vi "Wavefront analysis Final.vi"() -> ()   [LabVIEW 2020]
uses:
  <vilib>/Utility/file.llb/Read Delimited Spreadsheet (DBL).vi
  <vilib>/Analysis/NI_AALPro.lvlib
  <vilib>/Analysis/2dsp.llb/2D Real FFT.vi
  <vilib>/Analysis/2dsp.llb/2D Inverse Real FFT.vi
panel:
  in  "Reference images":T1(tab)
  out "Idler ref":dbl[][](graph)=[[0.0, 0.0, 0.0, 0.0, 0.0, 0.0, 0.0, 0.0, 0.0, 0.0, 0.0, 0.0, 0.0, 0.0, 0.0, 0.0, 0.0, 0.0, 33.0, 33.0, 33.0, 38.0, 30.0, 41.0, 34.0, 38.0, 29.0, 26.0, 34.0, 37.0, 34.0, 39.0, 41.0, 39.0, 28.0, 51.0, 29.0, 46.0, 35.0, 0.0, 0.0, 0.0, 0.0, 0.0, 0.0, 0.0, 0.0, 0.0, 0.0, 0.0, 0.0, 0.0, 0.0, 0.0, 0.0, 0.0, 0.0, 0.0], [0.0, 0.0, 0.0, 0.0, 0.0, 0.0, 0.0, 0.0, 0.0, 0.0, 0.0, 0.0, 0.0, 0.0, 0.0, 29.0, 23.0, 38.0, 37.0, 31.0, 35.0, 38.0, 33.0, 31.0, 43.0, 36.0, 24.0, 41.0, 38.0, 33.0, 48.0, 34.0, 27.0, 37.0, 37.0, 47.0, 27.0, 30.0, 24.0, 36.0, 28.0, 40.0, 0.0, 0.0, 0.0, 0.0, 0.0, 0.0, 0.0, 0.0, 0.0, 0.0, 0.0, 0.0, 0.0, 0.0, 0.0, 0.0], [0.0, 0.0, 0.0, 0.0, 0.0, 0.0, 0.0, 0.0, 0.0, 0.0, 0.0, 0.0, 0.0, 0.0, 24.0, 28.0, 30.0, 32.0, 21.0, 38.0, 33.0, 37.0, 36.0, 39.0, 36.0, 20.0, 48.0, 45.0, 50.0, 36.0, 30.0, 33.0, 44.0, 34.0, 31.0, 41.0, 34.0, 34.0, 26.0, 38.0, 38.0, 33.0, 28.0, 0.0, 0.0, 0.0, 0.0, 0.0, 0.0, 0.0, 0.0, 0.0, 0.0, 0.0, 0.0, 0.0, 0.0, 0.0], [0.0, 0.0, 0.0, 0.0, 0.0, 0.0, 0.0, 0.0, 0.0, 0.0, 0.0, 0.0, 36.0, 33.0, 26.0, 25.0, 35.0, 38.0, 37.0, 24.0, 35.0, 37.0, 34.0, 35.0, 34.0, 35.0, 42.0, 33.0, 36.0, 33.0, 53.0, 50.0, 40.0, 36.0, 45.0, 27.0, 36.0, 44.0, 23.0, 29.0, 23.0, 31.0, 26.0, 22.0, 27.0, 0.0, 0.0, 0.0, 0.0, 0.0, 0.0, 0.0, 0.0, 0.0, 0.0, 0.0, 0.0, 0.0], [0.0, 0.0, 0.0, 0.0, 0.0, 0.0, 0.0, 0.0, 0.0, 0.0, 0.0, 27.0, 31.0, 42.0, 27.0, 39.0, 33.0, 23.0, 26.0, 41.0, 28.0, 46.0, 34.0, 36.0, 36.0, 37.0, 37.0, 51.0, 39.0, 51.0, 38.0, 40.0, 32.0, 43.0, 30.0, 48.0, 29.0, 27.0, 31.0, 50.0, 35.0, 31.0, 23.0, 18.0, 27.0, 26.0, 0.0, 0.0, 0.0, 0.0, 0.0, 0.0, 0.0, 0.0, 0.0, 0.0, 0.0, 0.0], [0.0, 0.0, 0.0, 0.0, 0.0, 0.0, 0.0, 0.0, 0.0, 26.0, 28.0, 24.0, 30.0, 32.0, 29.0, 36.0, 28.0, 42.0, 34.0, 34.0, 43.0, 42.0, 35.0, 40.0, 24.0, 47.0, 35.0, 40.0, 41.0, 44.0, 46.0, 46.0, 40.0, 33.0, 42.0, 38.0, 30.0, 35.0, 29.0, 30.0, 24.0, 42.0, 40.0, 27.0, 29.0, 36.0, 26.0, 60.0, 0.0, 0.0, 0.0, 0.0, 0.0, 0.0, 0.0, 0.0, 0.0, 0.0], [0.0, 0.0, 0.0, 0.0, 0.0, 0.0, 0.0, 0.0, 30.0, 36.0, 36.0, 25.0, 30.0, 38.0, 31.0, 37.0, 36.0, 30.0, 25.0, 34.0, 55.0, 21.0, 38.0, 55.0, 42.0, 46.0, 34.0, 53.0, 43.0, 36.0, 41.0, 44.0, 40.0, 35.0, 42.0, 42.0, 27.0, 38.0, 40.0, 40.0, 41.0, 35.0, 31.0, 37.0, 30.0, 36.0, 39.0, 38.0, 25.0, 0.0, 0.0, 0.0, 0.0, 0.0, 0.0, 0.0, 0.0, 0.0], [0.0, 0.0, 0.0, 0.0, 0.0, 0.0, 0.0, 32.0, 34.0, 29.0, 26.0, 28.0, 35.0, 32.0, 27.0, 32.0, 35.0, 40.0, 43.0, 41.0, 29.0, 52.0, 41.0, 55.0, 34.0, 45.0, 44.0, 53.0, 55.0, 45.0, 41.0, 50.0, 47.0, 49.0, 41.0, 53.0, 57.0, 39.0, 43.0, 51.0, 30.0, 45.0, 32.0, 32.0, 28.0, 39.0, 31.0, 39.0, 38.0, 29.0, 0.0, 0.0, 0.0, 0.0, 0.0, 0.0, 0.0, 0.0], [0.0, 0.0, 0.0, 0.0, 0.0, 0.0, 24.0, 28.0, 14.0, 26.0, 35.0, 26.0, 43.0, 27.0, 40.0, 51.0, 25.0, 39.0, 40.0, 35.0, 39.0, 43.0, 43.0, 63.0, 50.0, 55.0, 64.0, 56.0, 55.0, 58.0, 62.0, 49.0, 50.0, 53.0, 40.0, 53.0, 40.0, 32.0, 47.0, 48.0, 40.0, 31.0, 33.0, 41.0, 37.0, 41.0, 35.0, 38.0, 22.0, 43.0, 25.0, 0.0, 0.0, 0.0, 0.0, 0.0, 0.0, 0.0], [0.0, 0.0, 0.0, 0.0, 0.0, 30.0, 23.0, 38.0, 28.0, 28.0, 21.0, 17.0, 39.0, 32.0, 25.0, 30.0, 39.0, 43.0, 39.0, 40.0, 36.0, 49.0, 65.0, 63.0, 68.0, 68.0, 91.0, 134.0, 191.0, 218.0, 213.0, 162.0, 141.0, 99.0, 74.0, 61.0, 57.0, 50.0, 46.0, 43.0, 39.0, 44.0, 31.0, 41.0, 31.0, 31.0, 39.0, 39.0, 25.0, 47.0, 30.0, 39.0, 0.0, 0.0, 0.0, 0.0, 0.0, 0.0], [0.0, 0.0, 0.0, 0.0, 0.0, 25.0, 34.0, 32.0, 30.0, 30.0, 33.0, 38.0, 20.0, 38.0, 36.0, 38.0, 38.0, 37.0, 50.0, 56.0, 67.0, 82.0, 95.0, 151.0, 229.0, 345.0, 495.0, 498.0, 427.0, 526.0, 467.0, 540.0, 425.0, 358.0, 282.0, 162.0, 126.0, 88.0, 41.0, 56.0, 54.0, 29.0, 38.0, 24.0, 29.0, 41.0, 25.0, 34.0, 38.0, 37.0, 32.0, 28.0, 0.0, 0.0, 0.0, 0.0, 0.0, 0.0], [0.0, 0.0, 0.0, 0.0, 33.0, 23.0, 29.0, 28.0, 21.0, 34.0, 21.0, 31.0, 28.0, 32.0, 38.0, 48.0, 24.0, 44.0, 53.0, 80.0, 88.0, 241.0, 416.0, 503.0, 578.0, 542.0, 550.0, 501.0, 622.0, 490.0, 555.0, 528.0, 521.0, 522.0, 551.0, 513.0, 396.0, 306.0, 163.0, 65.0, 58.0, 47.0, 45.0, 36.0, 49.0, 37.0, 40.0, 21.0, 28.0, 43.0, 42.0, 29.0, 39.0, 0.0, 0.0, 0.0, 0.0, 0.0], [0.0, 0.0, 0.0, 26.0, 22.0, 31.0, 26.0, 26.0, 29.0, 21.0, 33.0, 39.0, 34.0, 32.0, 40.0, 54.0, 44.0, 50.0, 84.0, 130.0, 319.0, 562.0, 595.0, 590.0, 484.0, 448.0, 430.0, 508.0, 426.0, 495.0, 370.0, 486.0, 414.0, 422.0, 449.0, 546.0, 539.0, 454.0, 378.0, 228.0, 88.0, 48.0, 35.0, 46.0, 27.0, 38.0, 30.0, 45.0, 34.0, 31.0, 35.0, 26.0, 42.0, 27.0, 0.0, 0.0, 0.0, 0.0], [0.0, 0.0, 0.0, 28.0, 28.0, 24.0, 30.0, 21.0, 29.0, 30.0, 37.0, 28.0, 41.0, 47.0, 32.0, 40.0, 69.0, 72.0, 195.0, 471.0, 613.0, 548.0, 436.0, 452.0, 459.0, 526.0, 488.0, 652.0, 721.0, 779.0, 685.0, 563.0, 529.0, 568.0, 425.0, 399.0, 408.0, 519.0, 486.0, 494.0, 295.0, 138.0, 54.0, 59.0, 44.0, 40.0, 36.0, 35.0, 34.0, 36.0, 30.0, 26.0, 20.0, 37.0, 0.0, 0.0, 0.0, 0.0], [0.0, 0.0, 24.0, 26.0, 32.0, 27.0, 27.0, 34.0, 19.0, 40.0, 35.0, 33.0, 35.0, 33.0, 55.0, 71.0, 90.0, 231.0, 518.0, 543.0, 543.0, 410.0, 519.0, 562.0, 791.0, 1009.0, 1198.0, 1635.0, 1601.0, 1726.0, 1566.0, 1517.0, 1198.0, 1037.0, 729.0, 515.0, 464.0, 430.0, 429.0, 503.0, 406.0, 338.0, 122.0, 51.0, 36.0, 41.0, 39.0, 42.0, 44.0, 36.0, 26.0, 33.0, 21.0, 32.0, 35.0, 0.0, 0.0, 0.0], [0.0, 21.0, 22.0, 24.0, 27.0, 27.0, 27.0, 23.0, 26.0, 29.0, 17.0, 42.0, 42.0, 46.0, 52.0, 106.0, 346.0, 509.0, 575.0, 535.0, 497.0, 567.0, 866.0, 1318.0, 1774.0, 2119.0, 2964.0, 3113.0, 3455.0, 3111.0, 3488.0, 3069.0, 2628.0, 2285.0, 1622.0, 1099.0, 710.0, 556.0, 435.0, 484.0, 498.0, 519.0, 371.0, 150.0, 59.0, 55.0, 36.0, 36.0, 35.0, 31.0, 41.0, 39.0, 30.0, 30.0, 26.0, 33.0, 0.0, 0.0], [0.0, 32.0, 24.0, 27.0, 25.0, 21.0, 32.0, 31.0, 36.0, 25.0, 45.0, 44.0, 58.0, 64.0, 65.0, 377.0, 581.0, 632.0, 457.0, 563.0, 675.0, 1158.0, 1641.0, 2438.0, 3581.0, 4509.0, 4776.0, 5330.0, 5944.0, 6860.0, 6038.0, 5448.0, 4841.0, 3697.0, 3073.0, 2359.0, 1544.0, 971.0, 576.0, 432.0, 386.0, 564.0, 475.0, 342.0, 118.0, 59.0, 45.0, 35.0, 43.0, 44.0, 32.0, 37.0, 43.0, 36.0, 27.0, 26.0, 0.0, 0.0], [0.0, 23.0, 16.0, 31.0, 22.0, 30.0, 32.0, 31.0, 35.0, 38.0, 40.0, 41.0, 52.0, 74.0, 176.0, 530.0, 531.0, 542.0, 517.0, 741.0, 1312.0, 1994.0, 3477.0, 4643.0, 5314.0, 6802.0, 7334.0, 7358.0, 8098.0, 7575.0, 8057.0, 7131.0, 6266.0, 6447.0, 4971.0, 4459.0, 2925.0, 2009.0, 1242.0, 643.0, 485.0, 441.0, 476.0, 478.0, 230.0, 121.0, 43.0, 35.0, 47.0, 37.0, 34.0, 26.0, 30.0, 43.0, 35.0, 38.0, 0.0, 0.0], [22.0, 14.0, 27.0, 31.0, 29.0, 36.0, 22.0, 29.0, 30.0, 32.0, 33.0, 37.0, 56.0, 104.0, 425.0, 632.0, 524.0, 490.0, 697.0, 1430.0, 2375.0, 3795.0, 4959.0, 7130.0, 7177.0, 7810.0, 8567.0, 10207.0, 9049.0, 9189.0, 8739.0, 9440.0, 8494.0, 7912.0, 7186.0, 5411.0, 4928.0, 3224.0, 2005.0, 1126.0, 613.0, 437.0, 411.0, 580.0, 384.0, 187.0, 76.0, 46.0, 32.0, 35.0, 42.0, 36.0, 33.0, 29.0, 23.0, 30.0, 26.0, 0.0], [20.0, 24.0, 22.0, 19.0, 30.0, 24.0, 32.0, 40.0, 41.0, 42.0, 40.0, 52.0, 68.0, 232.0, 602.0, 525.0, 564.0, 695.0, 1240.0, 2185.0, 3656.0, 5311.0, 4998.0, 9311.0, 9246.0, 11117.0, 9926.0, 10643.0, 9993.0, 10412.0, 10979.0, 10696.0, 10376.0, 9054.0, 8507.0, 7575.0, 5940.0, 4773.0, 3361.0, 1780.0, 1166.0, 531.0, 411.0, 468.0, 491.0, 311.0, 113.0, 56.0, 40.0, 39.0, 26.0, 35.0, 31.0, 34.0, 29.0, 26.0, 33.0, 0.0], [24.0, 23.0, 25.0, 31.0, 36.0, 20.0, 41.0, 28.0, 47.0, 25.0, 38.0, 71.0, 119.0, 408.0, 589.0, 505.0, 529.0, 1018.0, 2193.0, 3424.0, 5249.0, 6870.0, 12486.0, 7988.0, 10335.0, 10971.0, 11179.0, 10325.0, 11253.0, 11504.0, 10668.0, 9355.0, 12095.0, 9948.0, 10038.0, 9773.0, 8219.0, 6509.0, 4643.0, 3116.0, 1708.0, 893.0, 415.0, 381.0, 491.0, 398.0, 157.0, 68.0, 43.0, 43.0, 34.0, 34.0, 27.0, 24.0, 26.0, 40.0, 29.0, 0.0], [25.0, 31.0, 29.0, 24.0, 25.0, 21.0, 29.0, 30.0, 36.0, 32.0, 57.0, 71.0, 172.0, 601.0, 502.0, 557.0, 739.0, 1605.0, 2981.0, 4696.0, 6564.0, 7940.0, 9108.0, 9805.0, 12772.0, 10382.0, 10614.0, 11851.0, 11619.0, 9702.0, 11860.0, 11185.0, 12321.0, 10842.0, 11020.0, 9818.0, 8451.0, 8122.0, 5936.0, 4325.0, 2629.0, 1259.0, 627.0, 413.0, 407.0, 538.0, 227.0, 107.0, 49.0, 33.0, 39.0, 35.0, 26.0, 33.0, 31.0, 43.0, 21.0, 32.0], [28.0, 27.0, 31.0, 31.0, 21.0, 35.0, 25.0, 32.0, 21.0, 42.0, 61.0, 95.0, 378.0, 589.0, 538.0, 547.0, 975.0, 2235.0, 3482.0, 6571.0, 8268.0, 9056.0, 11003.0, 11631.0, 10641.0, 11928.0, 10949.0, 10324.0, 10096.0, 11159.0, 10977.0, 10308.0, 10593.0, 10623.0, 10514.0, 11646.0, 9405.0, 9366.0, 7021.0, 5020.0, 3319.0, 1720.0, 806.0, 455.0, 421.0, 467.0, 345.0, 132.0, 54.0, 34.0, 37.0, 37.0, 34.0, 27.0, 33.0, 20.0, 37.0, 34.0], [19.0, 18.0, 18.0, 23.0, 27.0, 34.0, 28.0, 31.0, 50.0, 42.0, 65.0, 182.0, 477.0, 528.0, 524.0, 691.0, 1719.0, 2864.0, 5291.0, 6825.0, 8333.0, 11756.0, 10344.0, 10804.0, 11046.0, 11765.0, 10495.0, 9731.0, 10459.0, 9842.0, 9930.0, 11113.0, 10964.0, 10430.0, 11969.0, 10333.0, 10266.0, 9385.0, 8245.0, 6496.0, 4192.0, 2630.0, 1143.0, 511.0, 400.0, 488.0, 448.0, 150.0, 70.0, 64.0, 42.0, 47.0, 34.0, 28.0, 33.0, 40.0, 13.0, 29.0], [21.0, 21.0, 24.0, 24.0, 27.0, 29.0, 24.0, 29.0, 46.0, 60.0, 76.0, 211.0, 501.0, 550.0, 555.0, 854.0, 1737.0, 3504.0, 6034.0, 8184.0, 8996.0, 11258.0, 10863.0, 12142.0, 11259.0, 10331.0, 10193.0, 9997.0, 10594.0, 8854.0, 10112.0, 9586.0, 10297.0, 11180.0, 10510.0, 10948.0, 10675.0, 10412.0, 8729.0, 6607.0, 5134.0, 3360.0, 1427.0, 586.0, 372.0, 479.0, 399.0, 286.0, 89.0, 51.0, 29.0, 30.0, 37.0, 32.0, 22.0, 31.0, 26.0, 37.0], [25.0, 27.0, 34.0, 27.0, 24.0, 28.0, 24.0, 36.0, 30.0, 53.0, 85.0, 319.0, 584.0, 600.0, 481.0, 1091.0, 2479.0, 4389.0, 6310.0, 9581.0, 9832.0, 10928.0, 11595.0, 11202.0, 11015.0, 10084.0, 9684.0, 9403.0, 7350.0, 9729.0, 8597.0, 10018.0, 9495.0, 10362.0, 10919.0, 10975.0, 10297.0, 10217.0, 9438.0, 7555.0, 5604.0, 3235.0, 1775.0, 800.0, 424.0, 481.0, 434.0, 294.0, 121.0, 48.0, 34.0, 37.0, 26.0, 35.0, 36.0, 25.0, 36.0, 33.0], [29.0, 21.0, 18.0, 24.0, 35.0, 21.0, 25.0, 37.0, 45.0, 52.0, 87.0, 334.0, 584.0, 473.0, 565.0, 1252.0, 2463.0, 4773.0, 6636.0, 8697.0, 11429.0, 10731.0, 10391.0, 11230.0, 10171.0, 9829.0, 9358.0, 9183.0, 9445.0, 8181.0, 9165.0, 8709.0, 8839.0, 10359.0, 10801.0, 9836.0, 10995.0, 10816.0, 10069.0, 7534.0, 5988.0, 3951.0, 1933.0, 952.0, 401.0, 448.0, 450.0, 343.0, 99.0, 57.0, 42.0, 36.0, 36.0, 38.0, 38.0, 37.0, 22.0, 40.0], [33.0, 35.0, 24.0, 27.0, 24.0, 26.0, 32.0, 30.0, 42.0, 65.0, 71.0, 328.0, 607.0, 516.0, 605.0, 1220.0, 2764.0, 5060.0, 7173.0, 9574.0, 9796.0, 11663.0, 10720.0, 12846.0, 9527.0, 10609.0, 8504.0, 9578.0, 8651.0, 8801.0, 7431.0, 8853.0, 9445.0, 9729.0, 10227.0, 11834.0, 10672.0, 10151.0, 9726.0, 8997.0, 6241.0, 4204.0, 2261.0, 870.0, 495.0, 443.0, 510.0, 339.0, 103.0, 64.0, 34.0, 33.0, 25.0, 41.0, 21.0, 21.0, 22.0, 31.0], [18.0, 23.0, 26.0, 26.0, 26.0, 42.0, 29.0, 42.0, 40.0, 57.0, 79.0, 370.0, 532.0, 574.0, 568.0, 1438.0, 2860.0, 5302.0, 7498.0, 9651.0, 9680.0, 11035.0, 11621.0, 10274.0, 9812.0, 10930.0, 8870.0, 9508.0, 7597.0, 8953.0, 8701.0, 9464.0, 8784.0, 10769.0, 9489.0, 11215.0, 10422.0, 10977.0, 8756.0, 8755.0, 5647.0, 4844.0, 2058.0, 1048.0, 428.0, 413.0, 465.0, 364.0, 127.0, 56.0, 38.0, 32.0, 32.0, 26.0, 26.0, 28.0, 26.0, 33.0], [22.0, 17.0, 26.0, 31.0, 26.0, 25.0, 23.0, 24.0, 35.0, 58.0, 99.0, 316.0, 630.0, 597.0, 550.0, 1361.0, 2643.0, 4687.0, 6930.0, 8844.0, 9908.0, 11137.0, 10461.0, 12016.0, 11124.0, 8758.0, 9497.0, 8959.0, 8403.0, 8907.0, 7968.0, 9479.0, 7817.0, 11878.0, 10209.0, 11642.0, 10825.0, 10586.0, 9688.0, 8819.0, 6405.0, 4123.0, 2208.0, 951.0, 432.0, 510.0, 416.0, 317.0, 98.0, 47.0, 30.0, 36.0, 34.0, 27.0, 30.0, 27.0, 28.0, 34.0], [20.0, 20.0, 31.0, 13.0, 23.0, 26.0, 38.0, 41.0, 43.0, 51.0, 59.0, 372.0, 566.0, 550.0, 547.0, 1163.0, 2273.0, 4811.0, 6481.0, 9604.0, 10290.0, 11230.0, 10872.0, 10070.0, 10565.0, 10873.0, 9490.0, 9608.0, 8858.0, 8698.0, 9740.0, 9255.0, 9585.0, 10318.0, 10549.0, 10201.0, 10721.0, 11495.0, 8466.0, 8079.0, 5681.0, 4016.0, 2129.0, 962.0, 427.0, 445.0, 393.0, 332.0, 116.0, 55.0, 32.0, 41.0, 30.0, 34.0, 34.0, 33.0, 27.0, 27.0], [16.0, 38.0, 26.0, 34.0, 22.0, 38.0, 27.0, 27.0, 44.0, 59.0, 66.0, 324.0, 585.0, 605.0, 505.0, 1057.0, 2197.0, 4221.0, 5855.0, 8610.0, 9564.0, 11505.0, 9789.0, 12674.0, 9997.0, 11264.0, 9528.0, 10363.0, 9151.0, 9507.0, 8605.0, 10215.0, 10311.0, 10253.0, 10901.0, 12845.0, 10351.0, 10239.0, 9807.0, 7870.0, 5582.0, 3329.0, 1717.0, 853.0, 371.0, 460.0, 440.0, 288.0, 102.0, 43.0, 34.0, 30.0, 41.0, 33.0, 19.0, 23.0, 27.0, 30.0], [16.0, 15.0, 12.0, 18.0, 32.0, 30.0, 18.0, 29.0, 48.0, 50.0, 68.0, 235.0, 544.0, 581.0, 577.0, 892.0, 1622.0, 3969.0, 6014.0, 7901.0, 9519.0, 11253.0, 10036.0, 12070.0, 10805.0, 10642.0, 10593.0, 10784.0, 9506.0, 11212.0, 9785.0, 11127.0, 10100.0, 12230.0, 10694.0, 10737.0, 12054.0, 11072.0, 8620.0, 7469.0, 4757.0, 3066.0, 1367.0, 495.0, 428.0, 498.0, 377.0, 256.0, 76.0, 53.0, 35.0, 30.0, 33.0, 37.0, 23.0, 44.0, 27.0, 31.0], [24.0, 31.0, 27.0, 15.0, 21.0, 30.0, 30.0, 36.0, 31.0, 49.0, 55.0, 145.0, 504.0, 573.0, 495.0, 620.0, 1607.0, 2733.0, 4655.0, 7794.0, 7507.0, 10585.0, 11470.0, 10295.0, 11512.0, 11444.0, 11207.0, 10982.0, 10269.0, 11393.0, 9225.0, 11186.0, 10890.0, 10763.0, 11164.0, 11732.0, 10195.0, 9714.0, 7731.0, 6073.0, 3965.0, 2203.0, 963.0, 560.0, 388.0, 443.0, 362.0, 245.0, 78.0, 54.0, 41.0, 25.0, 27.0, 36.0, 27.0, 22.0, 19.0, 24.0], [17.0, 23.0, 22.0, 27.0, 23.0, 25.0, 28.0, 27.0, 37.0, 59.0, 52.0, 86.0, 369.0, 616.0, 524.0, 613.0, 922.0, 2172.0, 3677.0, 5932.0, 8236.0, 9587.0, 10519.0, 11994.0, 11385.0, 12455.0, 11490.0, 11569.0, 9786.0, 12618.0, 10807.0, 11378.0, 10102.0, 11687.0, 11262.0, 11813.0, 9709.0, 9646.0, 6898.0, 5553.0, 3092.0, 1903.0, 712.0, 463.0, 401.0, 514.0, 366.0, 107.0, 61.0, 45.0, 31.0, 25.0, 19.0, 23.0, 24.0, 30.0, 32.0, 31.0], [35.0, 20.0, 25.0, 23.0, 25.0, 24.0, 28.0, 25.0, 38.0, 50.0, 59.0, 73.0, 172.0, 520.0, 567.0, 524.0, 809.0, 1769.0, 2680.0, 4518.0, 6192.0, 8250.0, 9723.0, 10511.0, 9553.0, 10974.0, 11124.0, 11651.0, 11831.0, 10824.0, 10850.0, 10868.0, 10452.0, 12044.0, 10795.0, 9860.0, 8964.0, 7809.0, 5547.0, 4172.0, 2266.0, 1037.0, 501.0, 427.0, 452.0, 473.0, 207.0, 97.0, 38.0, 35.0, 40.0, 41.0, 26.0, 38.0, 32.0, 23.0, 20.0, 29.0], [24.0, 25.0, 20.0, 28.0, 26.0, 23.0, 37.0, 36.0, 37.0, 39.0, 64.0, 63.0, 104.0, 418.0, 611.0, 593.0, 561.0, 1071.0, 1871.0, 4080.0, 4588.0, 7458.0, 7802.0, 9977.0, 10579.0, 10430.0, 10760.0, 11288.0, 10234.0, 12567.0, 10198.0, 11758.0, 10670.0, 11137.0, 9421.0, 9271.0, 7021.0, 6943.0, 3874.0, 2970.0, 1411.0, 812.0, 352.0, 444.0, 456.0, 394.0, 165.0, 59.0, 37.0, 30.0, 22.0, 31.0, 28.0, 27.0, 29.0, 28.0, 26.0, 0.0], [21.0, 24.0, 24.0, 25.0, 28.0, 29.0, 25.0, 44.0, 52.0, 45.0, 64.0, 76.0, 99.0, 215.0, 567.0, 577.0, 493.0, 697.0, 1111.0, 2039.0, 3142.0, 5007.0, 5918.0, 8639.0, 7955.0, 10544.0, 9986.0, 10767.0, 10437.0, 10532.0, 9905.0, 10126.0, 9204.0, 9729.0, 8888.0, 7806.0, 5715.0, 5184.0, 3167.0, 1756.0, 788.0, 560.0, 399.0, 480.0, 498.0, 250.0, 83.0, 56.0, 26.0, 34.0, 23.0, 29.0, 18.0, 27.0, 24.0, 27.0, 30.0, 0.0], [26.0, 22.0, 23.0, 23.0, 29.0, 34.0, 34.0, 46.0, 37.0, 48.0, 46.0, 74.0, 72.0, 128.0, 392.0, 639.0, 595.0, 512.0, 661.0, 1409.0, 2136.0, 3870.0, 4979.0, 5905.0, 6955.0, 8199.0, 8335.0, 8836.0, 8999.0, 9055.0, 8382.0, 9320.0, 8041.0, 8419.0, 6068.0, 5857.0, 4121.0, 2936.0, 1819.0, 994.0, 519.0, 404.0, 419.0, 507.0, 343.0, 164.0, 51.0, 55.0, 37.0, 29.0, 27.0, 20.0, 27.0, 22.0, 19.0, 24.0, 23.0, 0.0], [0.0, 22.0, 32.0, 27.0, 29.0, 33.0, 51.0, 25.0, 56.0, 48.0, 50.0, 63.0, 66.0, 102.0, 178.0, 575.0, 615.0, 596.0, 546.0, 708.0, 1087.0, 1959.0, 2831.0, 4292.0, 4826.0, 5620.0, 6566.0, 7177.0, 7116.0, 7486.0, 7108.0, 6801.0, 6665.0, 5350.0, 4676.0, 4161.0, 2937.0, 1656.0, 958.0, 611.0, 447.0, 466.0, 490.0, 468.0, 210.0, 88.0, 41.0, 49.0, 33.0, 43.0, 25.0, 35.0, 36.0, 26.0, 18.0, 21.0, 0.0, 0.0], [0.0, 20.0, 31.0, 31.0, 27.0, 34.0, 39.0, 57.0, 67.0, 56.0, 56.0, 60.0, 43.0, 73.0, 100.0, 256.0, 550.0, 593.0, 507.0, 507.0, 711.0, 1045.0, 1493.0, 2398.0, 2932.0, 4019.0, 4055.0, 5382.0, 4901.0, 5001.0, 5674.0, 5081.0, 3871.0, 4132.0, 2946.0, 1977.0, 1153.0, 918.0, 458.0, 391.0, 442.0, 540.0, 456.0, 291.0, 145.0, 59.0, 32.0, 35.0, 36.0, 35.0, 26.0, 22.0, 29.0, 19.0, 28.0, 28.0, 0.0, 0.0], [0.0, 28.0, 27.0, 32.0, 36.0, 34.0, 44.0, 41.0, 48.0, 58.0, 66.0, 55.0, 55.0, 54.0, 91.0, 102.0, 250.0, 571.0, 552.0, 494.0, 500.0, 556.0, 685.0, 1115.0, 1507.0, 2296.0, 2160.0, 3075.0, 2945.0, 3083.0, 2646.0, 2552.0, 2134.0, 2121.0, 1312.0, 1011.0, 629.0, 500.0, 395.0, 525.0, 514.0, 517.0, 306.0, 128.0, 63.0, 48.0, 28.0, 29.0, 22.0, 31.0, 25.0, 25.0, 19.0, 35.0, 23.0, 28.0, 0.0, 0.0], [0.0, 0.0, 38.0, 29.0, 31.0, 41.0, 43.0, 47.0, 41.0, 55.0, 64.0, 52.0, 66.0, 61.0, 70.0, 82.0, 146.0, 261.0, 506.0, 681.0, 570.0, 516.0, 465.0, 629.0, 707.0, 810.0, 1030.0, 1195.0, 1313.0, 1485.0, 1376.0, 1280.0, 1040.0, 835.0, 578.0, 487.0, 389.0, 416.0, 520.0, 504.0, 444.0, 273.0, 105.0, 82.0, 33.0, 36.0, 37.0, 36.0, 32.0, 20.0, 26.0, 36.0, 17.0, 26.0, 19.0, 0.0, 0.0, 0.0], [0.0, 0.0, 0.0, 40.0, 42.0, 35.0, 46.0, 41.0, 36.0, 56.0, 54.0, 63.0, 61.0, 50.0, 74.0, 75.0, 82.0, 107.0, 207.0, 465.0, 561.0, 647.0, 475.0, 444.0, 436.0, 517.0, 535.0, 560.0, 613.0, 674.0, 563.0, 591.0, 485.0, 467.0, 419.0, 442.0, 487.0, 576.0, 489.0, 438.0, 259.0, 127.0, 48.0, 38.0, 33.0, 31.0, 35.0, 31.0, 29.0, 29.0, 18.0, 36.0, 20.0, 22.0, 0.0, 0.0, 0.0, 0.0], [0.0, 0.0, 0.0, 31.0, 26.0, 40.0, 45.0, 40.0, 42.0, 56.0, 47.0, 43.0, 44.0, 70.0, 60.0, 66.0, 75.0, 71.0, 108.0, 130.0, 342.0, 563.0, 585.0, 561.0, 538.0, 523.0, 460.0, 479.0, 441.0, 384.0, 463.0, 437.0, 411.0, 476.0, 465.0, 609.0, 551.0, 529.0, 356.0, 192.0, 69.0, 45.0, 35.0, 48.0, 24.0, 24.0, 38.0, 27.0, 23.0, 25.0, 26.0, 23.0, 26.0, 23.0, 0.0, 0.0, 0.0, 0.0], [0.0, 0.0, 0.0, 0.0, 42.0, 55.0, 45.0, 47.0, 52.0, 38.0, 44.0, 52.0, 39.0, 59.0, 62.0, 61.0, 63.0, 63.0, 88.0, 97.0, 93.0, 223.0, 410.0, 517.0, 556.0, 602.0, 567.0, 594.0, 533.0, 602.0, 514.0, 624.0, 619.0, 596.0, 465.0, 473.0, 389.0, 230.0, 108.0, 68.0, 47.0, 38.0, 40.0, 40.0, 29.0, 28.0, 32.0, 23.0, 23.0, 32.0, 30.0, 19.0, 29.0, 0.0, 0.0, 0.0, 0.0, 0.0], [0.0, 0.0, 0.0, 0.0, 0.0, 40.0, 52.0, 44.0, 53.0, 40.0, 55.0, 52.0, 45.0, 55.0, 49.0, 58.0, 69.0, 55.0, 77.0, 59.0, 83.0, 109.0, 111.0, 139.0, 205.0, 362.0, 381.0, 536.0, 455.0, 495.0, 450.0, 439.0, 447.0, 353.0, 263.0, 134.0, 75.0, 77.0, 65.0, 60.0, 37.0, 35.0, 25.0, 22.0, 29.0, 35.0, 25.0, 24.0, 22.0, 27.0, 22.0, 36.0, 0.0, 0.0, 0.0, 0.0, 0.0, 0.0], [0.0, 0.0, 0.0, 0.0, 0.0, 44.0, 47.0, 55.0, 62.0, 51.0, 30.0, 40.0, 55.0, 52.0, 43.0, 56.0, 42.0, 64.0, 53.0, 69.0, 67.0, 66.0, 88.0, 86.0, 90.0, 90.0, 102.0, 127.0, 152.0, 236.0, 192.0, 140.0, 85.0, 79.0, 54.0, 53.0, 46.0, 51.0, 43.0, 32.0, 32.0, 26.0, 27.0, 15.0, 21.0, 30.0, 38.0, 22.0, 29.0, 19.0, 26.0, 15.0, 0.0, 0.0, 0.0, 0.0, 0.0, 0.0], [0.0, 0.0, 0.0, 0.0, 0.0, 0.0, 36.0, 33.0, 44.0, 49.0, 39.0, 45.0, 52.0, 48.0, 51.0, 50.0, 53.0, 51.0, 61.0, 75.0, 53.0, 76.0, 55.0, 55.0, 47.0, 77.0, 83.0, 73.0, 62.0, 58.0, 66.0, 51.0, 42.0, 48.0, 65.0, 34.0, 30.0, 49.0, 28.0, 37.0, 24.0, 35.0, 21.0, 20.0, 25.0, 30.0, 14.0, 33.0, 27.0, 20.0, 18.0, 0.0, 0.0, 0.0, 0.0, 0.0, 0.0, 0.0], [0.0, 0.0, 0.0, 0.0, 0.0, 0.0, 0.0, 45.0, 42.0, 58.0, 55.0, 66.0, 47.0, 42.0, 45.0, 37.0, 40.0, 64.0, 48.0, 48.0, 52.0, 47.0, 62.0, 50.0, 72.0, 32.0, 69.0, 48.0, 49.0, 40.0, 52.0, 51.0, 36.0, 42.0, 43.0, 29.0, 40.0, 35.0, 34.0, 35.0, 25.0, 18.0, 20.0, 24.0, 22.0, 19.0, 21.0, 20.0, 18.0, 23.0, 0.0, 0.0, 0.0, 0.0, 0.0, 0.0, 0.0, 0.0], [0.0, 0.0, 0.0, 0.0, 0.0, 0.0, 0.0, 0.0, 42.0, 43.0, 42.0, 36.0, 46.0, 42.0, 32.0, 56.0, 45.0, 54.0, 51.0, 43.0, 70.0, 56.0, 59.0, 50.0, 50.0, 54.0, 38.0, 32.0, 41.0, 45.0, 40.0, 36.0, 38.0, 48.0, 30.0, 30.0, 33.0, 35.0, 27.0, 31.0, 24.0, 26.0, 26.0, 29.0, 14.0, 24.0, 21.0, 23.0, 15.0, 0.0, 0.0, 0.0, 0.0, 0.0, 0.0, 0.0, 0.0, 0.0], [0.0, 0.0, 0.0, 0.0, 0.0, 0.0, 0.0, 0.0, 0.0, 42.0, 35.0, 52.0, 46.0, 49.0, 76.0, 38.0, 51.0, 42.0, 47.0, 51.0, 47.0, 52.0, 43.0, 61.0, 51.0, 48.0, 40.0, 38.0, 35.0, 40.0, 33.0, 36.0, 33.0, 31.0, 23.0, 24.0, 25.0, 34.0, 25.0, 20.0, 32.0, 25.0, 23.0, 23.0, 15.0, 34.0, 22.0, 27.0, 0.0, 0.0, 0.0, 0.0, 0.0, 0.0, 0.0, 0.0, 0.0, 0.0], [0.0, 0.0, 0.0, 0.0, 0.0, 0.0, 0.0, 0.0, 0.0, 0.0, 0.0, 39.0, 58.0, 43.0, 36.0, 51.0, 42.0, 53.0, 48.0, 42.0, 56.0, 35.0, 41.0, 43.0, 33.0, 42.0, 31.0, 32.0, 34.0, 36.0, 31.0, 27.0, 35.0, 31.0, 25.0, 37.0, 27.0, 26.0, 24.0, 30.0, 22.0, 32.0, 22.0, 19.0, 20.0, 17.0, 0.0, 0.0, 0.0, 0.0, 0.0, 0.0, 0.0, 0.0, 0.0, 0.0, 0.0, 0.0], [0.0, 0.0, 0.0, 0.0, 0.0, 0.0, 0.0, 0.0, 0.0, 0.0, 0.0, 0.0, 49.0, 36.0, 49.0, 46.0, 38.0, 45.0, 43.0, 45.0, 55.0, 53.0, 47.0, 46.0, 37.0, 41.0, 36.0, 45.0, 33.0, 35.0, 29.0, 34.0, 27.0, 33.0, 27.0, 27.0, 24.0, 34.0, 13.0, 27.0, 22.0, 30.0, 27.0, 16.0, 23.0, 0.0, 0.0, 0.0, 0.0, 0.0, 0.0, 0.0, 0.0, 0.0, 0.0, 0.0, 0.0, 0.0], [0.0, 0.0, 0.0, 0.0, 0.0, 0.0, 0.0, 0.0, 0.0, 0.0, 0.0, 0.0, 0.0, 0.0, 51.0, 53.0, 53.0, 47.0, 44.0, 48.0, 30.0, 39.0, 31.0, 49.0, 34.0, 28.0, 45.0, 22.0, 38.0, 30.0, 30.0, 30.0, 30.0, 16.0, 33.0, 22.0, 30.0, 28.0, 26.0, 25.0, 15.0, 32.0, 28.0, 0.0, 0.0, 0.0, 0.0, 0.0, 0.0, 0.0, 0.0, 0.0, 0.0, 0.0, 0.0, 0.0, 0.0, 0.0], [0.0, 0.0, 0.0, 0.0, 0.0, 0.0, 0.0, 0.0, 0.0, 0.0, 0.0, 0.0, 0.0, 0.0, 0.0, 42.0, 52.0, 47.0, 41.0, 40.0, 49.0, 44.0, 44.0, 25.0, 39.0, 43.0, 30.0, 32.0, 37.0, 31.0, 29.0, 35.0, 28.0, 38.0, 16.0, 28.0, 32.0, 22.0, 35.0, 18.0, 24.0, 26.0, 0.0, 0.0, 0.0, 0.0, 0.0, 0.0, 0.0, 0.0, 0.0, 0.0, 0.0, 0.0, 0.0, 0.0, 0.0, 0.0], [0.0, 0.0, 0.0, 0.0, 0.0, 0.0, 0.0, 0.0, 0.0, 0.0, 0.0, 0.0, 0.0, 0.0, 0.0, 0.0, 0.0, 0.0, 49.0, 46.0, 40.0, 32.0, 28.0, 38.0, 34.0, 29.0, 31.0, 23.0, 34.0, 30.0, 25.0, 32.0, 28.0, 28.0, 25.0, 23.0, 27.0, 29.0, 23.0, 0.0, 0.0, 0.0, 0.0, 0.0, 0.0, 0.0, 0.0, 0.0, 0.0, 0.0, 0.0, 0.0, 0.0, 0.0, 0.0, 0.0, 0.0, 0.0], [0.0, 0.0, 0.0, 0.0, 0.0, 0.0, 0.0, 0.0, 0.0, 0.0, 0.0, 0.0, 0.0, 0.0, 0.0, 0.0, 0.0, 0.0, 0.0, 0.0, 0.0, 43.0, 35.0, 33.0, 34.0, 26.0, 29.0, 22.0, 28.0, 30.0, 29.0, 34.0, 27.0, 38.0, 20.0, 22.0, 0.0, 0.0, 0.0, 0.0, 0.0, 0.0, 0.0, 0.0, 0.0, 0.0, 0.0, 0.0, 0.0, 0.0, 0.0, 0.0, 0.0, 0.0, 0.0, 0.0, 0.0, 0.0]]
  out "Signal ref":dbl[][](graph)
  out "Idler Bck fer":dbl[][](graph)=[[0.0, 0.0, 0.0, 0.0, 0.0, 0.0, 0.0, 0.0, 0.0, 0.0, 0.0, 0.0, 0.0, 0.0, 0.0, 0.0, 0.0, 0.0, 30.0, 43.0, 31.0, 27.0, 24.0, 24.0, 33.0, 34.0, 40.0, 44.0, 26.0, 28.0, 24.0, 30.0, 32.0, 44.0, 24.0, 27.0, 32.0, 32.0, 28.0, 0.0, 0.0, 0.0, 0.0, 0.0, 0.0, 0.0, 0.0, 0.0, 0.0, 0.0, 0.0, 0.0, 0.0, 0.0, 0.0, 0.0, 0.0, 0.0], [0.0, 0.0, 0.0, 0.0, 0.0, 0.0, 0.0, 0.0, 0.0, 0.0, 0.0, 0.0, 0.0, 0.0, 0.0, 33.0, 24.0, 25.0, 29.0, 16.0, 31.0, 32.0, 24.0, 33.0, 37.0, 32.0, 18.0, 33.0, 18.0, 34.0, 27.0, 25.0, 28.0, 42.0, 23.0, 22.0, 23.0, 25.0, 32.0, 30.0, 18.0, 25.0, 0.0, 0.0, 0.0, 0.0, 0.0, 0.0, 0.0, 0.0, 0.0, 0.0, 0.0, 0.0, 0.0, 0.0, 0.0, 0.0], [0.0, 0.0, 0.0, 0.0, 0.0, 0.0, 0.0, 0.0, 0.0, 0.0, 0.0, 0.0, 0.0, 0.0, 29.0, 30.0, 25.0, 32.0, 20.0, 38.0, 31.0, 35.0, 24.0, 38.0, 27.0, 25.0, 36.0, 26.0, 45.0, 37.0, 40.0, 27.0, 45.0, 21.0, 36.0, 37.0, 28.0, 22.0, 38.0, 28.0, 31.0, 35.0, 32.0, 0.0, 0.0, 0.0, 0.0, 0.0, 0.0, 0.0, 0.0, 0.0, 0.0, 0.0, 0.0, 0.0, 0.0, 0.0], [0.0, 0.0, 0.0, 0.0, 0.0, 0.0, 0.0, 0.0, 0.0, 0.0, 0.0, 0.0, 24.0, 33.0, 37.0, 20.0, 30.0, 33.0, 24.0, 16.0, 24.0, 31.0, 29.0, 23.0, 28.0, 28.0, 22.0, 20.0, 28.0, 36.0, 24.0, 42.0, 24.0, 27.0, 32.0, 28.0, 31.0, 42.0, 23.0, 42.0, 29.0, 38.0, 29.0, 38.0, 23.0, 0.0, 0.0, 0.0, 0.0, 0.0, 0.0, 0.0, 0.0, 0.0, 0.0, 0.0, 0.0, 0.0], [0.0, 0.0, 0.0, 0.0, 0.0, 0.0, 0.0, 0.0, 0.0, 0.0, 0.0, 36.0, 22.0, 33.0, 32.0, 22.0, 23.0, 27.0, 29.0, 26.0, 39.0, 27.0, 24.0, 27.0, 29.0, 37.0, 32.0, 38.0, 19.0, 37.0, 33.0, 25.0, 36.0, 30.0, 29.0, 31.0, 34.0, 37.0, 31.0, 28.0, 26.0, 38.0, 40.0, 33.0, 33.0, 17.0, 0.0, 0.0, 0.0, 0.0, 0.0, 0.0, 0.0, 0.0, 0.0, 0.0, 0.0, 0.0], [0.0, 0.0, 0.0, 0.0, 0.0, 0.0, 0.0, 0.0, 0.0, 22.0, 30.0, 19.0, 26.0, 29.0, 23.0, 23.0, 36.0, 23.0, 25.0, 22.0, 32.0, 34.0, 28.0, 33.0, 17.0, 28.0, 29.0, 40.0, 30.0, 37.0, 32.0, 27.0, 34.0, 31.0, 29.0, 24.0, 25.0, 13.0, 38.0, 34.0, 31.0, 24.0, 35.0, 36.0, 30.0, 39.0, 23.0, 35.0, 0.0, 0.0, 0.0, 0.0, 0.0, 0.0, 0.0, 0.0, 0.0, 0.0], [0.0, 0.0, 0.0, 0.0, 0.0, 0.0, 0.0, 0.0, 21.0, 39.0, 38.0, 30.0, 21.0, 24.0, 29.0, 29.0, 29.0, 29.0, 23.0, 47.0, 34.0, 21.0, 31.0, 32.0, 33.0, 33.0, 32.0, 30.0, 35.0, 39.0, 28.0, 38.0, 38.0, 37.0, 31.0, 30.0, 35.0, 37.0, 25.0, 28.0, 41.0, 27.0, 25.0, 29.0, 28.0, 35.0, 24.0, 22.0, 20.0, 0.0, 0.0, 0.0, 0.0, 0.0, 0.0, 0.0, 0.0, 0.0], [0.0, 0.0, 0.0, 0.0, 0.0, 0.0, 0.0, 25.0, 21.0, 34.0, 25.0, 24.0, 30.0, 32.0, 17.0, 32.0, 22.0, 40.0, 28.0, 22.0, 16.0, 34.0, 30.0, 33.0, 25.0, 42.0, 36.0, 35.0, 41.0, 44.0, 32.0, 37.0, 27.0, 41.0, 37.0, 41.0, 38.0, 30.0, 27.0, 38.0, 31.0, 24.0, 37.0, 36.0, 28.0, 41.0, 30.0, 38.0, 31.0, 26.0, 0.0, 0.0, 0.0, 0.0, 0.0, 0.0, 0.0, 0.0], [0.0, 0.0, 0.0, 0.0, 0.0, 0.0, 25.0, 25.0, 21.0, 32.0, 18.0, 23.0, 23.0, 30.0, 27.0, 35.0, 22.0, 24.0, 25.0, 42.0, 42.0, 33.0, 17.0, 30.0, 45.0, 36.0, 48.0, 37.0, 37.0, 45.0, 39.0, 31.0, 35.0, 33.0, 40.0, 36.0, 33.0, 31.0, 25.0, 19.0, 32.0, 26.0, 35.0, 37.0, 40.0, 34.0, 30.0, 35.0, 26.0, 31.0, 30.0, 0.0, 0.0, 0.0, 0.0, 0.0, 0.0, 0.0], [0.0, 0.0, 0.0, 0.0, 0.0, 22.0, 25.0, 26.0, 23.0, 33.0, 24.0, 27.0, 18.0, 29.0, 19.0, 28.0, 40.0, 39.0, 26.0, 31.0, 24.0, 38.0, 52.0, 40.0, 38.0, 36.0, 41.0, 71.0, 63.0, 90.0, 79.0, 78.0, 68.0, 61.0, 38.0, 37.0, 30.0, 54.0, 27.0, 29.0, 33.0, 36.0, 26.0, 40.0, 22.0, 40.0, 39.0, 33.0, 29.0, 37.0, 30.0, 22.0, 0.0, 0.0, 0.0, 0.0, 0.0, 0.0], [0.0, 0.0, 0.0, 0.0, 0.0, 25.0, 27.0, 25.0, 26.0, 21.0, 23.0, 23.0, 24.0, 36.0, 31.0, 33.0, 28.0, 21.0, 26.0, 32.0, 39.0, 45.0, 35.0, 62.0, 80.0, 130.0, 141.0, 164.0, 125.0, 156.0, 139.0, 148.0, 121.0, 121.0, 137.0, 93.0, 80.0, 72.0, 34.0, 42.0, 29.0, 31.0, 23.0, 23.0, 30.0, 46.0, 28.0, 38.0, 29.0, 30.0, 21.0, 31.0, 0.0, 0.0, 0.0, 0.0, 0.0, 0.0], [0.0, 0.0, 0.0, 0.0, 25.0, 25.0, 15.0, 28.0, 26.0, 26.0, 26.0, 31.0, 29.0, 36.0, 19.0, 38.0, 27.0, 28.0, 24.0, 40.0, 47.0, 70.0, 140.0, 143.0, 155.0, 162.0, 159.0, 163.0, 188.0, 160.0, 181.0, 165.0, 171.0, 150.0, 146.0, 131.0, 94.0, 139.0, 79.0, 51.0, 29.0, 32.0, 36.0, 27.0, 32.0, 29.0, 34.0, 28.0, 24.0, 31.0, 24.0, 31.0, 20.0, 0.0, 0.0, 0.0, 0.0, 0.0], [0.0, 0.0, 0.0, 28.0, 19.0, 35.0, 24.0, 22.0, 26.0, 18.0, 26.0, 31.0, 21.0, 27.0, 33.0, 25.0, 39.0, 29.0, 47.0, 39.0, 100.0, 146.0, 162.0, 161.0, 140.0, 148.0, 155.0, 193.0, 152.0, 201.0, 139.0, 170.0, 163.0, 124.0, 147.0, 151.0, 157.0, 137.0, 152.0, 123.0, 58.0, 36.0, 42.0, 35.0, 29.0, 33.0, 16.0, 43.0, 29.0, 33.0, 23.0, 27.0, 30.0, 20.0, 0.0, 0.0, 0.0, 0.0], [0.0, 0.0, 0.0, 26.0, 25.0, 31.0, 28.0, 27.0, 30.0, 25.0, 28.0, 22.0, 25.0, 41.0, 25.0, 34.0, 34.0, 46.0, 81.0, 135.0, 163.0, 170.0, 136.0, 166.0, 169.0, 192.0, 215.0, 238.0, 221.0, 225.0, 244.0, 226.0, 191.0, 182.0, 156.0, 145.0, 126.0, 165.0, 148.0, 147.0, 117.0, 81.0, 27.0, 32.0, 31.0, 34.0, 55.0, 27.0, 29.0, 29.0, 21.0, 26.0, 17.0, 29.0, 0.0, 0.0, 0.0, 0.0], [0.0, 0.0, 18.0, 21.0, 21.0, 25.0, 17.0, 32.0, 22.0, 34.0, 33.0, 35.0, 21.0, 25.0, 36.0, 38.0, 42.0, 79.0, 136.0, 154.0, 168.0, 153.0, 204.0, 197.0, 235.0, 291.0, 354.0, 419.0, 444.0, 404.0, 389.0, 445.0, 309.0, 314.0, 222.0, 166.0, 161.0, 162.0, 131.0, 143.0, 133.0, 117.0, 71.0, 47.0, 38.0, 26.0, 20.0, 32.0, 35.0, 33.0, 32.0, 27.0, 31.0, 21.0, 15.0, 0.0, 0.0, 0.0], [0.0, 25.0, 19.0, 33.0, 19.0, 24.0, 21.0, 31.0, 29.0, 30.0, 31.0, 25.0, 35.0, 20.0, 34.0, 59.0, 116.0, 151.0, 157.0, 168.0, 168.0, 203.0, 290.0, 397.0, 463.0, 516.0, 704.0, 737.0, 791.0, 747.0, 960.0, 748.0, 645.0, 521.0, 454.0, 312.0, 204.0, 195.0, 135.0, 157.0, 141.0, 120.0, 137.0, 84.0, 45.0, 32.0, 25.0, 28.0, 34.0, 32.0, 26.0, 29.0, 25.0, 26.0, 22.0, 31.0, 0.0, 0.0], [0.0, 17.0, 21.0, 31.0, 16.0, 21.0, 23.0, 24.0, 28.0, 19.0, 21.0, 27.0, 21.0, 34.0, 32.0, 118.0, 168.0, 185.0, 154.0, 177.0, 222.0, 332.0, 402.0, 631.0, 830.0, 981.0, 1023.0, 1143.0, 1299.0, 1566.0, 1389.0, 1193.0, 1034.0, 777.0, 648.0, 602.0, 409.0, 253.0, 172.0, 147.0, 109.0, 152.0, 125.0, 138.0, 85.0, 42.0, 39.0, 28.0, 33.0, 28.0, 41.0, 20.0, 24.0, 24.0, 20.0, 17.0, 0.0, 0.0], [0.0, 23.0, 16.0, 23.0, 23.0, 29.0, 25.0, 27.0, 24.0, 38.0, 30.0, 28.0, 19.0, 50.0, 74.0, 136.0, 153.0, 184.0, 186.0, 254.0, 353.0, 461.0, 807.0, 1037.0, 1180.0, 1334.0, 1540.0, 1519.0, 1716.0, 1599.0, 1774.0, 1516.0, 1329.0, 1492.0, 1073.0, 922.0, 677.0, 466.0, 339.0, 202.0, 151.0, 113.0, 121.0, 126.0, 94.0, 82.0, 37.0, 34.0, 32.0, 25.0, 26.0, 26.0, 20.0, 20.0, 21.0, 23.0, 0.0, 0.0], [25.0, 25.0, 24.0, 24.0, 22.0, 20.0, 23.0, 24.0, 21.0, 22.0, 25.0, 16.0, 30.0, 51.0, 112.0, 185.0, 149.0, 168.0, 231.0, 430.0, 588.0, 842.0, 1077.0, 1539.0, 1511.0, 1590.0, 1685.0, 2150.0, 1827.0, 1926.0, 1771.0, 1953.0, 1756.0, 1691.0, 1540.0, 1159.0, 1059.0, 701.0, 432.0, 267.0, 162.0, 135.0, 130.0, 148.0, 109.0, 88.0, 53.0, 41.0, 36.0, 19.0, 32.0, 35.0, 31.0, 23.0, 27.0, 27.0, 27.0, 0.0], [31.0, 28.0, 27.0, 21.0, 17.0, 21.0, 22.0, 28.0, 31.0, 30.0, 26.0, 31.0, 51.0, 85.0, 179.0, 162.0, 200.0, 238.0, 373.0, 566.0, 838.0, 1076.0, 965.0, 2073.0, 1860.0, 2338.0, 2087.0, 2183.0, 2159.0, 2026.0, 2259.0, 2148.0, 2208.0, 1766.0, 1719.0, 1376.0, 1184.0, 1006.0, 789.0, 365.0, 314.0, 155.0, 170.0, 148.0, 149.0, 103.0, 79.0, 32.0, 37.0, 36.0, 32.0, 41.0, 29.0, 27.0, 24.0, 29.0, 33.0, 0.0], [19.0, 22.0, 18.0, 24.0, 25.0, 29.0, 27.0, 24.0, 34.0, 22.0, 26.0, 43.0, 52.0, 125.0, 186.0, 155.0, 189.0, 314.0, 603.0, 802.0, 1200.0, 1529.0, 2843.0, 1582.0, 2150.0, 2271.0, 2342.0, 2106.0, 2259.0, 2414.0, 2188.0, 1850.0, 2598.0, 2074.0, 2007.0, 2071.0, 1589.0, 1388.0, 899.0, 684.0, 390.0, 226.0, 133.0, 126.0, 117.0, 125.0, 92.0, 51.0, 28.0, 34.0, 23.0, 21.0, 20.0, 29.0, 33.0, 24.0, 32.0, 0.0], [21.0, 27.0, 19.0, 21.0, 18.0, 12.0, 23.0, 31.0, 31.0, 25.0, 38.0, 37.0, 64.0, 165.0, 142.0, 188.0, 206.0, 421.0, 745.0, 1023.0, 1384.0, 1644.0, 1935.0, 1915.0, 2646.0, 2078.0, 2196.0, 2583.0, 2491.0, 2193.0, 2551.0, 2302.0, 2611.0, 2072.0, 2342.0, 2054.0, 1592.0, 1561.0, 1119.0, 846.0, 544.0, 304.0, 180.0, 143.0, 101.0, 173.0, 91.0, 63.0, 24.0, 34.0, 23.0, 27.0, 19.0, 23.0, 28.0, 25.0, 27.0, 16.0], [17.0, 19.0, 17.0, 20.0, 24.0, 22.0, 18.0, 30.0, 23.0, 30.0, 27.0, 47.0, 111.0, 135.0, 209.0, 197.0, 319.0, 550.0, 775.0, 1537.0, 1821.0, 1836.0, 2224.0, 2316.0, 2119.0, 2514.0, 2374.0, 2223.0, 2299.0, 2416.0, 2366.0, 2019.0, 2264.0, 2043.0, 2182.0, 2402.0, 1928.0, 1883.0, 1427.0, 1018.0, 703.0, 372.0, 209.0, 167.0, 125.0, 144.0, 126.0, 77.0, 51.0, 33.0, 31.0, 27.0, 27.0, 28.0, 21.0, 21.0, 26.0, 24.0], [25.0, 20.0, 25.0, 17.0, 20.0, 18.0, 18.0, 20.0, 23.0, 33.0, 27.0, 74.0, 170.0, 173.0, 179.0, 241.0, 471.0, 664.0, 1168.0, 1387.0, 1731.0, 2460.0, 2053.0, 2222.0, 2244.0, 2561.0, 2311.0, 2064.0, 2189.0, 2104.0, 2074.0, 2317.0, 2355.0, 2225.0, 2459.0, 2049.0, 2098.0, 1911.0, 1605.0, 1244.0, 880.0, 661.0, 283.0, 172.0, 143.0, 136.0, 125.0, 91.0, 44.0, 41.0, 19.0, 30.0, 20.0, 27.0, 23.0, 28.0, 28.0, 25.0], [19.0, 24.0, 29.0, 28.0, 33.0, 12.0, 20.0, 26.0, 27.0, 32.0, 46.0, 92.0, 160.0, 145.0, 183.0, 266.0, 426.0, 795.0, 1285.0, 1650.0, 1815.0, 2313.0, 2278.0, 2602.0, 2408.0, 2217.0, 2150.0, 2290.0, 2394.0, 1884.0, 2209.0, 1984.0, 2232.0, 2318.0, 2103.0, 2197.0, 2072.0, 2113.0, 1657.0, 1296.0, 1090.0, 688.0, 332.0, 180.0, 132.0, 137.0, 131.0, 106.0, 77.0, 35.0, 38.0, 16.0, 27.0, 36.0, 21.0, 26.0, 24.0, 26.0], [12.0, 23.0, 18.0, 11.0, 19.0, 21.0, 21.0, 17.0, 17.0, 45.0, 20.0, 115.0, 161.0, 180.0, 189.0, 341.0, 645.0, 1029.0, 1270.0, 1935.0, 2093.0, 2130.0, 2357.0, 2242.0, 2237.0, 2072.0, 2119.0, 1984.0, 1444.0, 2123.0, 1772.0, 2115.0, 2031.0, 2285.0, 2251.0, 2218.0, 2074.0, 1996.0, 1823.0, 1503.0, 1175.0, 626.0, 389.0, 219.0, 131.0, 132.0, 96.0, 98.0, 79.0, 38.0, 24.0, 35.0, 28.0, 29.0, 29.0, 29.0, 16.0, 26.0], [24.0, 24.0, 21.0, 24.0, 25.0, 25.0, 15.0, 20.0, 23.0, 33.0, 41.0, 119.0, 164.0, 169.0, 202.0, 370.0, 553.0, 1056.0, 1402.0, 1818.0, 2437.0, 2142.0, 2116.0, 2300.0, 2118.0, 2071.0, 1921.0, 1902.0, 2073.0, 1720.0, 1998.0, 1897.0, 1756.0, 2183.0, 2312.0, 2061.0, 2258.0, 2236.0, 1943.0, 1534.0, 1181.0, 799.0, 477.0, 264.0, 111.0, 127.0, 121.0, 111.0, 62.0, 40.0, 26.0, 29.0, 14.0, 28.0, 20.0, 26.0, 22.0, 27.0], [22.0, 21.0, 19.0, 21.0, 17.0, 20.0, 22.0, 17.0, 26.0, 24.0, 40.0, 110.0, 180.0, 169.0, 199.0, 365.0, 704.0, 1157.0, 1489.0, 1980.0, 2025.0, 2522.0, 2258.0, 2725.0, 1889.0, 2363.0, 1820.0, 1997.0, 1803.0, 1904.0, 1493.0, 1979.0, 2097.0, 2100.0, 2121.0, 2432.0, 2073.0, 2149.0, 1847.0, 1849.0, 1218.0, 934.0, 492.0, 198.0, 150.0, 119.0, 120.0, 96.0, 76.0, 56.0, 29.0, 19.0, 31.0, 29.0, 33.0, 35.0, 22.0, 20.0], [12.0, 19.0, 25.0, 19.0, 16.0, 18.0, 21.0, 20.0, 30.0, 30.0, 39.0, 121.0, 134.0, 178.0, 183.0, 423.0, 728.0, 1221.0, 1592.0, 2105.0, 2006.0, 2279.0, 2332.0, 2143.0, 1975.0, 2373.0, 1821.0, 2110.0, 1513.0, 1933.0, 1913.0, 2086.0, 1811.0, 2283.0, 2029.0, 2454.0, 2116.0, 2168.0, 1722.0, 1699.0, 1014.0, 973.0, 444.0, 254.0, 137.0, 115.0, 112.0, 70.0, 58.0, 30.0, 32.0, 28.0, 24.0, 19.0, 21.0, 23.0, 25.0, 24.0], [17.0, 27.0, 29.0, 22.0, 15.0, 16.0, 22.0, 27.0, 21.0, 31.0, 39.0, 112.0, 168.0, 191.0, 162.0, 418.0, 658.0, 1060.0, 1441.0, 1874.0, 2043.0, 2415.0, 2243.0, 2614.0, 2348.0, 1751.0, 1972.0, 1890.0, 1827.0, 1903.0, 1693.0, 2071.0, 1591.0, 2461.0, 2016.0, 2422.0, 2248.0, 2158.0, 1951.0, 1805.0, 1299.0, 897.0, 489.0, 261.0, 110.0, 152.0, 103.0, 144.0, 69.0, 42.0, 14.0, 15.0, 24.0, 25.0, 21.0, 16.0, 18.0, 19.0], [21.0, 21.0, 21.0, 26.0, 18.0, 28.0, 23.0, 23.0, 23.0, 27.0, 32.0, 149.0, 146.0, 161.0, 212.0, 386.0, 535.0, 1151.0, 1444.0, 2096.0, 2122.0, 2464.0, 2196.0, 2141.0, 2202.0, 2312.0, 2074.0, 1990.0, 1860.0, 1929.0, 2124.0, 2035.0, 2019.0, 2231.0, 2187.0, 2119.0, 2172.0, 2328.0, 1659.0, 1615.0, 1035.0, 830.0, 489.0, 251.0, 162.0, 144.0, 108.0, 104.0, 83.0, 29.0, 19.0, 35.0, 20.0, 14.0, 21.0, 19.0, 29.0, 20.0], [23.0, 33.0, 20.0, 32.0, 22.0, 24.0, 30.0, 19.0, 26.0, 34.0, 36.0, 92.0, 144.0, 198.0, 162.0, 344.0, 527.0, 954.0, 1233.0, 1884.0, 2108.0, 2409.0, 1970.0, 2857.0, 2011.0, 2459.0, 1965.0, 2281.0, 1928.0, 2001.0, 1672.0, 2054.0, 2091.0, 2136.0, 2189.0, 2677.0, 2079.0, 1956.0, 2040.0, 1535.0, 1125.0, 687.0, 411.0, 227.0, 117.0, 124.0, 100.0, 113.0, 74.0, 33.0, 24.0, 30.0, 25.0, 20.0, 24.0, 17.0, 17.0, 27.0], [17.0, 19.0, 15.0, 28.0, 15.0, 16.0, 16.0, 28.0, 24.0, 20.0, 39.0, 78.0, 158.0, 192.0, 177.0, 286.0, 441.0, 972.0, 1336.0, 1683.0, 1949.0, 2382.0, 2023.0, 2618.0, 2109.0, 2169.0, 2284.0, 2251.0, 1928.0, 2304.0, 1971.0, 2274.0, 1992.0, 2592.0, 2260.0, 2130.0, 2562.0, 2282.0, 1666.0, 1478.0, 1017.0, 669.0, 338.0, 170.0, 121.0, 131.0, 107.0, 82.0, 40.0, 38.0, 18.0, 29.0, 26.0, 24.0, 22.0, 18.0, 21.0, 22.0], [21.0, 22.0, 23.0, 21.0, 19.0, 19.0, 16.0, 18.0, 30.0, 27.0, 37.0, 66.0, 141.0, 177.0, 182.0, 197.0, 417.0, 634.0, 995.0, 1684.0, 1601.0, 2254.0, 2375.0, 2106.0, 2392.0, 2256.0, 2295.0, 2178.0, 2005.0, 2474.0, 1768.0, 2250.0, 2153.0, 2115.0, 2274.0, 2399.0, 2032.0, 1839.0, 1452.0, 1338.0, 816.0, 486.0, 238.0, 215.0, 86.0, 125.0, 102.0, 95.0, 48.0, 20.0, 25.0, 20.0, 23.0, 22.0, 29.0, 19.0, 21.0, 27.0], [27.0, 24.0, 14.0, 15.0, 13.0, 27.0, 19.0, 28.0, 26.0, 29.0, 20.0, 47.0, 109.0, 199.0, 147.0, 201.0, 261.0, 556.0, 855.0, 1386.0, 1789.0, 2046.0, 2139.0, 2352.0, 2374.0, 2424.0, 2299.0, 2334.0, 1939.0, 2701.0, 2280.0, 2239.0, 2025.0, 2334.0, 2230.0, 2470.0, 1918.0, 1963.0, 1408.0, 1183.0, 670.0, 460.0, 222.0, 148.0, 107.0, 160.0, 105.0, 61.0, 32.0, 40.0, 26.0, 17.0, 26.0, 22.0, 31.0, 23.0, 26.0, 35.0], [12.0, 17.0, 27.0, 19.0, 22.0, 22.0, 22.0, 25.0, 32.0, 18.0, 30.0, 30.0, 67.0, 152.0, 142.0, 214.0, 253.0, 525.0, 656.0, 1020.0, 1372.0, 1773.0, 2131.0, 2287.0, 1886.0, 2263.0, 2258.0, 2415.0, 2344.0, 2200.0, 2188.0, 2300.0, 2128.0, 2548.0, 2214.0, 1938.0, 1749.0, 1611.0, 1101.0, 842.0, 512.0, 265.0, 146.0, 140.0, 118.0, 129.0, 102.0, 75.0, 29.0, 28.0, 19.0, 25.0, 17.0, 29.0, 26.0, 20.0, 25.0, 26.0], [19.0, 25.0, 20.0, 16.0, 16.0, 25.0, 27.0, 32.0, 23.0, 31.0, 38.0, 35.0, 39.0, 136.0, 184.0, 201.0, 179.0, 292.0, 482.0, 1016.0, 1014.0, 1561.0, 1664.0, 2135.0, 2110.0, 2169.0, 2083.0, 2320.0, 1992.0, 2526.0, 2043.0, 2504.0, 2168.0, 2210.0, 1892.0, 1910.0, 1415.0, 1535.0, 764.0, 674.0, 370.0, 225.0, 128.0, 129.0, 135.0, 125.0, 82.0, 45.0, 18.0, 25.0, 24.0, 33.0, 29.0, 19.0, 15.0, 28.0, 26.0, 0.0], [12.0, 21.0, 14.0, 21.0, 21.0, 19.0, 15.0, 28.0, 26.0, 23.0, 29.0, 34.0, 29.0, 80.0, 174.0, 164.0, 146.0, 265.0, 323.0, 566.0, 779.0, 1068.0, 1215.0, 1906.0, 1633.0, 2358.0, 2058.0, 2229.0, 2192.0, 2205.0, 2129.0, 2249.0, 1828.0, 1993.0, 1755.0, 1643.0, 1132.0, 1172.0, 753.0, 433.0, 196.0, 145.0, 133.0, 126.0, 124.0, 94.0, 57.0, 45.0, 29.0, 28.0, 24.0, 32.0, 21.0, 20.0, 22.0, 31.0, 23.0, 0.0], [11.0, 19.0, 23.0, 19.0, 29.0, 14.0, 25.0, 27.0, 27.0, 31.0, 25.0, 29.0, 34.0, 47.0, 107.0, 197.0, 175.0, 178.0, 213.0, 437.0, 525.0, 891.0, 1146.0, 1298.0, 1495.0, 1777.0, 1703.0, 1754.0, 1790.0, 1936.0, 1799.0, 1980.0, 1573.0, 1781.0, 1189.0, 1283.0, 845.0, 697.0, 458.0, 302.0, 180.0, 140.0, 112.0, 143.0, 124.0, 100.0, 45.0, 25.0, 18.0, 20.0, 18.0, 21.0, 25.0, 18.0, 13.0, 27.0, 25.0, 0.0], [0.0, 15.0, 25.0, 19.0, 21.0, 25.0, 28.0, 19.0, 19.0, 32.0, 29.0, 31.0, 21.0, 51.0, 72.0, 172.0, 153.0, 179.0, 186.0, 220.0, 321.0, 504.0, 658.0, 1030.0, 1028.0, 1267.0, 1404.0, 1449.0, 1519.0, 1608.0, 1531.0, 1442.0, 1292.0, 1146.0, 995.0, 983.0, 719.0, 407.0, 300.0, 196.0, 123.0, 135.0, 137.0, 112.0, 70.0, 59.0, 20.0, 27.0, 25.0, 35.0, 11.0, 21.0, 21.0, 17.0, 21.0, 29.0, 0.0, 0.0], [0.0, 22.0, 17.0, 28.0, 16.0, 22.0, 25.0, 29.0, 18.0, 35.0, 30.0, 32.0, 28.0, 33.0, 41.0, 71.0, 186.0, 164.0, 155.0, 148.0, 235.0, 333.0, 431.0, 632.0, 658.0, 937.0, 932.0, 1294.0, 1034.0, 1135.0, 1256.0, 1084.0, 837.0, 961.0, 655.0, 455.0, 296.0, 244.0, 193.0, 147.0, 125.0, 168.0, 142.0, 101.0, 82.0, 45.0, 32.0, 29.0, 15.0, 24.0, 19.0, 21.0, 13.0, 24.0, 28.0, 14.0, 0.0, 0.0], [0.0, 19.0, 12.0, 20.0, 20.0, 12.0, 18.0, 18.0, 25.0, 24.0, 24.0, 32.0, 30.0, 27.0, 43.0, 45.0, 81.0, 141.0, 148.0, 137.0, 172.0, 204.0, 195.0, 328.0, 431.0, 612.0, 557.0, 807.0, 682.0, 789.0, 659.0, 621.0, 519.0, 537.0, 340.0, 325.0, 198.0, 171.0, 123.0, 142.0, 135.0, 128.0, 95.0, 89.0, 33.0, 28.0, 21.0, 18.0, 18.0, 16.0, 19.0, 21.0, 20.0, 18.0, 16.0, 22.0, 0.0, 0.0], [0.0, 0.0, 26.0, 24.0, 21.0, 21.0, 35.0, 28.0, 32.0, 21.0, 30.0, 31.0, 38.0, 23.0, 32.0, 54.0, 63.0, 91.0, 134.0, 190.0, 158.0, 156.0, 144.0, 233.0, 242.0, 255.0, 300.0, 356.0, 387.0, 422.0, 422.0, 380.0, 304.0, 293.0, 194.0, 148.0, 123.0, 125.0, 163.0, 156.0, 119.0, 106.0, 65.0, 45.0, 27.0, 33.0, 13.0, 24.0, 18.0, 13.0, 23.0, 21.0, 20.0, 22.0, 19.0, 0.0, 0.0, 0.0], [0.0, 0.0, 0.0, 22.0, 22.0, 21.0, 19.0, 20.0, 27.0, 21.0, 24.0, 32.0, 29.0, 27.0, 24.0, 33.0, 40.0, 36.0, 63.0, 155.0, 167.0, 192.0, 137.0, 120.0, 162.0, 174.0, 176.0, 205.0, 191.0, 249.0, 218.0, 225.0, 158.0, 155.0, 119.0, 152.0, 149.0, 141.0, 143.0, 152.0, 94.0, 75.0, 36.0, 21.0, 22.0, 25.0, 27.0, 32.0, 21.0, 30.0, 16.0, 32.0, 13.0, 35.0, 0.0, 0.0, 0.0, 0.0], [0.0, 0.0, 0.0, 16.0, 26.0, 20.0, 22.0, 24.0, 33.0, 45.0, 27.0, 24.0, 14.0, 35.0, 22.0, 22.0, 36.0, 36.0, 38.0, 58.0, 107.0, 166.0, 155.0, 148.0, 180.0, 141.0, 136.0, 191.0, 138.0, 162.0, 139.0, 146.0, 117.0, 142.0, 159.0, 170.0, 146.0, 134.0, 109.0, 89.0, 33.0, 29.0, 25.0, 23.0, 29.0, 18.0, 21.0, 21.0, 12.0, 15.0, 21.0, 11.0, 34.0, 15.0, 0.0, 0.0, 0.0, 0.0], [0.0, 0.0, 0.0, 0.0, 12.0, 27.0, 26.0, 24.0, 30.0, 24.0, 25.0, 21.0, 27.0, 26.0, 31.0, 37.0, 37.0, 35.0, 36.0, 40.0, 42.0, 84.0, 115.0, 137.0, 167.0, 157.0, 153.0, 174.0, 118.0, 208.0, 161.0, 167.0, 186.0, 178.0, 142.0, 141.0, 108.0, 102.0, 67.0, 29.0, 28.0, 18.0, 30.0, 24.0, 20.0, 23.0, 20.0, 19.0, 16.0, 25.0, 19.0, 11.0, 19.0, 0.0, 0.0, 0.0, 0.0, 0.0], [0.0, 0.0, 0.0, 0.0, 0.0, 31.0, 22.0, 24.0, 17.0, 17.0, 25.0, 27.0, 24.0, 26.0, 29.0, 33.0, 34.0, 30.0, 20.0, 26.0, 30.0, 40.0, 42.0, 50.0, 68.0, 108.0, 117.0, 149.0, 158.0, 158.0, 129.0, 136.0, 125.0, 138.0, 102.0, 78.0, 54.0, 39.0, 42.0, 52.0, 23.0, 17.0, 22.0, 25.0, 27.0, 24.0, 18.0, 19.0, 17.0, 16.0, 20.0, 17.0, 0.0, 0.0, 0.0, 0.0, 0.0, 0.0], [0.0, 0.0, 0.0, 0.0, 0.0, 23.0, 30.0, 26.0, 18.0, 17.0, 32.0, 27.0, 28.0, 21.0, 14.0, 26.0, 19.0, 32.0, 30.0, 37.0, 26.0, 35.0, 28.0, 42.0, 40.0, 35.0, 51.0, 48.0, 53.0, 88.0, 92.0, 86.0, 59.0, 51.0, 26.0, 31.0, 27.0, 35.0, 21.0, 23.0, 25.0, 26.0, 21.0, 29.0, 14.0, 15.0, 20.0, 31.0, 24.0, 23.0, 22.0, 15.0, 0.0, 0.0, 0.0, 0.0, 0.0, 0.0], [0.0, 0.0, 0.0, 0.0, 0.0, 0.0, 21.0, 20.0, 30.0, 25.0, 22.0, 20.0, 21.0, 25.0, 27.0, 26.0, 22.0, 31.0, 16.0, 31.0, 24.0, 30.0, 28.0, 41.0, 33.0, 43.0, 43.0, 26.0, 27.0, 41.0, 33.0, 31.0, 18.0, 29.0, 29.0, 20.0, 19.0, 33.0, 20.0, 22.0, 19.0, 27.0, 22.0, 22.0, 24.0, 20.0, 14.0, 24.0, 18.0, 23.0, 14.0, 0.0, 0.0, 0.0, 0.0, 0.0, 0.0, 0.0], [0.0, 0.0, 0.0, 0.0, 0.0, 0.0, 0.0, 22.0, 19.0, 29.0, 22.0, 29.0, 24.0, 35.0, 18.0, 20.0, 32.0, 37.0, 27.0, 29.0, 30.0, 25.0, 36.0, 26.0, 35.0, 33.0, 28.0, 19.0, 34.0, 25.0, 23.0, 32.0, 33.0, 30.0, 24.0, 16.0, 18.0, 35.0, 18.0, 25.0, 20.0, 17.0, 23.0, 23.0, 19.0, 20.0, 22.0, 24.0, 15.0, 24.0, 0.0, 0.0, 0.0, 0.0, 0.0, 0.0, 0.0, 0.0], [0.0, 0.0, 0.0, 0.0, 0.0, 0.0, 0.0, 0.0, 26.0, 24.0, 29.0, 29.0, 14.0, 20.0, 20.0, 29.0, 19.0, 27.0, 21.0, 27.0, 24.0, 29.0, 30.0, 31.0, 22.0, 28.0, 23.0, 24.0, 25.0, 17.0, 29.0, 13.0, 28.0, 42.0, 23.0, 23.0, 24.0, 22.0, 17.0, 18.0, 11.0, 20.0, 20.0, 22.0, 29.0, 12.0, 12.0, 25.0, 20.0, 0.0, 0.0, 0.0, 0.0, 0.0, 0.0, 0.0, 0.0, 0.0], [0.0, 0.0, 0.0, 0.0, 0.0, 0.0, 0.0, 0.0, 0.0, 19.0, 28.0, 26.0, 20.0, 21.0, 14.0, 25.0, 28.0, 29.0, 26.0, 28.0, 27.0, 30.0, 31.0, 26.0, 33.0, 33.0, 22.0, 21.0, 19.0, 22.0, 31.0, 25.0, 32.0, 25.0, 16.0, 32.0, 29.0, 27.0, 19.0, 20.0, 30.0, 21.0, 15.0, 19.0, 18.0, 17.0, 14.0, 18.0, 0.0, 0.0, 0.0, 0.0, 0.0, 0.0, 0.0, 0.0, 0.0, 0.0], [0.0, 0.0, 0.0, 0.0, 0.0, 0.0, 0.0, 0.0, 0.0, 0.0, 0.0, 28.0, 19.0, 29.0, 21.0, 16.0, 33.0, 26.0, 22.0, 33.0, 21.0, 20.0, 30.0, 31.0, 26.0, 35.0, 16.0, 22.0, 16.0, 16.0, 28.0, 13.0, 20.0, 13.0, 22.0, 18.0, 13.0, 22.0, 23.0, 27.0, 18.0, 13.0, 17.0, 15.0, 15.0, 21.0, 0.0, 0.0, 0.0, 0.0, 0.0, 0.0, 0.0, 0.0, 0.0, 0.0, 0.0, 0.0], [0.0, 0.0, 0.0, 0.0, 0.0, 0.0, 0.0, 0.0, 0.0, 0.0, 0.0, 0.0, 20.0, 18.0, 18.0, 33.0, 22.0, 27.0, 32.0, 17.0, 23.0, 27.0, 31.0, 21.0, 16.0, 21.0, 25.0, 18.0, 26.0, 22.0, 17.0, 24.0, 16.0, 22.0, 28.0, 20.0, 19.0, 23.0, 21.0, 30.0, 16.0, 19.0, 18.0, 19.0, 15.0, 0.0, 0.0, 0.0, 0.0, 0.0, 0.0, 0.0, 0.0, 0.0, 0.0, 0.0, 0.0, 0.0], [0.0, 0.0, 0.0, 0.0, 0.0, 0.0, 0.0, 0.0, 0.0, 0.0, 0.0, 0.0, 0.0, 0.0, 21.0, 20.0, 16.0, 23.0, 18.0, 22.0, 17.0, 12.0, 27.0, 29.0, 27.0, 23.0, 26.0, 25.0, 24.0, 18.0, 16.0, 19.0, 16.0, 19.0, 20.0, 19.0, 22.0, 20.0, 20.0, 14.0, 12.0, 17.0, 17.0, 0.0, 0.0, 0.0, 0.0, 0.0, 0.0, 0.0, 0.0, 0.0, 0.0, 0.0, 0.0, 0.0, 0.0, 0.0], [0.0, 0.0, 0.0, 0.0, 0.0, 0.0, 0.0, 0.0, 0.0, 0.0, 0.0, 0.0, 0.0, 0.0, 0.0, 21.0, 19.0, 33.0, 24.0, 34.0, 29.0, 34.0, 34.0, 15.0, 23.0, 20.0, 30.0, 14.0, 21.0, 21.0, 24.0, 15.0, 27.0, 25.0, 29.0, 22.0, 11.0, 27.0, 20.0, 24.0, 18.0, 18.0, 0.0, 0.0, 0.0, 0.0, 0.0, 0.0, 0.0, 0.0, 0.0, 0.0, 0.0, 0.0, 0.0, 0.0, 0.0, 0.0], [0.0, 0.0, 0.0, 0.0, 0.0, 0.0, 0.0, 0.0, 0.0, 0.0, 0.0, 0.0, 0.0, 0.0, 0.0, 0.0, 0.0, 0.0, 23.0, 24.0, 25.0, 15.0, 21.0, 22.0, 25.0, 24.0, 22.0, 20.0, 16.0, 21.0, 19.0, 28.0, 15.0, 20.0, 24.0, 15.0, 27.0, 24.0, 20.0, 0.0, 0.0, 0.0, 0.0, 0.0, 0.0, 0.0, 0.0, 0.0, 0.0, 0.0, 0.0, 0.0, 0.0, 0.0, 0.0, 0.0, 0.0, 0.0], [0.0, 0.0, 0.0, 0.0, 0.0, 0.0, 0.0, 0.0, 0.0, 0.0, 0.0, 0.0, 0.0, 0.0, 0.0, 0.0, 0.0, 0.0, 0.0, 0.0, 0.0, 29.0, 17.0, 22.0, 18.0, 25.0, 12.0, 18.0, 21.0, 27.0, 13.0, 21.0, 20.0, 18.0, 23.0, 14.0, 0.0, 0.0, 0.0, 0.0, 0.0, 0.0, 0.0, 0.0, 0.0, 0.0, 0.0, 0.0, 0.0, 0.0, 0.0, 0.0, 0.0, 0.0, 0.0, 0.0, 0.0, 0.0]]
  out "Signal Bck ref":dbl[][](graph)
  out "Coincidence image ref":dbl[][](graph)
  out "Coincidence image ref bck":dbl[][](graph)
  out "Signal Idler pix crop":T2
  out "Background pix crop":T2
  in  "Signal (Near Field) ROI":T3={"Near Field  Row"=130, "Near Field Col"=125, "Near Field outer radius"=75, "Near Field inner radius"=0}
  in  "Magnification":dbl=37.5 format="%#_13g"
  in  "Reference Background files":path caption="start path"
  in  "Reference Coincidence files":path caption="start path"
  in  "Subtract Background?":bool=TRUE
  in  "Phase":enum32{"Phase", "Phase gradient"}(tab)
  out "Phase":dbl[][](graph)
  out "Poisson":dbl[][](graph)
  out "Shift kx":dbl[][](graph)
  out "Shift ky":dbl[][](graph)
  in  "Data images":T4(tab)
  out "Signal":dbl[][](graph)
  out "Idler":dbl[][](graph)=[[0.0, 0.0, 0.0, 0.0, 0.0, 0.0, 0.0, 0.0, 0.0, 0.0, 0.0, 0.0, 0.0, 0.0, 0.0, 0.0, 0.0, 0.0, 57.0, 49.0, 43.0, 67.0, 62.0, 70.0, 65.0, 67.0, 76.0, 67.0, 75.0, 52.0, 68.0, 77.0, 70.0, 76.0, 64.0, 81.0, 59.0, 75.0, 40.0, 0.0, 0.0, 0.0, 0.0, 0.0, 0.0, 0.0, 0.0, 0.0, 0.0, 0.0, 0.0, 0.0, 0.0, 0.0, 0.0, 0.0, 0.0, 0.0], [0.0, 0.0, 0.0, 0.0, 0.0, 0.0, 0.0, 0.0, 0.0, 0.0, 0.0, 0.0, 0.0, 0.0, 0.0, 38.0, 33.0, 47.0, 45.0, 54.0, 63.0, 59.0, 67.0, 54.0, 60.0, 112.0, 60.0, 70.0, 73.0, 83.0, 79.0, 78.0, 49.0, 66.0, 69.0, 58.0, 57.0, 63.0, 59.0, 47.0, 35.0, 37.0, 0.0, 0.0, 0.0, 0.0, 0.0, 0.0, 0.0, 0.0, 0.0, 0.0, 0.0, 0.0, 0.0, 0.0, 0.0, 0.0], [0.0, 0.0, 0.0, 0.0, 0.0, 0.0, 0.0, 0.0, 0.0, 0.0, 0.0, 0.0, 0.0, 0.0, 40.0, 50.0, 51.0, 48.0, 35.0, 56.0, 66.0, 56.0, 74.0, 83.0, 56.0, 69.0, 80.0, 91.0, 87.0, 70.0, 90.0, 71.0, 88.0, 79.0, 66.0, 76.0, 85.0, 48.0, 60.0, 75.0, 38.0, 37.0, 48.0, 0.0, 0.0, 0.0, 0.0, 0.0, 0.0, 0.0, 0.0, 0.0, 0.0, 0.0, 0.0, 0.0, 0.0, 0.0], [0.0, 0.0, 0.0, 0.0, 0.0, 0.0, 0.0, 0.0, 0.0, 0.0, 0.0, 0.0, 33.0, 30.0, 28.0, 55.0, 43.0, 46.0, 52.0, 35.0, 62.0, 66.0, 69.0, 76.0, 80.0, 80.0, 110.0, 86.0, 87.0, 81.0, 68.0, 103.0, 70.0, 70.0, 79.0, 68.0, 70.0, 63.0, 45.0, 62.0, 42.0, 44.0, 30.0, 53.0, 41.0, 0.0, 0.0, 0.0, 0.0, 0.0, 0.0, 0.0, 0.0, 0.0, 0.0, 0.0, 0.0, 0.0], [0.0, 0.0, 0.0, 0.0, 0.0, 0.0, 0.0, 0.0, 0.0, 0.0, 0.0, 33.0, 29.0, 48.0, 41.0, 39.0, 45.0, 41.0, 58.0, 73.0, 66.0, 89.0, 89.0, 101.0, 55.0, 86.0, 83.0, 96.0, 85.0, 133.0, 86.0, 101.0, 92.0, 79.0, 73.0, 69.0, 91.0, 75.0, 50.0, 70.0, 52.0, 40.0, 41.0, 32.0, 37.0, 43.0, 0.0, 0.0, 0.0, 0.0, 0.0, 0.0, 0.0, 0.0, 0.0, 0.0, 0.0, 0.0], [0.0, 0.0, 0.0, 0.0, 0.0, 0.0, 0.0, 0.0, 0.0, 24.0, 31.0, 35.0, 31.0, 38.0, 31.0, 34.0, 41.0, 53.0, 59.0, 53.0, 53.0, 74.0, 96.0, 98.0, 71.0, 108.0, 93.0, 95.0, 103.0, 97.0, 95.0, 92.0, 100.0, 90.0, 95.0, 81.0, 74.0, 61.0, 71.0, 60.0, 47.0, 58.0, 49.0, 39.0, 52.0, 35.0, 31.0, 44.0, 0.0, 0.0, 0.0, 0.0, 0.0, 0.0, 0.0, 0.0, 0.0, 0.0], [0.0, 0.0, 0.0, 0.0, 0.0, 0.0, 0.0, 0.0, 19.0, 39.0, 27.0, 32.0, 36.0, 41.0, 38.0, 40.0, 39.0, 52.0, 53.0, 59.0, 86.0, 70.0, 56.0, 95.0, 110.0, 117.0, 113.0, 106.0, 105.0, 130.0, 111.0, 85.0, 84.0, 114.0, 94.0, 102.0, 72.0, 78.0, 78.0, 64.0, 70.0, 48.0, 56.0, 55.0, 40.0, 42.0, 37.0, 31.0, 42.0, 0.0, 0.0, 0.0, 0.0, 0.0, 0.0, 0.0, 0.0, 0.0], [0.0, 0.0, 0.0, 0.0, 0.0, 0.0, 0.0, 30.0, 24.0, 43.0, 35.0, 34.0, 25.0, 49.0, 30.0, 37.0, 43.0, 66.0, 69.0, 72.0, 94.0, 95.0, 112.0, 98.0, 101.0, 128.0, 113.0, 138.0, 127.0, 116.0, 105.0, 134.0, 129.0, 113.0, 112.0, 108.0, 81.0, 94.0, 65.0, 70.0, 71.0, 64.0, 58.0, 39.0, 41.0, 45.0, 40.0, 47.0, 35.0, 51.0, 0.0, 0.0, 0.0, 0.0, 0.0, 0.0, 0.0, 0.0], [0.0, 0.0, 0.0, 0.0, 0.0, 0.0, 19.0, 30.0, 27.0, 38.0, 29.0, 18.0, 44.0, 39.0, 41.0, 59.0, 52.0, 65.0, 57.0, 89.0, 96.0, 99.0, 94.0, 129.0, 118.0, 158.0, 153.0, 147.0, 140.0, 181.0, 202.0, 135.0, 139.0, 136.0, 136.0, 128.0, 101.0, 93.0, 85.0, 78.0, 67.0, 54.0, 50.0, 50.0, 45.0, 38.0, 29.0, 30.0, 38.0, 38.0, 37.0, 0.0, 0.0, 0.0, 0.0, 0.0, 0.0, 0.0], [0.0, 0.0, 0.0, 0.0, 0.0, 41.0, 24.0, 39.0, 27.0, 29.0, 36.0, 40.0, 28.0, 44.0, 39.0, 51.0, 56.0, 77.0, 73.0, 98.0, 76.0, 121.0, 156.0, 131.0, 154.0, 172.0, 169.0, 209.0, 326.0, 281.0, 239.0, 275.0, 221.0, 178.0, 171.0, 138.0, 123.0, 129.0, 80.0, 84.0, 73.0, 58.0, 57.0, 49.0, 48.0, 35.0, 59.0, 54.0, 32.0, 42.0, 36.0, 25.0, 0.0, 0.0, 0.0, 0.0, 0.0, 0.0], [0.0, 0.0, 0.0, 0.0, 0.0, 27.0, 29.0, 24.0, 31.0, 34.0, 34.0, 53.0, 36.0, 26.0, 46.0, 50.0, 48.0, 77.0, 96.0, 102.0, 128.0, 140.0, 161.0, 290.0, 376.0, 446.0, 629.0, 601.0, 527.0, 615.0, 586.0, 581.0, 515.0, 416.0, 332.0, 261.0, 214.0, 163.0, 108.0, 102.0, 91.0, 57.0, 63.0, 65.0, 53.0, 35.0, 36.0, 55.0, 46.0, 39.0, 34.0, 34.0, 0.0, 0.0, 0.0, 0.0, 0.0, 0.0], [0.0, 0.0, 0.0, 0.0, 25.0, 34.0, 37.0, 39.0, 34.0, 27.0, 49.0, 28.0, 40.0, 61.0, 45.0, 61.0, 67.0, 107.0, 99.0, 124.0, 181.0, 340.0, 522.0, 584.0, 687.0, 606.0, 721.0, 572.0, 675.0, 586.0, 709.0, 638.0, 627.0, 580.0, 627.0, 622.0, 413.0, 370.0, 208.0, 136.0, 77.0, 94.0, 71.0, 60.0, 49.0, 50.0, 56.0, 38.0, 41.0, 33.0, 37.0, 32.0, 35.0, 0.0, 0.0, 0.0, 0.0, 0.0], [0.0, 0.0, 0.0, 22.0, 32.0, 32.0, 27.0, 47.0, 32.0, 35.0, 32.0, 53.0, 42.0, 58.0, 56.0, 78.0, 87.0, 92.0, 158.0, 180.0, 395.0, 606.0, 646.0, 707.0, 565.0, 597.0, 552.0, 608.0, 520.0, 582.0, 467.0, 544.0, 565.0, 518.0, 575.0, 602.0, 645.0, 521.0, 462.0, 266.0, 139.0, 96.0, 80.0, 73.0, 44.0, 65.0, 54.0, 55.0, 36.0, 44.0, 53.0, 34.0, 36.0, 43.0, 0.0, 0.0, 0.0, 0.0], [0.0, 0.0, 0.0, 33.0, 33.0, 36.0, 45.0, 27.0, 36.0, 31.0, 35.0, 38.0, 58.0, 48.0, 60.0, 78.0, 101.0, 153.0, 251.0, 534.0, 689.0, 698.0, 572.0, 517.0, 656.0, 660.0, 626.0, 840.0, 756.0, 866.0, 847.0, 750.0, 587.0, 667.0, 550.0, 530.0, 497.0, 582.0, 535.0, 553.0, 354.0, 164.0, 92.0, 78.0, 70.0, 48.0, 46.0, 36.0, 49.0, 46.0, 35.0, 40.0, 32.0, 28.0, 0.0, 0.0, 0.0, 0.0], [0.0, 0.0, 31.0, 33.0, 23.0, 36.0, 46.0, 40.0, 46.0, 45.0, 42.0, 44.0, 64.0, 47.0, 72.0, 88.0, 133.0, 299.0, 583.0, 633.0, 624.0, 532.0, 691.0, 669.0, 962.0, 1084.0, 1421.0, 1630.0, 1697.0, 1690.0, 1602.0, 1653.0, 1257.0, 1144.0, 873.0, 658.0, 611.0, 555.0, 512.0, 638.0, 453.0, 350.0, 128.0, 81.0, 87.0, 68.0, 51.0, 49.0, 46.0, 52.0, 41.0, 36.0, 50.0, 43.0, 35.0, 0.0, 0.0, 0.0], [0.0, 38.0, 24.0, 37.0, 32.0, 47.0, 40.0, 46.0, 35.0, 37.0, 59.0, 62.0, 59.0, 100.0, 111.0, 137.0, 356.0, 533.0, 600.0, 626.0, 585.0, 719.0, 958.0, 1463.0, 1952.0, 2127.0, 2963.0, 3024.0, 3327.0, 3119.0, 3526.0, 2988.0, 2554.0, 2256.0, 1766.0, 1251.0, 840.0, 627.0, 534.0, 509.0, 543.0, 554.0, 392.0, 156.0, 94.0, 66.0, 61.0, 68.0, 59.0, 47.0, 47.0, 35.0, 34.0, 35.0, 42.0, 43.0, 0.0, 0.0], [0.0, 36.0, 33.0, 36.0, 33.0, 37.0, 28.0, 56.0, 50.0, 56.0, 64.0, 52.0, 66.0, 90.0, 109.0, 333.0, 589.0, 676.0, 496.0, 641.0, 741.0, 1345.0, 1694.0, 2501.0, 3724.0, 4510.0, 4732.0, 5317.0, 5818.0, 6458.0, 5675.0, 5108.0, 4736.0, 3743.0, 3034.0, 2392.0, 1589.0, 1031.0, 683.0, 562.0, 443.0, 624.0, 459.0, 408.0, 130.0, 72.0, 86.0, 59.0, 56.0, 55.0, 45.0, 57.0, 43.0, 40.0, 36.0, 27.0, 0.0, 0.0], [0.0, 46.0, 40.0, 36.0, 25.0, 42.0, 58.0, 56.0, 43.0, 66.0, 64.0, 98.0, 84.0, 123.0, 270.0, 538.0, 581.0, 606.0, 588.0, 896.0, 1534.0, 2062.0, 3488.0, 4691.0, 5408.0, 6555.0, 7335.0, 7320.0, 7879.0, 7159.0, 7726.0, 6795.0, 6310.0, 6313.0, 4906.0, 4428.0, 2898.0, 2222.0, 1366.0, 749.0, 549.0, 490.0, 521.0, 548.0, 272.0, 167.0, 69.0, 72.0, 69.0, 56.0, 54.0, 48.0, 51.0, 46.0, 31.0, 32.0, 0.0, 0.0], [27.0, 37.0, 48.0, 47.0, 48.0, 41.0, 48.0, 60.0, 60.0, 57.0, 77.0, 79.0, 95.0, 145.0, 436.0, 661.0, 589.0, 559.0, 811.0, 1590.0, 2458.0, 3724.0, 4945.0, 6945.0, 7160.0, 7757.0, 8324.0, 10140.0, 8604.0, 8924.0, 8604.0, 9083.0, 8133.0, 7799.0, 6908.0, 5354.0, 4906.0, 3223.0, 1994.0, 1350.0, 659.0, 531.0, 540.0, 542.0, 407.0, 211.0, 118.0, 85.0, 58.0, 73.0, 39.0, 56.0, 57.0, 45.0, 27.0, 41.0, 37.0, 0.0], [32.0, 40.0, 50.0, 40.0, 36.0, 48.0, 62.0, 54.0, 62.0, 79.0, 87.0, 98.0, 154.0, 331.0, 659.0, 598.0, 651.0, 796.0, 1387.0, 2361.0, 3664.0, 5192.0, 4864.0, 9306.0, 8938.0, 10876.0, 9949.0, 10370.0, 9847.0, 10227.0, 10675.0, 10232.0, 10211.0, 8839.0, 8224.0, 7219.0, 5758.0, 4832.0, 3313.0, 1812.0, 1313.0, 611.0, 465.0, 563.0, 565.0, 331.0, 149.0, 90.0, 71.0, 54.0, 63.0, 61.0, 54.0, 57.0, 60.0, 57.0, 47.0, 0.0], [40.0, 59.0, 50.0, 52.0, 55.0, 43.0, 56.0, 47.0, 64.0, 68.0, 75.0, 114.0, 194.0, 456.0, 618.0, 569.0, 643.0, 1147.0, 2287.0, 3571.0, 5079.0, 6673.0, 12486.0, 7493.0, 9908.0, 10522.0, 10704.0, 10145.0, 10812.0, 11419.0, 10336.0, 9040.0, 11533.0, 9856.0, 9764.0, 9337.0, 7767.0, 6618.0, 4530.0, 3186.0, 1771.0, 934.0, 534.0, 458.0, 548.0, 443.0, 200.0, 121.0, 64.0, 90.0, 61.0, 64.0, 45.0, 47.0, 46.0, 59.0, 39.0, 0.0], [46.0, 32.0, 47.0, 54.0, 47.0, 55.0, 52.0, 79.0, 78.0, 89.0, 106.0, 133.0, 265.0, 666.0, 582.0, 702.0, 851.0, 1735.0, 3143.0, 4726.0, 6507.0, 7531.0, 9052.0, 9347.0, 12466.0, 9822.0, 10218.0, 12049.0, 11257.0, 9801.0, 11456.0, 10796.0, 12064.0, 10495.0, 10702.0, 9605.0, 8219.0, 7753.0, 5663.0, 4095.0, 2619.0, 1402.0, 651.0, 523.0, 412.0, 631.0, 274.0, 166.0, 80.0, 103.0, 87.0, 73.0, 64.0, 61.0, 49.0, 54.0, 47.0, 48.0], [37.0, 49.0, 41.0, 30.0, 44.0, 60.0, 78.0, 72.0, 68.0, 114.0, 82.0, 150.0, 460.0, 613.0, 630.0, 627.0, 1137.0, 2284.0, 3508.0, 6622.0, 8473.0, 8988.0, 10690.0, 11364.0, 10376.0, 11713.0, 10750.0, 10237.0, 9938.0, 11003.0, 10682.0, 10028.0, 10471.0, 10250.0, 10392.0, 11222.0, 9150.0, 8980.0, 6815.0, 5055.0, 3209.0, 1736.0, 864.0, 548.0, 501.0, 575.0, 397.0, 178.0, 112.0, 80.0, 54.0, 64.0, 54.0, 59.0, 58.0, 53.0, 60.0, 49.0], [46.0, 40.0, 50.0, 54.0, 59.0, 69.0, 65.0, 69.0, 78.0, 109.0, 109.0, 250.0, 579.0, 646.0, 649.0, 793.0, 1855.0, 2935.0, 5274.0, 6655.0, 8251.0, 11346.0, 10149.0, 10538.0, 10783.0, 11527.0, 10424.0, 9668.0, 10153.0, 9793.0, 9814.0, 11040.0, 10799.0, 10106.0, 11585.0, 10130.0, 9947.0, 9193.0, 7772.0, 6337.0, 4136.0, 2647.0, 1075.0, 573.0, 517.0, 510.0, 493.0, 244.0, 112.0, 100.0, 60.0, 76.0, 69.0, 56.0, 44.0, 50.0, 43.0, 55.0], [47.0, 52.0, 46.0, 58.0, 56.0, 43.0, 61.0, 88.0, 86.0, 110.0, 151.0, 324.0, 624.0, 607.0, 666.0, 996.0, 1803.0, 3459.0, 5992.0, 7900.0, 8791.0, 11010.0, 10693.0, 11917.0, 11061.0, 10210.0, 9944.0, 9815.0, 10487.0, 8548.0, 9932.0, 9328.0, 10074.0, 10831.0, 10266.0, 10565.0, 10268.0, 10072.0, 8317.0, 6264.0, 4935.0, 3297.0, 1424.0, 645.0, 488.0, 528.0, 534.0, 339.0, 155.0, 96.0, 85.0, 65.0, 88.0, 54.0, 57.0, 57.0, 52.0, 54.0], [39.0, 45.0, 49.0, 52.0, 44.0, 60.0, 76.0, 80.0, 84.0, 144.0, 148.0, 448.0, 586.0, 681.0, 664.0, 1327.0, 2578.0, 4390.0, 6111.0, 9415.0, 9706.0, 10440.0, 11165.0, 10977.0, 10739.0, 9905.0, 9485.0, 9109.0, 7133.0, 9596.0, 8479.0, 9967.0, 9383.0, 10386.0, 10613.0, 10688.0, 9774.0, 10024.0, 8751.0, 7262.0, 5437.0, 3107.0, 1829.0, 921.0, 451.0, 538.0, 440.0, 372.0, 174.0, 123.0, 75.0, 70.0, 53.0, 66.0, 58.0, 68.0, 47.0, 51.0], [48.0, 50.0, 49.0, 62.0, 59.0, 50.0, 58.0, 112.0, 101.0, 106.0, 172.0, 435.0, 681.0, 545.0, 627.0, 1368.0, 2448.0, 4700.0, 6446.0, 8584.0, 11226.0, 10382.0, 10245.0, 10964.0, 10026.0, 9736.0, 9134.0, 8793.0, 9394.0, 8242.0, 9250.0, 8700.0, 8829.0, 10074.0, 10511.0, 9798.0, 10767.0, 10687.0, 9496.0, 7284.0, 5690.0, 3830.0, 1931.0, 1017.0, 492.0, 591.0, 507.0, 395.0, 165.0, 120.0, 91.0, 77.0, 66.0, 53.0, 79.0, 59.0, 57.0, 60.0], [41.0, 52.0, 56.0, 41.0, 56.0, 54.0, 82.0, 96.0, 98.0, 112.0, 167.0, 417.0, 712.0, 611.0, 763.0, 1389.0, 2858.0, 4995.0, 7046.0, 9295.0, 9673.0, 11261.0, 10484.0, 12601.0, 9209.0, 10775.0, 8458.0, 9636.0, 8578.0, 8664.0, 7312.0, 8866.0, 9439.0, 9688.0, 9647.0, 11576.0, 10342.0, 9848.0, 9477.0, 8509.0, 5996.0, 4200.0, 2226.0, 953.0, 568.0, 508.0, 564.0, 418.0, 182.0, 131.0, 75.0, 73.0, 58.0, 68.0, 60.0, 71.0, 47.0, 48.0], [42.0, 47.0, 51.0, 67.0, 56.0, 68.0, 77.0, 84.0, 98.0, 115.0, 161.0, 435.0, 556.0, 692.0, 651.0, 1576.0, 2829.0, 5330.0, 7306.0, 9302.0, 9449.0, 11048.0, 11300.0, 10199.0, 9591.0, 10788.0, 8537.0, 9401.0, 7582.0, 9159.0, 8741.0, 9162.0, 8699.0, 10636.0, 9557.0, 11188.0, 10228.0, 10533.0, 8555.0, 8375.0, 5317.0, 4788.0, 2010.0, 1135.0, 537.0, 533.0, 514.0, 429.0, 201.0, 97.0, 87.0, 82.0, 62.0, 59.0, 64.0, 53.0, 37.0, 50.0], [56.0, 49.0, 51.0, 54.0, 46.0, 66.0, 84.0, 72.0, 107.0, 109.0, 170.0, 388.0, 666.0, 689.0, 640.0, 1497.0, 2682.0, 4445.0, 6921.0, 8754.0, 9673.0, 10935.0, 10284.0, 12081.0, 10816.0, 8302.0, 9237.0, 8724.0, 8346.0, 8661.0, 8143.0, 9239.0, 7785.0, 11724.0, 10079.0, 11161.0, 10442.0, 10239.0, 9468.0, 8466.0, 6283.0, 3993.0, 2110.0, 1047.0, 489.0, 552.0, 444.0, 403.0, 165.0, 112.0, 66.0, 95.0, 82.0, 74.0, 57.0, 48.0, 58.0, 50.0], [38.0, 50.0, 56.0, 48.0, 51.0, 83.0, 74.0, 71.0, 100.0, 106.0, 131.0, 487.0, 624.0, 578.0, 632.0, 1331.0, 2348.0, 5123.0, 6363.0, 9618.0, 10251.0, 11205.0, 10673.0, 9881.0, 10275.0, 10829.0, 9525.0, 9291.0, 8776.0, 8677.0, 9635.0, 8839.0, 9459.0, 10159.0, 10375.0, 10090.0, 10258.0, 11294.0, 7956.0, 7766.0, 5540.0, 3937.0, 2146.0, 979.0, 541.0, 564.0, 467.0, 397.0, 163.0, 98.0, 95.0, 73.0, 59.0, 56.0, 49.0, 56.0, 56.0, 52.0], [53.0, 48.0, 50.0, 58.0, 49.0, 72.0, 82.0, 79.0, 96.0, 126.0, 148.0, 441.0, 641.0, 727.0, 631.0, 1199.0, 2285.0, 4363.0, 5668.0, 8397.0, 9341.0, 11147.0, 9546.0, 12554.0, 9382.0, 11001.0, 9028.0, 10103.0, 9116.0, 9364.0, 8492.0, 10029.0, 10127.0, 10158.0, 10380.0, 12645.0, 10069.0, 9863.0, 9348.0, 7347.0, 5340.0, 3245.0, 1729.0, 911.0, 462.0, 536.0, 464.0, 363.0, 179.0, 121.0, 86.0, 96.0, 69.0, 52.0, 57.0, 57.0, 69.0, 63.0], [34.0, 40.0, 39.0, 60.0, 47.0, 50.0, 57.0, 77.0, 92.0, 105.0, 169.0, 287.0, 574.0, 652.0, 690.0, 914.0, 1669.0, 4028.0, 5906.0, 7922.0, 9101.0, 10821.0, 10025.0, 11720.0, 10376.0, 10554.0, 10586.0, 10705.0, 9206.0, 11048.0, 9519.0, 10771.0, 9911.0, 12018.0, 10443.0, 10433.0, 11653.0, 10868.0, 8273.0, 7042.0, 4676.0, 2944.0, 1433.0, 593.0, 514.0, 541.0, 468.0, 282.0, 135.0, 125.0, 66.0, 85.0, 59.0, 66.0, 60.0, 58.0, 47.0, 54.0], [51.0, 52.0, 57.0, 56.0, 58.0, 73.0, 79.0, 83.0, 97.0, 136.0, 132.0, 237.0, 519.0, 733.0, 601.0, 845.0, 1840.0, 2764.0, 4580.0, 7601.0, 7562.0, 10524.0, 11102.0, 10016.0, 11428.0, 11043.0, 10909.0, 10769.0, 10238.0, 11295.0, 9110.0, 10794.0, 10497.0, 10654.0, 11055.0, 11282.0, 9897.0, 9114.0, 7534.0, 5939.0, 3893.0, 2242.0, 992.0, 649.0, 490.0, 528.0, 496.0, 308.0, 126.0, 104.0, 72.0, 76.0, 60.0, 60.0, 53.0, 56.0, 47.0, 54.0], [43.0, 35.0, 48.0, 63.0, 40.0, 77.0, 54.0, 78.0, 90.0, 100.0, 117.0, 161.0, 410.0, 707.0, 630.0, 739.0, 1027.0, 2298.0, 3802.0, 5938.0, 7937.0, 9245.0, 10375.0, 11695.0, 11033.0, 12197.0, 10987.0, 11483.0, 9671.0, 12701.0, 10444.0, 10946.0, 10194.0, 11417.0, 10817.0, 11476.0, 9498.0, 9417.0, 6847.0, 5308.0, 3092.0, 2008.0, 804.0, 572.0, 471.0, 563.0, 379.0, 185.0, 109.0, 110.0, 82.0, 74.0, 54.0, 74.0, 64.0, 43.0, 48.0, 47.0], [35.0, 55.0, 61.0, 54.0, 40.0, 69.0, 60.0, 88.0, 77.0, 91.0, 124.0, 140.0, 270.0, 572.0, 608.0, 650.0, 923.0, 1902.0, 3019.0, 4467.0, 6238.0, 8118.0, 9530.0, 10343.0, 9223.0, 10723.0, 10817.0, 11322.0, 11405.0, 10575.0, 10430.0, 10470.0, 9932.0, 11697.0, 10439.0, 9469.0, 8598.0, 7635.0, 5353.0, 4215.0, 2470.0, 1065.0, 573.0, 568.0, 486.0, 537.0, 290.0, 162.0, 91.0, 77.0, 55.0, 70.0, 60.0, 52.0, 53.0, 48.0, 40.0, 59.0], [41.0, 44.0, 41.0, 53.0, 56.0, 56.0, 59.0, 80.0, 61.0, 79.0, 134.0, 110.0, 181.0, 494.0, 613.0, 742.0, 678.0, 1135.0, 2028.0, 4297.0, 4499.0, 7335.0, 7649.0, 9582.0, 10180.0, 10280.0, 10322.0, 11392.0, 9819.0, 12281.0, 9843.0, 11415.0, 10346.0, 10653.0, 9376.0, 9128.0, 6831.0, 6725.0, 3861.0, 2944.0, 1609.0, 906.0, 477.0, 543.0, 513.0, 464.0, 179.0, 120.0, 79.0, 75.0, 45.0, 69.0, 49.0, 65.0, 42.0, 61.0, 37.0, 0.0], [35.0, 45.0, 42.0, 43.0, 44.0, 70.0, 53.0, 77.0, 82.0, 92.0, 98.0, 152.0, 129.0, 305.0, 625.0, 605.0, 565.0, 840.0, 1300.0, 2254.0, 3353.0, 5065.0, 5744.0, 8587.0, 7931.0, 10381.0, 9591.0, 10643.0, 10156.0, 10030.0, 9592.0, 9943.0, 9054.0, 9449.0, 8537.0, 7544.0, 5516.0, 5096.0, 3177.0, 1886.0, 923.0, 666.0, 478.0, 520.0, 511.0, 320.0, 111.0, 101.0, 75.0, 52.0, 49.0, 53.0, 36.0, 51.0, 52.0, 47.0, 33.0, 0.0], [33.0, 33.0, 52.0, 41.0, 61.0, 54.0, 70.0, 69.0, 65.0, 85.0, 79.0, 122.0, 128.0, 219.0, 396.0, 677.0, 674.0, 667.0, 707.0, 1548.0, 2286.0, 3904.0, 4771.0, 5936.0, 6956.0, 8090.0, 8053.0, 8551.0, 8651.0, 8738.0, 8203.0, 9152.0, 7729.0, 8324.0, 5988.0, 5881.0, 4193.0, 2926.0, 1852.0, 1151.0, 644.0, 545.0, 495.0, 539.0, 397.0, 211.0, 102.0, 90.0, 55.0, 54.0, 45.0, 53.0, 48.0, 47.0, 32.0, 38.0, 38.0, 0.0], [0.0, 35.0, 45.0, 56.0, 44.0, 57.0, 57.0, 72.0, 47.0, 81.0, 72.0, 106.0, 127.0, 172.0, 254.0, 616.0, 598.0, 644.0, 714.0, 803.0, 1287.0, 2146.0, 2959.0, 4334.0, 4545.0, 5643.0, 6271.0, 6953.0, 6924.0, 7309.0, 7110.0, 6573.0, 6314.0, 5274.0, 4505.0, 4247.0, 2943.0, 1888.0, 1122.0, 712.0, 510.0, 571.0, 577.0, 520.0, 197.0, 128.0, 82.0, 91.0, 60.0, 48.0, 31.0, 39.0, 36.0, 34.0, 37.0, 43.0, 0.0, 0.0], [0.0, 36.0, 32.0, 40.0, 39.0, 46.0, 50.0, 79.0, 72.0, 64.0, 93.0, 78.0, 95.0, 122.0, 156.0, 307.0, 650.0, 651.0, 578.0, 665.0, 855.0, 1191.0, 1694.0, 2565.0, 2926.0, 4053.0, 4058.0, 5371.0, 5037.0, 5109.0, 5581.0, 5156.0, 3810.0, 4174.0, 2897.0, 2132.0, 1192.0, 1035.0, 592.0, 492.0, 514.0, 591.0, 500.0, 359.0, 164.0, 98.0, 48.0, 58.0, 38.0, 35.0, 59.0, 45.0, 31.0, 42.0, 37.0, 35.0, 0.0, 0.0], [0.0, 36.0, 39.0, 47.0, 50.0, 57.0, 63.0, 45.0, 67.0, 60.0, 91.0, 81.0, 90.0, 131.0, 118.0, 140.0, 322.0, 567.0, 628.0, 612.0, 629.0, 783.0, 803.0, 1296.0, 1638.0, 2460.0, 2366.0, 3165.0, 3047.0, 3183.0, 2693.0, 2719.0, 2300.0, 2181.0, 1444.0, 1227.0, 807.0, 669.0, 508.0, 621.0, 516.0, 524.0, 320.0, 171.0, 82.0, 85.0, 48.0, 51.0, 40.0, 48.0, 37.0, 45.0, 31.0, 41.0, 36.0, 23.0, 0.0, 0.0], [0.0, 0.0, 36.0, 29.0, 50.0, 50.0, 43.0, 56.0, 53.0, 60.0, 56.0, 53.0, 76.0, 82.0, 97.0, 138.0, 157.0, 323.0, 556.0, 684.0, 618.0, 611.0, 638.0, 759.0, 865.0, 913.0, 1174.0, 1369.0, 1400.0, 1638.0, 1478.0, 1471.0, 1090.0, 989.0, 750.0, 610.0, 522.0, 547.0, 634.0, 596.0, 453.0, 332.0, 129.0, 83.0, 44.0, 56.0, 37.0, 51.0, 30.0, 43.0, 31.0, 35.0, 36.0, 38.0, 13.0, 0.0, 0.0, 0.0], [0.0, 0.0, 0.0, 42.0, 41.0, 41.0, 47.0, 59.0, 59.0, 59.0, 53.0, 71.0, 73.0, 72.0, 90.0, 94.0, 126.0, 155.0, 250.0, 543.0, 638.0, 707.0, 619.0, 522.0, 643.0, 658.0, 652.0, 685.0, 733.0, 772.0, 714.0, 760.0, 615.0, 616.0, 538.0, 596.0, 580.0, 676.0, 522.0, 543.0, 276.0, 154.0, 81.0, 64.0, 53.0, 43.0, 43.0, 45.0, 34.0, 31.0, 30.0, 33.0, 27.0, 27.0, 0.0, 0.0, 0.0, 0.0], [0.0, 0.0, 0.0, 46.0, 36.0, 62.0, 44.0, 47.0, 66.0, 55.0, 56.0, 68.0, 51.0, 59.0, 71.0, 80.0, 114.0, 116.0, 138.0, 195.0, 379.0, 646.0, 707.0, 664.0, 696.0, 624.0, 665.0, 603.0, 596.0, 570.0, 608.0, 539.0, 555.0, 615.0, 635.0, 690.0, 555.0, 567.0, 389.0, 243.0, 123.0, 80.0, 71.0, 57.0, 59.0, 52.0, 37.0, 31.0, 27.0, 38.0, 24.0, 27.0, 22.0, 31.0, 0.0, 0.0, 0.0, 0.0], [0.0, 0.0, 0.0, 0.0, 46.0, 43.0, 53.0, 48.0, 52.0, 53.0, 61.0, 59.0, 52.0, 56.0, 68.0, 86.0, 95.0, 105.0, 130.0, 185.0, 180.0, 274.0, 489.0, 576.0, 656.0, 737.0, 605.0, 706.0, 594.0, 777.0, 622.0, 730.0, 692.0, 719.0, 528.0, 570.0, 490.0, 387.0, 178.0, 119.0, 106.0, 77.0, 46.0, 59.0, 47.0, 48.0, 32.0, 34.0, 31.0, 34.0, 24.0, 18.0, 19.0, 0.0, 0.0, 0.0, 0.0, 0.0], [0.0, 0.0, 0.0, 0.0, 0.0, 44.0, 41.0, 55.0, 51.0, 50.0, 49.0, 41.0, 54.0, 57.0, 76.0, 76.0, 94.0, 92.0, 100.0, 112.0, 141.0, 157.0, 225.0, 222.0, 315.0, 453.0, 537.0, 594.0, 559.0, 612.0, 584.0, 489.0, 498.0, 452.0, 340.0, 260.0, 172.0, 168.0, 90.0, 105.0, 62.0, 75.0, 39.0, 44.0, 41.0, 34.0, 31.0, 28.0, 27.0, 26.0, 19.0, 31.0, 0.0, 0.0, 0.0, 0.0, 0.0, 0.0], [0.0, 0.0, 0.0, 0.0, 0.0, 45.0, 59.0, 35.0, 34.0, 51.0, 57.0, 50.0, 49.0, 63.0, 47.0, 58.0, 69.0, 103.0, 101.0, 109.0, 127.0, 134.0, 163.0, 142.0, 176.0, 169.0, 185.0, 224.0, 268.0, 360.0, 300.0, 285.0, 179.0, 171.0, 122.0, 149.0, 139.0, 117.0, 94.0, 81.0, 66.0, 49.0, 42.0, 50.0, 33.0, 41.0, 26.0, 31.0, 18.0, 30.0, 24.0, 30.0, 0.0, 0.0, 0.0, 0.0, 0.0, 0.0], [0.0, 0.0, 0.0, 0.0, 0.0, 0.0, 51.0, 53.0, 49.0, 50.0, 33.0, 39.0, 41.0, 52.0, 76.0, 55.0, 69.0, 81.0, 76.0, 105.0, 107.0, 124.0, 139.0, 148.0, 130.0, 173.0, 166.0, 170.0, 178.0, 189.0, 143.0, 141.0, 141.0, 116.0, 144.0, 115.0, 92.0, 89.0, 73.0, 76.0, 58.0, 46.0, 33.0, 45.0, 35.0, 37.0, 22.0, 29.0, 29.0, 27.0, 29.0, 0.0, 0.0, 0.0, 0.0, 0.0, 0.0, 0.0], [0.0, 0.0, 0.0, 0.0, 0.0, 0.0, 0.0, 50.0, 40.0, 53.0, 53.0, 42.0, 41.0, 48.0, 54.0, 65.0, 62.0, 73.0, 92.0, 86.0, 116.0, 94.0, 127.0, 90.0, 154.0, 116.0, 114.0, 125.0, 122.0, 144.0, 124.0, 148.0, 115.0, 118.0, 101.0, 82.0, 103.0, 87.0, 72.0, 54.0, 57.0, 43.0, 41.0, 25.0, 35.0, 26.0, 30.0, 25.0, 27.0, 22.0, 0.0, 0.0, 0.0, 0.0, 0.0, 0.0, 0.0, 0.0], [0.0, 0.0, 0.0, 0.0, 0.0, 0.0, 0.0, 0.0, 41.0, 43.0, 50.0, 38.0, 51.0, 60.0, 53.0, 73.0, 51.0, 58.0, 92.0, 63.0, 95.0, 98.0, 113.0, 118.0, 113.0, 113.0, 105.0, 119.0, 108.0, 109.0, 114.0, 89.0, 83.0, 114.0, 98.0, 93.0, 97.0, 79.0, 56.0, 54.0, 43.0, 54.0, 48.0, 35.0, 30.0, 39.0, 32.0, 29.0, 27.0, 0.0, 0.0, 0.0, 0.0, 0.0, 0.0, 0.0, 0.0, 0.0], [0.0, 0.0, 0.0, 0.0, 0.0, 0.0, 0.0, 0.0, 0.0, 50.0, 46.0, 61.0, 60.0, 64.0, 46.0, 51.0, 55.0, 68.0, 57.0, 80.0, 76.0, 86.0, 91.0, 86.0, 93.0, 107.0, 97.0, 107.0, 109.0, 105.0, 85.0, 98.0, 84.0, 95.0, 64.0, 86.0, 70.0, 74.0, 40.0, 61.0, 63.0, 39.0, 46.0, 37.0, 34.0, 37.0, 26.0, 18.0, 0.0, 0.0, 0.0, 0.0, 0.0, 0.0, 0.0, 0.0, 0.0, 0.0], [0.0, 0.0, 0.0, 0.0, 0.0, 0.0, 0.0, 0.0, 0.0, 0.0, 0.0, 40.0, 52.0, 44.0, 58.0, 37.0, 61.0, 65.0, 61.0, 84.0, 90.0, 73.0, 81.0, 76.0, 75.0, 84.0, 84.0, 75.0, 76.0, 83.0, 83.0, 83.0, 85.0, 79.0, 71.0, 65.0, 46.0, 71.0, 64.0, 43.0, 56.0, 36.0, 42.0, 30.0, 23.0, 21.0, 0.0, 0.0, 0.0, 0.0, 0.0, 0.0, 0.0, 0.0, 0.0, 0.0, 0.0, 0.0], [0.0, 0.0, 0.0, 0.0, 0.0, 0.0, 0.0, 0.0, 0.0, 0.0, 0.0, 0.0, 59.0, 44.0, 50.0, 44.0, 72.0, 63.0, 64.0, 70.0, 90.0, 68.0, 97.0, 68.0, 72.0, 101.0, 75.0, 76.0, 72.0, 84.0, 76.0, 79.0, 64.0, 73.0, 82.0, 73.0, 49.0, 63.0, 46.0, 51.0, 25.0, 41.0, 32.0, 35.0, 31.0, 0.0, 0.0, 0.0, 0.0, 0.0, 0.0, 0.0, 0.0, 0.0, 0.0, 0.0, 0.0, 0.0], [0.0, 0.0, 0.0, 0.0, 0.0, 0.0, 0.0, 0.0, 0.0, 0.0, 0.0, 0.0, 0.0, 0.0, 37.0, 48.0, 47.0, 50.0, 60.0, 76.0, 72.0, 68.0, 79.0, 68.0, 71.0, 70.0, 72.0, 65.0, 73.0, 55.0, 83.0, 93.0, 73.0, 57.0, 62.0, 48.0, 60.0, 58.0, 47.0, 37.0, 42.0, 37.0, 25.0, 0.0, 0.0, 0.0, 0.0, 0.0, 0.0, 0.0, 0.0, 0.0, 0.0, 0.0, 0.0, 0.0, 0.0, 0.0], [0.0, 0.0, 0.0, 0.0, 0.0, 0.0, 0.0, 0.0, 0.0, 0.0, 0.0, 0.0, 0.0, 0.0, 0.0, 47.0, 42.0, 60.0, 72.0, 84.0, 69.0, 88.0, 71.0, 67.0, 68.0, 76.0, 66.0, 68.0, 58.0, 71.0, 69.0, 47.0, 49.0, 78.0, 49.0, 56.0, 46.0, 59.0, 27.0, 43.0, 40.0, 35.0, 0.0, 0.0, 0.0, 0.0, 0.0, 0.0, 0.0, 0.0, 0.0, 0.0, 0.0, 0.0, 0.0, 0.0, 0.0, 0.0], [0.0, 0.0, 0.0, 0.0, 0.0, 0.0, 0.0, 0.0, 0.0, 0.0, 0.0, 0.0, 0.0, 0.0, 0.0, 0.0, 0.0, 0.0, 43.0, 55.0, 75.0, 55.0, 70.0, 69.0, 73.0, 54.0, 70.0, 65.0, 65.0, 51.0, 82.0, 50.0, 70.0, 63.0, 49.0, 75.0, 45.0, 58.0, 35.0, 0.0, 0.0, 0.0, 0.0, 0.0, 0.0, 0.0, 0.0, 0.0, 0.0, 0.0, 0.0, 0.0, 0.0, 0.0, 0.0, 0.0, 0.0, 0.0], [0.0, 0.0, 0.0, 0.0, 0.0, 0.0, 0.0, 0.0, 0.0, 0.0, 0.0, 0.0, 0.0, 0.0, 0.0, 0.0, 0.0, 0.0, 0.0, 0.0, 0.0, 68.0, 59.0, 57.0, 48.0, 67.0, 50.0, 49.0, 69.0, 51.0, 53.0, 73.0, 68.0, 57.0, 70.0, 39.0, 0.0, 0.0, 0.0, 0.0, 0.0, 0.0, 0.0, 0.0, 0.0, 0.0, 0.0, 0.0, 0.0, 0.0, 0.0, 0.0, 0.0, 0.0, 0.0, 0.0, 0.0, 0.0]]
  out "Idler Bck":dbl[][](graph)=[[0.0, 0.0, 0.0, 0.0, 0.0, 0.0, 0.0, 0.0, 0.0, 0.0, 0.0, 0.0, 0.0, 0.0, 0.0, 0.0, 0.0, 0.0, 27.0, 38.0, 29.0, 31.0, 36.0, 36.0, 33.0, 42.0, 34.0, 31.0, 35.0, 29.0, 34.0, 20.0, 43.0, 34.0, 20.0, 35.0, 37.0, 43.0, 23.0, 0.0, 0.0, 0.0, 0.0, 0.0, 0.0, 0.0, 0.0, 0.0, 0.0, 0.0, 0.0, 0.0, 0.0, 0.0, 0.0, 0.0, 0.0, 0.0], [0.0, 0.0, 0.0, 0.0, 0.0, 0.0, 0.0, 0.0, 0.0, 0.0, 0.0, 0.0, 0.0, 0.0, 0.0, 30.0, 26.0, 24.0, 35.0, 36.0, 36.0, 27.0, 32.0, 33.0, 47.0, 30.0, 27.0, 33.0, 32.0, 34.0, 36.0, 40.0, 41.0, 38.0, 26.0, 27.0, 37.0, 32.0, 38.0, 40.0, 24.0, 44.0, 0.0, 0.0, 0.0, 0.0, 0.0, 0.0, 0.0, 0.0, 0.0, 0.0, 0.0, 0.0, 0.0, 0.0, 0.0, 0.0], [0.0, 0.0, 0.0, 0.0, 0.0, 0.0, 0.0, 0.0, 0.0, 0.0, 0.0, 0.0, 0.0, 0.0, 30.0, 26.0, 30.0, 31.0, 27.0, 25.0, 30.0, 25.0, 36.0, 41.0, 26.0, 30.0, 49.0, 29.0, 50.0, 41.0, 32.0, 36.0, 41.0, 34.0, 27.0, 32.0, 36.0, 28.0, 31.0, 41.0, 27.0, 29.0, 33.0, 0.0, 0.0, 0.0, 0.0, 0.0, 0.0, 0.0, 0.0, 0.0, 0.0, 0.0, 0.0, 0.0, 0.0, 0.0], [0.0, 0.0, 0.0, 0.0, 0.0, 0.0, 0.0, 0.0, 0.0, 0.0, 0.0, 0.0, 30.0, 25.0, 19.0, 31.0, 26.0, 28.0, 24.0, 29.0, 28.0, 30.0, 35.0, 22.0, 36.0, 37.0, 40.0, 35.0, 37.0, 35.0, 31.0, 38.0, 33.0, 30.0, 51.0, 30.0, 24.0, 30.0, 14.0, 42.0, 35.0, 32.0, 32.0, 44.0, 27.0, 0.0, 0.0, 0.0, 0.0, 0.0, 0.0, 0.0, 0.0, 0.0, 0.0, 0.0, 0.0, 0.0], [0.0, 0.0, 0.0, 0.0, 0.0, 0.0, 0.0, 0.0, 0.0, 0.0, 0.0, 31.0, 24.0, 30.0, 18.0, 24.0, 27.0, 29.0, 30.0, 46.0, 30.0, 31.0, 37.0, 40.0, 38.0, 36.0, 38.0, 55.0, 30.0, 38.0, 49.0, 43.0, 35.0, 47.0, 28.0, 45.0, 32.0, 40.0, 30.0, 41.0, 26.0, 35.0, 33.0, 40.0, 34.0, 27.0, 0.0, 0.0, 0.0, 0.0, 0.0, 0.0, 0.0, 0.0, 0.0, 0.0, 0.0, 0.0], [0.0, 0.0, 0.0, 0.0, 0.0, 0.0, 0.0, 0.0, 0.0, 22.0, 22.0, 22.0, 29.0, 21.0, 24.0, 32.0, 32.0, 21.0, 38.0, 28.0, 40.0, 40.0, 37.0, 35.0, 20.0, 45.0, 32.0, 29.0, 35.0, 44.0, 31.0, 41.0, 29.0, 38.0, 28.0, 32.0, 31.0, 38.0, 31.0, 35.0, 28.0, 35.0, 24.0, 30.0, 36.0, 33.0, 23.0, 31.0, 0.0, 0.0, 0.0, 0.0, 0.0, 0.0, 0.0, 0.0, 0.0, 0.0], [0.0, 0.0, 0.0, 0.0, 0.0, 0.0, 0.0, 0.0, 15.0, 30.0, 28.0, 24.0, 34.0, 34.0, 20.0, 41.0, 28.0, 26.0, 39.0, 29.0, 38.0, 25.0, 19.0, 45.0, 35.0, 26.0, 35.0, 35.0, 40.0, 33.0, 35.0, 37.0, 41.0, 33.0, 35.0, 45.0, 37.0, 36.0, 33.0, 40.0, 27.0, 37.0, 34.0, 30.0, 31.0, 27.0, 27.0, 31.0, 24.0, 0.0, 0.0, 0.0, 0.0, 0.0, 0.0, 0.0, 0.0, 0.0], [0.0, 0.0, 0.0, 0.0, 0.0, 0.0, 0.0, 22.0, 23.0, 25.0, 30.0, 27.0, 31.0, 28.0, 30.0, 24.0, 25.0, 43.0, 22.0, 42.0, 29.0, 49.0, 42.0, 40.0, 39.0, 37.0, 51.0, 33.0, 46.0, 40.0, 44.0, 40.0, 38.0, 41.0, 39.0, 50.0, 30.0, 35.0, 42.0, 34.0, 29.0, 28.0, 32.0, 28.0, 27.0, 44.0, 24.0, 39.0, 35.0, 32.0, 0.0, 0.0, 0.0, 0.0, 0.0, 0.0, 0.0, 0.0], [0.0, 0.0, 0.0, 0.0, 0.0, 0.0, 27.0, 34.0, 29.0, 22.0, 24.0, 25.0, 34.0, 38.0, 36.0, 36.0, 21.0, 31.0, 27.0, 32.0, 46.0, 42.0, 36.0, 48.0, 45.0, 37.0, 62.0, 49.0, 56.0, 51.0, 53.0, 32.0, 41.0, 37.0, 39.0, 34.0, 34.0, 29.0, 35.0, 29.0, 43.0, 39.0, 35.0, 36.0, 26.0, 32.0, 29.0, 33.0, 24.0, 35.0, 29.0, 0.0, 0.0, 0.0, 0.0, 0.0, 0.0, 0.0], [0.0, 0.0, 0.0, 0.0, 0.0, 32.0, 24.0, 23.0, 35.0, 28.0, 27.0, 24.0, 20.0, 29.0, 24.0, 30.0, 27.0, 52.0, 30.0, 44.0, 23.0, 54.0, 42.0, 41.0, 59.0, 57.0, 62.0, 82.0, 98.0, 89.0, 94.0, 100.0, 98.0, 60.0, 62.0, 38.0, 51.0, 37.0, 42.0, 35.0, 37.0, 58.0, 26.0, 35.0, 29.0, 32.0, 30.0, 35.0, 36.0, 38.0, 33.0, 35.0, 0.0, 0.0, 0.0, 0.0, 0.0, 0.0], [0.0, 0.0, 0.0, 0.0, 0.0, 29.0, 23.0, 27.0, 28.0, 24.0, 23.0, 39.0, 34.0, 21.0, 20.0, 37.0, 21.0, 39.0, 40.0, 32.0, 38.0, 44.0, 62.0, 67.0, 88.0, 130.0, 169.0, 160.0, 126.0, 178.0, 151.0, 140.0, 141.0, 145.0, 130.0, 111.0, 81.0, 70.0, 44.0, 45.0, 32.0, 24.0, 31.0, 47.0, 35.0, 32.0, 31.0, 42.0, 25.0, 25.0, 18.0, 32.0, 0.0, 0.0, 0.0, 0.0, 0.0, 0.0], [0.0, 0.0, 0.0, 0.0, 20.0, 26.0, 27.0, 18.0, 22.0, 26.0, 20.0, 23.0, 22.0, 28.0, 25.0, 34.0, 36.0, 42.0, 33.0, 48.0, 60.0, 81.0, 156.0, 133.0, 204.0, 180.0, 169.0, 158.0, 192.0, 139.0, 197.0, 181.0, 172.0, 157.0, 183.0, 176.0, 141.0, 115.0, 79.0, 51.0, 32.0, 42.0, 26.0, 45.0, 47.0, 35.0, 45.0, 31.0, 31.0, 29.0, 32.0, 35.0, 29.0, 0.0, 0.0, 0.0, 0.0, 0.0], [0.0, 0.0, 0.0, 17.0, 19.0, 24.0, 27.0, 27.0, 22.0, 35.0, 28.0, 27.0, 23.0, 38.0, 29.0, 34.0, 35.0, 24.0, 38.0, 54.0, 108.0, 181.0, 162.0, 176.0, 149.0, 171.0, 165.0, 161.0, 159.0, 208.0, 131.0, 166.0, 177.0, 151.0, 161.0, 171.0, 179.0, 148.0, 130.0, 112.0, 50.0, 42.0, 27.0, 40.0, 24.0, 38.0, 24.0, 36.0, 31.0, 31.0, 35.0, 23.0, 31.0, 19.0, 0.0, 0.0, 0.0, 0.0], [0.0, 0.0, 0.0, 25.0, 24.0, 19.0, 26.0, 22.0, 25.0, 21.0, 33.0, 25.0, 32.0, 34.0, 33.0, 33.0, 55.0, 52.0, 83.0, 146.0, 186.0, 212.0, 182.0, 161.0, 180.0, 192.0, 202.0, 260.0, 244.0, 279.0, 209.0, 238.0, 192.0, 219.0, 150.0, 143.0, 124.0, 159.0, 139.0, 155.0, 114.0, 79.0, 52.0, 39.0, 46.0, 37.0, 41.0, 30.0, 25.0, 34.0, 24.0, 31.0, 19.0, 28.0, 0.0, 0.0, 0.0, 0.0], [0.0, 0.0, 20.0, 18.0, 26.0, 28.0, 25.0, 22.0, 32.0, 27.0, 26.0, 22.0, 28.0, 23.0, 43.0, 41.0, 56.0, 95.0, 156.0, 168.0, 192.0, 142.0, 207.0, 204.0, 271.0, 279.0, 361.0, 430.0, 439.0, 467.0, 394.0, 413.0, 347.0, 319.0, 233.0, 193.0, 164.0, 168.0, 117.0, 158.0, 145.0, 126.0, 63.0, 38.0, 34.0, 27.0, 27.0, 22.0, 24.0, 38.0, 25.0, 33.0, 31.0, 28.0, 29.0, 0.0, 0.0, 0.0], [0.0, 27.0, 28.0, 29.0, 25.0, 35.0, 21.0, 21.0, 35.0, 34.0, 25.0, 24.0, 32.0, 32.0, 38.0, 38.0, 100.0, 175.0, 178.0, 200.0, 203.0, 239.0, 286.0, 371.0, 486.0, 515.0, 730.0, 698.0, 772.0, 729.0, 856.0, 759.0, 606.0, 474.0, 475.0, 326.0, 228.0, 199.0, 171.0, 162.0, 165.0, 141.0, 137.0, 85.0, 49.0, 43.0, 23.0, 35.0, 30.0, 29.0, 31.0, 24.0, 44.0, 23.0, 37.0, 33.0, 0.0, 0.0], [0.0, 25.0, 34.0, 25.0, 26.0, 20.0, 18.0, 23.0, 22.0, 22.0, 34.0, 30.0, 28.0, 54.0, 42.0, 129.0, 139.0, 189.0, 139.0, 187.0, 215.0, 348.0, 463.0, 553.0, 800.0, 1039.0, 1031.0, 1075.0, 1236.0, 1573.0, 1372.0, 1196.0, 1046.0, 792.0, 668.0, 510.0, 406.0, 259.0, 176.0, 163.0, 137.0, 184.0, 109.0, 121.0, 76.0, 46.0, 38.0, 40.0, 33.0, 29.0, 39.0, 24.0, 33.0, 34.0, 28.0, 31.0, 0.0, 0.0], [0.0, 19.0, 21.0, 29.0, 14.0, 26.0, 32.0, 32.0, 30.0, 28.0, 41.0, 38.0, 28.0, 71.0, 82.0, 156.0, 180.0, 205.0, 185.0, 274.0, 391.0, 487.0, 841.0, 1017.0, 1173.0, 1437.0, 1549.0, 1493.0, 1617.0, 1568.0, 1749.0, 1544.0, 1255.0, 1368.0, 1083.0, 903.0, 628.0, 488.0, 334.0, 180.0, 156.0, 130.0, 123.0, 141.0, 116.0, 81.0, 37.0, 35.0, 26.0, 28.0, 33.0, 20.0, 28.0, 22.0, 35.0, 28.0, 0.0, 0.0], [19.0, 20.0, 29.0, 28.0, 29.0, 22.0, 24.0, 29.0, 24.0, 32.0, 32.0, 33.0, 43.0, 56.0, 131.0, 204.0, 180.0, 179.0, 254.0, 433.0, 582.0, 872.0, 1089.0, 1567.0, 1478.0, 1623.0, 1730.0, 2117.0, 1800.0, 1882.0, 1663.0, 1778.0, 1706.0, 1633.0, 1422.0, 1095.0, 1092.0, 674.0, 431.0, 306.0, 170.0, 164.0, 158.0, 153.0, 123.0, 106.0, 75.0, 41.0, 27.0, 36.0, 33.0, 21.0, 38.0, 25.0, 24.0, 32.0, 29.0, 0.0], [20.0, 25.0, 22.0, 21.0, 18.0, 28.0, 27.0, 20.0, 27.0, 34.0, 31.0, 30.0, 55.0, 123.0, 168.0, 167.0, 252.0, 251.0, 343.0, 525.0, 800.0, 1099.0, 961.0, 1910.0, 1829.0, 2236.0, 2054.0, 2177.0, 2093.0, 2103.0, 2217.0, 2192.0, 2153.0, 1759.0, 1688.0, 1530.0, 1149.0, 970.0, 768.0, 408.0, 340.0, 189.0, 131.0, 163.0, 148.0, 114.0, 71.0, 43.0, 28.0, 42.0, 24.0, 28.0, 29.0, 40.0, 25.0, 29.0, 28.0, 0.0], [26.0, 28.0, 16.0, 28.0, 35.0, 29.0, 17.0, 21.0, 31.0, 20.0, 29.0, 48.0, 78.0, 132.0, 182.0, 179.0, 184.0, 306.0, 598.0, 772.0, 1067.0, 1532.0, 2844.0, 1519.0, 2061.0, 2327.0, 2280.0, 2087.0, 2302.0, 2333.0, 2139.0, 1836.0, 2473.0, 2037.0, 2076.0, 1961.0, 1509.0, 1291.0, 929.0, 662.0, 372.0, 230.0, 151.0, 124.0, 147.0, 122.0, 84.0, 63.0, 34.0, 35.0, 32.0, 26.0, 29.0, 39.0, 34.0, 31.0, 25.0, 0.0], [31.0, 19.0, 20.0, 14.0, 27.0, 22.0, 28.0, 26.0, 33.0, 33.0, 61.0, 36.0, 85.0, 172.0, 161.0, 222.0, 246.0, 486.0, 688.0, 1048.0, 1450.0, 1556.0, 1886.0, 1989.0, 2619.0, 2136.0, 2218.0, 2662.0, 2487.0, 2072.0, 2559.0, 2180.0, 2583.0, 2128.0, 2190.0, 2010.0, 1555.0, 1538.0, 1112.0, 801.0, 542.0, 324.0, 171.0, 141.0, 118.0, 148.0, 111.0, 76.0, 29.0, 27.0, 27.0, 24.0, 20.0, 40.0, 25.0, 25.0, 25.0, 20.0], [11.0, 29.0, 31.0, 20.0, 19.0, 27.0, 32.0, 33.0, 24.0, 37.0, 44.0, 45.0, 129.0, 172.0, 184.0, 235.0, 330.0, 587.0, 832.0, 1540.0, 1821.0, 1929.0, 2287.0, 2341.0, 2123.0, 2432.0, 2285.0, 2151.0, 2207.0, 2437.0, 2365.0, 2013.0, 2165.0, 2112.0, 2103.0, 2447.0, 1852.0, 1797.0, 1392.0, 1064.0, 669.0, 363.0, 226.0, 174.0, 148.0, 145.0, 117.0, 78.0, 57.0, 36.0, 23.0, 29.0, 25.0, 35.0, 33.0, 29.0, 24.0, 23.0], [28.0, 15.0, 29.0, 20.0, 24.0, 27.0, 17.0, 20.0, 32.0, 45.0, 44.0, 95.0, 166.0, 187.0, 192.0, 271.0, 554.0, 693.0, 1186.0, 1393.0, 1694.0, 2419.0, 2074.0, 2230.0, 2226.0, 2527.0, 2229.0, 2016.0, 2271.0, 2134.0, 2051.0, 2302.0, 2219.0, 2117.0, 2379.0, 1952.0, 2025.0, 1963.0, 1572.0, 1276.0, 864.0, 565.0, 278.0, 178.0, 145.0, 154.0, 125.0, 97.0, 48.0, 41.0, 30.0, 36.0, 24.0, 22.0, 26.0, 36.0, 21.0, 37.0], [21.0, 28.0, 13.0, 23.0, 23.0, 25.0, 35.0, 28.0, 37.0, 39.0, 58.0, 97.0, 161.0, 171.0, 208.0, 272.0, 454.0, 780.0, 1240.0, 1656.0, 1828.0, 2201.0, 2148.0, 2455.0, 2322.0, 2176.0, 2107.0, 2240.0, 2361.0, 1935.0, 2090.0, 1954.0, 2157.0, 2369.0, 2075.0, 2121.0, 2113.0, 2082.0, 1645.0, 1283.0, 957.0, 697.0, 341.0, 148.0, 146.0, 159.0, 125.0, 119.0, 76.0, 35.0, 39.0, 24.0, 22.0, 29.0, 18.0, 25.0, 26.0, 31.0], [26.0, 25.0, 24.0, 31.0, 17.0, 32.0, 31.0, 30.0, 42.0, 43.0, 40.0, 112.0, 160.0, 197.0, 206.0, 412.0, 591.0, 1027.0, 1297.0, 2009.0, 1983.0, 2195.0, 2421.0, 2361.0, 2193.0, 2123.0, 2032.0, 1962.0, 1456.0, 2074.0, 1780.0, 2208.0, 2033.0, 2126.0, 2187.0, 2256.0, 2024.0, 2050.0, 1916.0, 1412.0, 1075.0, 640.0, 396.0, 242.0, 147.0, 138.0, 105.0, 119.0, 88.0, 62.0, 24.0, 35.0, 26.0, 23.0, 26.0, 25.0, 22.0, 26.0], [28.0, 22.0, 21.0, 26.0, 37.0, 22.0, 22.0, 30.0, 39.0, 37.0, 48.0, 139.0, 172.0, 173.0, 200.0, 392.0, 564.0, 1048.0, 1302.0, 1840.0, 2436.0, 2364.0, 2111.0, 2291.0, 1957.0, 2085.0, 1930.0, 2025.0, 2097.0, 1703.0, 2050.0, 1845.0, 1843.0, 2229.0, 2178.0, 2014.0, 2190.0, 2263.0, 1880.0, 1400.0, 1075.0, 803.0, 439.0, 253.0, 140.0, 135.0, 142.0, 127.0, 78.0, 45.0, 35.0, 35.0, 27.0, 26.0, 40.0, 28.0, 30.0, 37.0], [28.0, 15.0, 40.0, 23.0, 22.0, 30.0, 35.0, 41.0, 39.0, 31.0, 57.0, 151.0, 201.0, 193.0, 237.0, 428.0, 717.0, 1152.0, 1466.0, 1986.0, 1995.0, 2446.0, 2190.0, 2780.0, 1891.0, 2293.0, 1842.0, 2093.0, 1750.0, 1949.0, 1578.0, 1870.0, 2034.0, 2128.0, 2093.0, 2584.0, 1994.0, 2018.0, 1757.0, 1768.0, 1185.0, 878.0, 462.0, 256.0, 133.0, 127.0, 152.0, 98.0, 76.0, 59.0, 33.0, 30.0, 36.0, 36.0, 21.0, 33.0, 34.0, 35.0], [19.0, 24.0, 27.0, 21.0, 28.0, 18.0, 24.0, 31.0, 50.0, 46.0, 60.0, 152.0, 176.0, 221.0, 198.0, 462.0, 716.0, 1289.0, 1545.0, 2029.0, 1973.0, 2329.0, 2298.0, 2125.0, 1928.0, 2383.0, 1739.0, 2039.0, 1517.0, 1969.0, 1908.0, 2052.0, 1783.0, 2343.0, 1997.0, 2315.0, 2064.0, 2142.0, 1654.0, 1663.0, 1028.0, 917.0, 421.0, 247.0, 149.0, 128.0, 132.0, 115.0, 73.0, 36.0, 31.0, 26.0, 38.0, 24.0, 19.0, 34.0, 18.0, 29.0], [17.0, 23.0, 30.0, 18.0, 21.0, 37.0, 29.0, 19.0, 44.0, 38.0, 56.0, 124.0, 192.0, 209.0, 191.0, 407.0, 680.0, 1055.0, 1445.0, 1786.0, 2029.0, 2329.0, 2152.0, 2575.0, 2349.0, 1769.0, 1978.0, 1832.0, 1777.0, 1954.0, 1685.0, 2051.0, 1603.0, 2476.0, 2126.0, 2405.0, 2335.0, 2159.0, 1893.0, 1784.0, 1227.0, 828.0, 467.0, 280.0, 136.0, 155.0, 132.0, 108.0, 60.0, 64.0, 40.0, 28.0, 35.0, 21.0, 31.0, 30.0, 28.0, 39.0], [28.0, 25.0, 37.0, 24.0, 17.0, 32.0, 23.0, 23.0, 37.0, 34.0, 37.0, 153.0, 163.0, 161.0, 207.0, 341.0, 599.0, 1189.0, 1438.0, 2097.0, 2129.0, 2424.0, 2151.0, 2149.0, 2264.0, 2330.0, 2010.0, 2014.0, 1850.0, 1829.0, 2196.0, 1889.0, 1882.0, 2111.0, 2084.0, 2151.0, 2128.0, 2330.0, 1620.0, 1681.0, 1118.0, 819.0, 461.0, 261.0, 165.0, 141.0, 112.0, 124.0, 79.0, 43.0, 35.0, 29.0, 22.0, 35.0, 23.0, 32.0, 33.0, 19.0], [14.0, 20.0, 20.0, 23.0, 25.0, 38.0, 28.0, 31.0, 34.0, 34.0, 44.0, 121.0, 197.0, 222.0, 204.0, 320.0, 581.0, 1108.0, 1258.0, 1879.0, 2089.0, 2441.0, 1964.0, 2801.0, 1994.0, 2487.0, 1873.0, 2261.0, 1906.0, 1970.0, 1685.0, 2151.0, 2006.0, 2058.0, 2187.0, 2728.0, 2094.0, 2027.0, 2020.0, 1558.0, 1088.0, 625.0, 395.0, 260.0, 126.0, 147.0, 106.0, 95.0, 94.0, 44.0, 38.0, 35.0, 20.0, 18.0, 26.0, 23.0, 17.0, 32.0], [22.0, 26.0, 20.0, 20.0, 18.0, 25.0, 34.0, 26.0, 34.0, 44.0, 46.0, 84.0, 158.0, 164.0, 195.0, 299.0, 430.0, 960.0, 1335.0, 1706.0, 1940.0, 2398.0, 2023.0, 2542.0, 2089.0, 2145.0, 2194.0, 2256.0, 1890.0, 2339.0, 1918.0, 2125.0, 2012.0, 2507.0, 2110.0, 2056.0, 2412.0, 2209.0, 1720.0, 1525.0, 949.0, 620.0, 338.0, 194.0, 96.0, 141.0, 127.0, 77.0, 65.0, 43.0, 38.0, 29.0, 40.0, 36.0, 16.0, 32.0, 22.0, 29.0], [19.0, 23.0, 26.0, 23.0, 19.0, 29.0, 23.0, 33.0, 34.0, 35.0, 43.0, 72.0, 140.0, 214.0, 194.0, 283.0, 507.0, 655.0, 971.0, 1711.0, 1613.0, 2204.0, 2346.0, 2051.0, 2402.0, 2269.0, 2225.0, 2162.0, 2085.0, 2395.0, 1843.0, 2267.0, 2151.0, 2149.0, 2225.0, 2380.0, 1896.0, 1818.0, 1475.0, 1218.0, 750.0, 496.0, 265.0, 205.0, 125.0, 130.0, 115.0, 111.0, 57.0, 25.0, 34.0, 44.0, 37.0, 32.0, 19.0, 31.0, 27.0, 38.0], [27.0, 20.0, 28.0, 19.0, 25.0, 17.0, 21.0, 28.0, 43.0, 51.0, 43.0, 57.0, 98.0, 195.0, 198.0, 267.0, 258.0, 605.0, 863.0, 1362.0, 1715.0, 1926.0, 2086.0, 2439.0, 2163.0, 2529.0, 2245.0, 2240.0, 1911.0, 2777.0, 2329.0, 2224.0, 2050.0, 2287.0, 2157.0, 2352.0, 1831.0, 1977.0, 1315.0, 1129.0, 678.0, 502.0, 201.0, 176.0, 130.0, 137.0, 80.0, 74.0, 45.0, 32.0, 35.0, 27.0, 18.0, 26.0, 32.0, 30.0, 29.0, 28.0], [18.0, 18.0, 21.0, 21.0, 23.0, 23.0, 19.0, 44.0, 37.0, 29.0, 37.0, 37.0, 81.0, 161.0, 187.0, 216.0, 274.0, 516.0, 725.0, 1052.0, 1369.0, 1730.0, 2045.0, 2141.0, 1878.0, 2262.0, 2191.0, 2218.0, 2323.0, 2192.0, 2213.0, 2159.0, 2086.0, 2382.0, 2123.0, 1941.0, 1751.0, 1611.0, 1087.0, 864.0, 544.0, 259.0, 169.0, 136.0, 117.0, 150.0, 107.0, 71.0, 23.0, 29.0, 29.0, 28.0, 21.0, 18.0, 31.0, 30.0, 27.0, 39.0], [22.0, 21.0, 20.0, 19.0, 21.0, 22.0, 19.0, 30.0, 28.0, 30.0, 41.0, 43.0, 56.0, 138.0, 193.0, 209.0, 193.0, 364.0, 496.0, 1100.0, 1038.0, 1573.0, 1646.0, 2038.0, 2123.0, 2156.0, 2117.0, 2271.0, 1960.0, 2545.0, 1993.0, 2435.0, 2202.0, 2111.0, 1786.0, 1906.0, 1332.0, 1463.0, 802.0, 716.0, 387.0, 285.0, 134.0, 167.0, 128.0, 125.0, 88.0, 56.0, 39.0, 32.0, 21.0, 33.0, 25.0, 34.0, 22.0, 22.0, 23.0, 0.0], [21.0, 20.0, 12.0, 29.0, 26.0, 32.0, 13.0, 32.0, 41.0, 17.0, 36.0, 56.0, 35.0, 101.0, 195.0, 150.0, 185.0, 290.0, 363.0, 557.0, 820.0, 1194.0, 1265.0, 1848.0, 1540.0, 2260.0, 2055.0, 2183.0, 2084.0, 2163.0, 2104.0, 2223.0, 1811.0, 1998.0, 1814.0, 1576.0, 1211.0, 1168.0, 730.0, 463.0, 227.0, 208.0, 129.0, 161.0, 147.0, 104.0, 63.0, 28.0, 34.0, 25.0, 23.0, 28.0, 32.0, 24.0, 15.0, 19.0, 11.0, 0.0], [20.0, 21.0, 22.0, 20.0, 20.0, 26.0, 15.0, 25.0, 27.0, 28.0, 30.0, 39.0, 46.0, 78.0, 89.0, 164.0, 163.0, 220.0, 215.0, 433.0, 567.0, 990.0, 1071.0, 1349.0, 1480.0, 1795.0, 1755.0, 1757.0, 1732.0, 1976.0, 1678.0, 1998.0, 1532.0, 1674.0, 1196.0, 1298.0, 865.0, 667.0, 454.0, 318.0, 171.0, 158.0, 116.0, 135.0, 104.0, 115.0, 43.0, 36.0, 24.0, 29.0, 23.0, 29.0, 31.0, 30.0, 29.0, 26.0, 23.0, 0.0], [0.0, 21.0, 24.0, 24.0, 19.0, 19.0, 32.0, 18.0, 29.0, 34.0, 39.0, 31.0, 40.0, 40.0, 79.0, 178.0, 156.0, 192.0, 210.0, 265.0, 340.0, 562.0, 704.0, 1042.0, 1023.0, 1280.0, 1364.0, 1435.0, 1554.0, 1610.0, 1494.0, 1333.0, 1293.0, 1091.0, 913.0, 949.0, 734.0, 464.0, 302.0, 224.0, 145.0, 140.0, 121.0, 114.0, 84.0, 74.0, 33.0, 47.0, 32.0, 33.0, 28.0, 23.0, 28.0, 20.0, 19.0, 19.0, 0.0, 0.0], [0.0, 20.0, 22.0, 25.0, 23.0, 24.0, 28.0, 18.0, 26.0, 39.0, 30.0, 25.0, 28.0, 32.0, 51.0, 82.0, 142.0, 205.0, 164.0, 186.0, 268.0, 342.0, 404.0, 645.0, 650.0, 919.0, 890.0, 1175.0, 1072.0, 1091.0, 1248.0, 1075.0, 868.0, 1001.0, 715.0, 500.0, 332.0, 260.0, 184.0, 148.0, 125.0, 143.0, 131.0, 113.0, 62.0, 41.0, 25.0, 25.0, 20.0, 40.0, 24.0, 16.0, 22.0, 13.0, 17.0, 21.0, 0.0, 0.0], [0.0, 17.0, 28.0, 24.0, 21.0, 25.0, 16.0, 32.0, 21.0, 26.0, 31.0, 30.0, 49.0, 34.0, 49.0, 50.0, 91.0, 126.0, 166.0, 174.0, 187.0, 215.0, 233.0, 359.0, 444.0, 629.0, 601.0, 771.0, 711.0, 748.0, 630.0, 619.0, 513.0, 612.0, 358.0, 352.0, 242.0, 189.0, 137.0, 161.0, 117.0, 132.0, 112.0, 82.0, 45.0, 40.0, 35.0, 32.0, 23.0, 26.0, 22.0, 31.0, 11.0, 23.0, 23.0, 17.0, 0.0, 0.0], [0.0, 0.0, 16.0, 16.0, 25.0, 33.0, 30.0, 22.0, 24.0, 31.0, 30.0, 32.0, 30.0, 31.0, 44.0, 39.0, 46.0, 98.0, 137.0, 192.0, 217.0, 169.0, 176.0, 242.0, 247.0, 282.0, 279.0, 397.0, 396.0, 455.0, 409.0, 406.0, 299.0, 281.0, 204.0, 167.0, 168.0, 140.0, 169.0, 153.0, 120.0, 132.0, 69.0, 41.0, 24.0, 37.0, 26.0, 30.0, 16.0, 23.0, 19.0, 23.0, 19.0, 24.0, 18.0, 0.0, 0.0, 0.0], [0.0, 0.0, 0.0, 24.0, 32.0, 22.0, 20.0, 30.0, 25.0, 28.0, 18.0, 32.0, 28.0, 26.0, 31.0, 29.0, 38.0, 46.0, 84.0, 161.0, 165.0, 197.0, 166.0, 146.0, 213.0, 216.0, 236.0, 225.0, 204.0, 252.0, 211.0, 271.0, 194.0, 180.0, 149.0, 182.0, 150.0, 152.0, 127.0, 143.0, 100.0, 70.0, 49.0, 26.0, 26.0, 18.0, 19.0, 33.0, 24.0, 23.0, 9.0, 33.0, 18.0, 17.0, 0.0, 0.0, 0.0, 0.0], [0.0, 0.0, 0.0, 23.0, 25.0, 32.0, 22.0, 31.0, 33.0, 41.0, 24.0, 35.0, 20.0, 37.0, 24.0, 33.0, 39.0, 46.0, 52.0, 59.0, 116.0, 158.0, 154.0, 159.0, 167.0, 174.0, 167.0, 168.0, 195.0, 166.0, 158.0, 172.0, 141.0, 182.0, 152.0, 174.0, 138.0, 178.0, 119.0, 111.0, 55.0, 30.0, 30.0, 26.0, 25.0, 25.0, 21.0, 23.0, 29.0, 20.0, 21.0, 20.0, 12.0, 31.0, 0.0, 0.0, 0.0, 0.0], [0.0, 0.0, 0.0, 0.0, 30.0, 26.0, 28.0, 26.0, 32.0, 31.0, 23.0, 26.0, 25.0, 33.0, 30.0, 36.0, 30.0, 34.0, 35.0, 48.0, 44.0, 90.0, 122.0, 166.0, 174.0, 175.0, 142.0, 157.0, 163.0, 188.0, 167.0, 204.0, 191.0, 189.0, 129.0, 169.0, 115.0, 107.0, 85.0, 36.0, 38.0, 30.0, 28.0, 25.0, 12.0, 31.0, 18.0, 26.0, 28.0, 23.0, 24.0, 18.0, 17.0, 0.0, 0.0, 0.0, 0.0, 0.0], [0.0, 0.0, 0.0, 0.0, 0.0, 25.0, 19.0, 23.0, 26.0, 30.0, 21.0, 30.0, 25.0, 24.0, 29.0, 28.0, 27.0, 27.0, 35.0, 34.0, 25.0, 50.0, 52.0, 72.0, 92.0, 112.0, 128.0, 161.0, 144.0, 172.0, 155.0, 126.0, 155.0, 115.0, 106.0, 84.0, 51.0, 50.0, 48.0, 42.0, 22.0, 31.0, 31.0, 22.0, 29.0, 16.0, 23.0, 24.0, 10.0, 28.0, 16.0, 32.0, 0.0, 0.0, 0.0, 0.0, 0.0, 0.0], [0.0, 0.0, 0.0, 0.0, 0.0, 24.0, 26.0, 25.0, 17.0, 28.0, 21.0, 33.0, 30.0, 29.0, 23.0, 30.0, 29.0, 29.0, 42.0, 42.0, 36.0, 29.0, 37.0, 40.0, 55.0, 69.0, 50.0, 77.0, 73.0, 113.0, 85.0, 100.0, 50.0, 67.0, 30.0, 36.0, 44.0, 33.0, 36.0, 29.0, 30.0, 28.0, 27.0, 21.0, 19.0, 29.0, 17.0, 23.0, 24.0, 23.0, 20.0, 30.0, 0.0, 0.0, 0.0, 0.0, 0.0, 0.0], [0.0, 0.0, 0.0, 0.0, 0.0, 0.0, 31.0, 18.0, 29.0, 27.0, 20.0, 30.0, 16.0, 24.0, 31.0, 30.0, 34.0, 41.0, 27.0, 53.0, 36.0, 44.0, 40.0, 37.0, 45.0, 39.0, 39.0, 42.0, 44.0, 43.0, 26.0, 33.0, 36.0, 44.0, 35.0, 41.0, 27.0, 35.0, 33.0, 32.0, 27.0, 26.0, 24.0, 28.0, 16.0, 27.0, 15.0, 23.0, 17.0, 23.0, 14.0, 0.0, 0.0, 0.0, 0.0, 0.0, 0.0, 0.0], [0.0, 0.0, 0.0, 0.0, 0.0, 0.0, 0.0, 25.0, 22.0, 26.0, 25.0, 24.0, 26.0, 29.0, 20.0, 31.0, 34.0, 34.0, 35.0, 38.0, 30.0, 22.0, 34.0, 32.0, 52.0, 28.0, 35.0, 42.0, 35.0, 44.0, 38.0, 67.0, 26.0, 32.0, 20.0, 23.0, 39.0, 29.0, 32.0, 17.0, 20.0, 21.0, 18.0, 25.0, 20.0, 33.0, 19.0, 19.0, 14.0, 20.0, 0.0, 0.0, 0.0, 0.0, 0.0, 0.0, 0.0, 0.0], [0.0, 0.0, 0.0, 0.0, 0.0, 0.0, 0.0, 0.0, 24.0, 20.0, 20.0, 25.0, 24.0, 27.0, 21.0, 30.0, 34.0, 31.0, 28.0, 28.0, 33.0, 36.0, 43.0, 41.0, 29.0, 33.0, 43.0, 29.0, 40.0, 43.0, 52.0, 31.0, 33.0, 36.0, 35.0, 37.0, 30.0, 21.0, 26.0, 29.0, 18.0, 17.0, 37.0, 23.0, 13.0, 21.0, 17.0, 24.0, 21.0, 0.0, 0.0, 0.0, 0.0, 0.0, 0.0, 0.0, 0.0, 0.0], [0.0, 0.0, 0.0, 0.0, 0.0, 0.0, 0.0, 0.0, 0.0, 26.0, 17.0, 18.0, 16.0, 25.0, 42.0, 28.0, 22.0, 37.0, 23.0, 38.0, 26.0, 29.0, 32.0, 33.0, 29.0, 30.0, 25.0, 35.0, 32.0, 34.0, 20.0, 27.0, 25.0, 38.0, 27.0, 28.0, 20.0, 27.0, 27.0, 23.0, 11.0, 20.0, 24.0, 19.0, 22.0, 20.0, 17.0, 15.0, 0.0, 0.0, 0.0, 0.0, 0.0, 0.0, 0.0, 0.0, 0.0, 0.0], [0.0, 0.0, 0.0, 0.0, 0.0, 0.0, 0.0, 0.0, 0.0, 0.0, 0.0, 35.0, 24.0, 16.0, 25.0, 32.0, 20.0, 27.0, 35.0, 18.0, 30.0, 30.0, 24.0, 21.0, 36.0, 36.0, 39.0, 30.0, 30.0, 24.0, 31.0, 19.0, 27.0, 19.0, 37.0, 24.0, 27.0, 21.0, 29.0, 23.0, 22.0, 18.0, 21.0, 17.0, 13.0, 19.0, 0.0, 0.0, 0.0, 0.0, 0.0, 0.0, 0.0, 0.0, 0.0, 0.0, 0.0, 0.0], [0.0, 0.0, 0.0, 0.0, 0.0, 0.0, 0.0, 0.0, 0.0, 0.0, 0.0, 0.0, 22.0, 26.0, 23.0, 29.0, 21.0, 22.0, 30.0, 25.0, 29.0, 27.0, 30.0, 26.0, 26.0, 37.0, 26.0, 30.0, 29.0, 35.0, 27.0, 22.0, 30.0, 35.0, 18.0, 19.0, 23.0, 17.0, 18.0, 23.0, 14.0, 11.0, 20.0, 28.0, 20.0, 0.0, 0.0, 0.0, 0.0, 0.0, 0.0, 0.0, 0.0, 0.0, 0.0, 0.0, 0.0, 0.0], [0.0, 0.0, 0.0, 0.0, 0.0, 0.0, 0.0, 0.0, 0.0, 0.0, 0.0, 0.0, 0.0, 0.0, 31.0, 22.0, 26.0, 17.0, 25.0, 37.0, 27.0, 28.0, 36.0, 27.0, 18.0, 22.0, 34.0, 32.0, 19.0, 27.0, 19.0, 33.0, 28.0, 23.0, 31.0, 14.0, 26.0, 30.0, 21.0, 18.0, 15.0, 18.0, 18.0, 0.0, 0.0, 0.0, 0.0, 0.0, 0.0, 0.0, 0.0, 0.0, 0.0, 0.0, 0.0, 0.0, 0.0, 0.0], [0.0, 0.0, 0.0, 0.0, 0.0, 0.0, 0.0, 0.0, 0.0, 0.0, 0.0, 0.0, 0.0, 0.0, 0.0, 20.0, 29.0, 31.0, 22.0, 25.0, 22.0, 22.0, 18.0, 16.0, 27.0, 32.0, 33.0, 21.0, 29.0, 22.0, 25.0, 29.0, 24.0, 30.0, 22.0, 29.0, 19.0, 22.0, 26.0, 18.0, 24.0, 23.0, 0.0, 0.0, 0.0, 0.0, 0.0, 0.0, 0.0, 0.0, 0.0, 0.0, 0.0, 0.0, 0.0, 0.0, 0.0, 0.0], [0.0, 0.0, 0.0, 0.0, 0.0, 0.0, 0.0, 0.0, 0.0, 0.0, 0.0, 0.0, 0.0, 0.0, 0.0, 0.0, 0.0, 0.0, 28.0, 25.0, 25.0, 21.0, 23.0, 21.0, 23.0, 23.0, 23.0, 29.0, 31.0, 35.0, 20.0, 33.0, 20.0, 22.0, 23.0, 15.0, 14.0, 22.0, 22.0, 0.0, 0.0, 0.0, 0.0, 0.0, 0.0, 0.0, 0.0, 0.0, 0.0, 0.0, 0.0, 0.0, 0.0, 0.0, 0.0, 0.0, 0.0, 0.0], [0.0, 0.0, 0.0, 0.0, 0.0, 0.0, 0.0, 0.0, 0.0, 0.0, 0.0, 0.0, 0.0, 0.0, 0.0, 0.0, 0.0, 0.0, 0.0, 0.0, 0.0, 31.0, 23.0, 24.0, 18.0, 24.0, 23.0, 30.0, 31.0, 17.0, 41.0, 30.0, 28.0, 25.0, 20.0, 17.0, 0.0, 0.0, 0.0, 0.0, 0.0, 0.0, 0.0, 0.0, 0.0, 0.0, 0.0, 0.0, 0.0, 0.0, 0.0, 0.0, 0.0, 0.0, 0.0, 0.0, 0.0, 0.0]]
  out "Signal Bck":dbl[][](graph)
  out "Coincidence image":dbl[][](graph)
  out "Coincidence image Bck":dbl[][](graph)
  in  "Background files":path caption="start path"
  out "zero array":dbl[][](array[numeric])
  in  "Coincidence files":path caption="start path"
  out "Background pix ref crop":T2
  out "Signal Idler pix ref crop":T2
  in  "Centroid shift bound (pixels)":dbl=30.0 format="%#_13g"
  in  "Beam Diameter (mm)\n4 sigma":dbl=0.217
  in  "Load New Reference?":bool=TRUE
  out "Beam size ref":T5={"Signal x size"=160.0, "Signal y size"=160.0, "Idler x size"=2.0, "Idler y size"=2.0}
  out "Background pix ref":T2
  out "Signal Idler pix ref":T2
  in  "focal length (m)":dbl=0.25 format="%#_13g"
  out "Background pix":T2
  out "Beam size (pixels)":T5={"Signal x size"=160.0, "Signal y size"=160.0, "Idler x size"=2.0, "Idler y size"=2.0}
  out "Signal Idler pix":T2
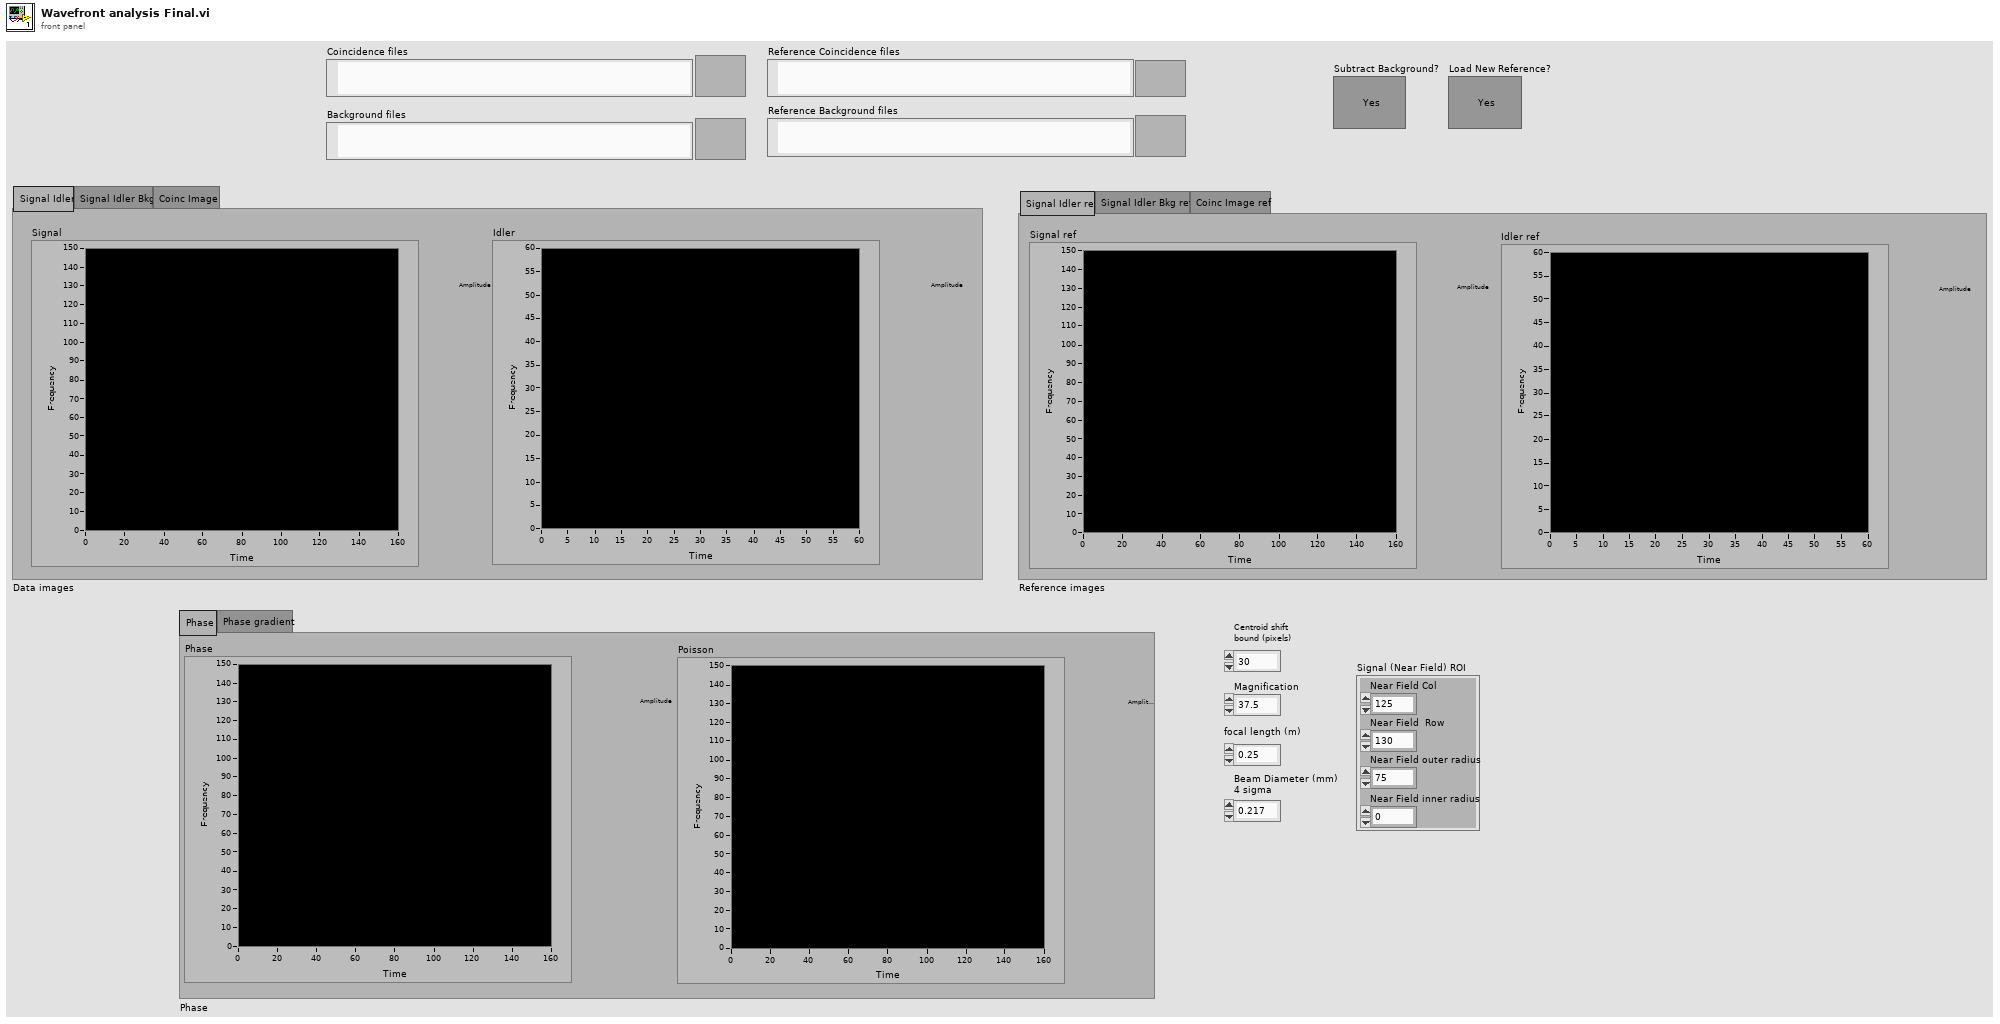
[diagram p1: front panel]
types:
  T1 = enum32{"Signal Idler ref", "Signal Idler Bkg ref", "Coinc Image ref"}
  T2 = cluster{"Signal x":dbl[], "Signal y":dbl[], "Idler x":dbl[], "Idler y":dbl[]}
  T3 = cluster{"Near Field  Row":i32, "Near Field Col":i32, "Near Field outer radius":i32, "Near Field inner radius":i32}
  T4 = enum32{"Signal Idler", "Signal Idler Bkg", "Coinc Image"}
  T5 = cluster{"Signal x size":dbl, "Signal y size":dbl, "Idler x size":dbl, "Idler y size":dbl}
  T6 = enum16{"fire", "rainbow", "gray", "inverse gray", "ice", "original"}
  T7 = cluster{"Far Field Row":dbl[], "Far Field Col":dbl[]}
  T8 = cluster{"Near Field Row":dbl[], "Near Field Col":dbl[]}
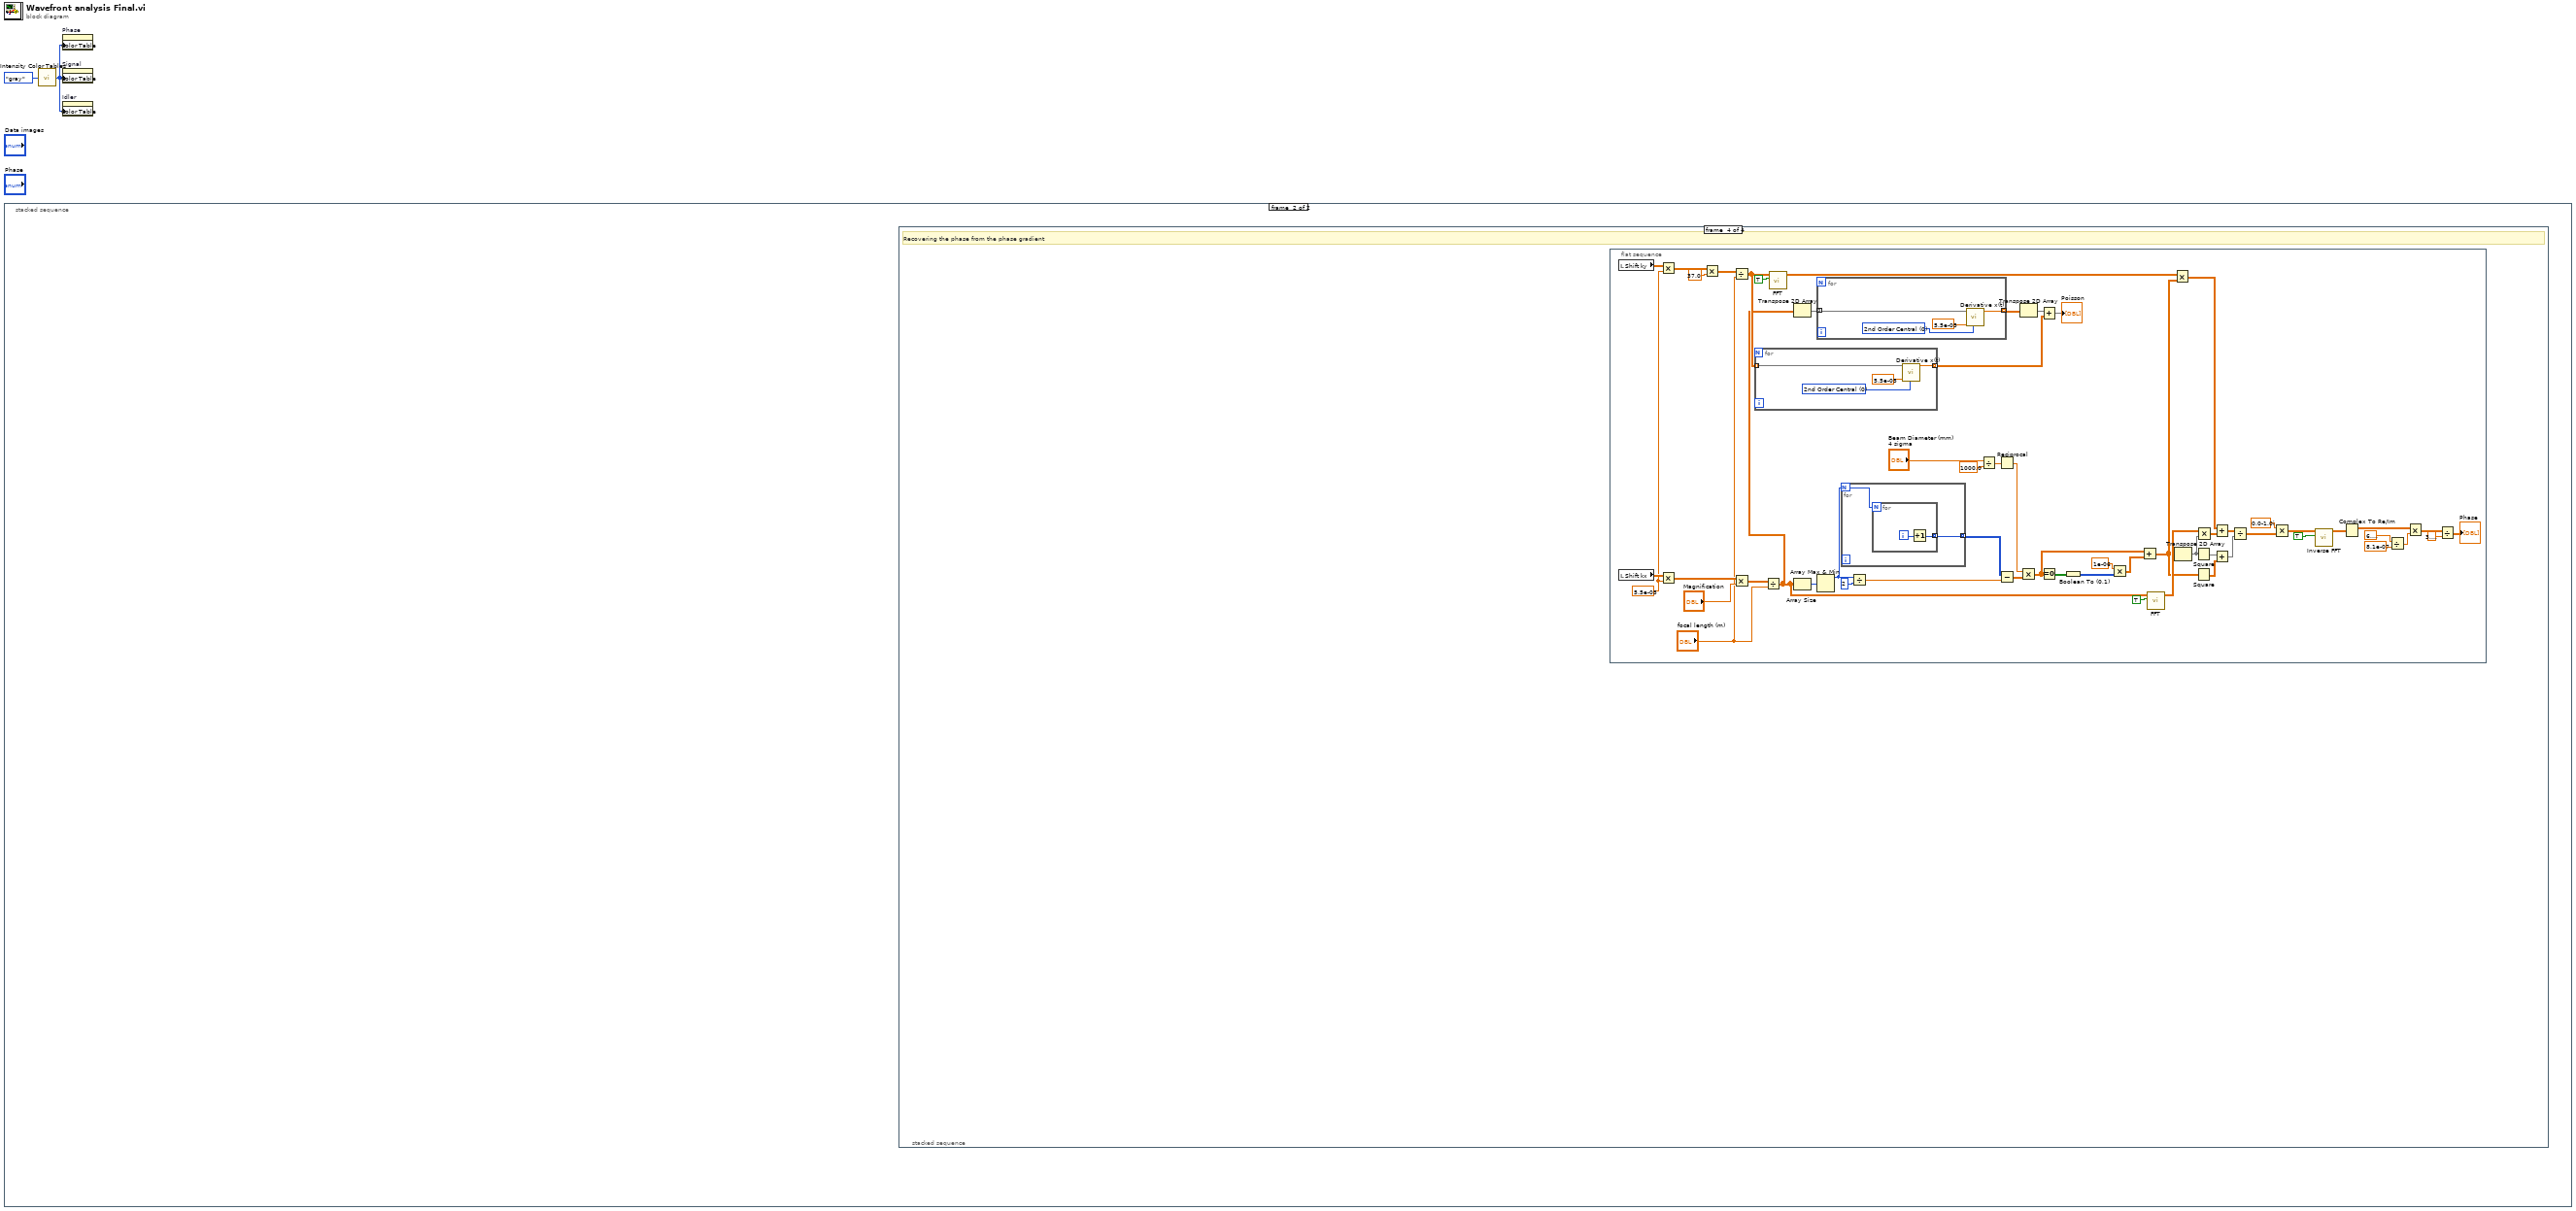
[diagram p0: block diagram]
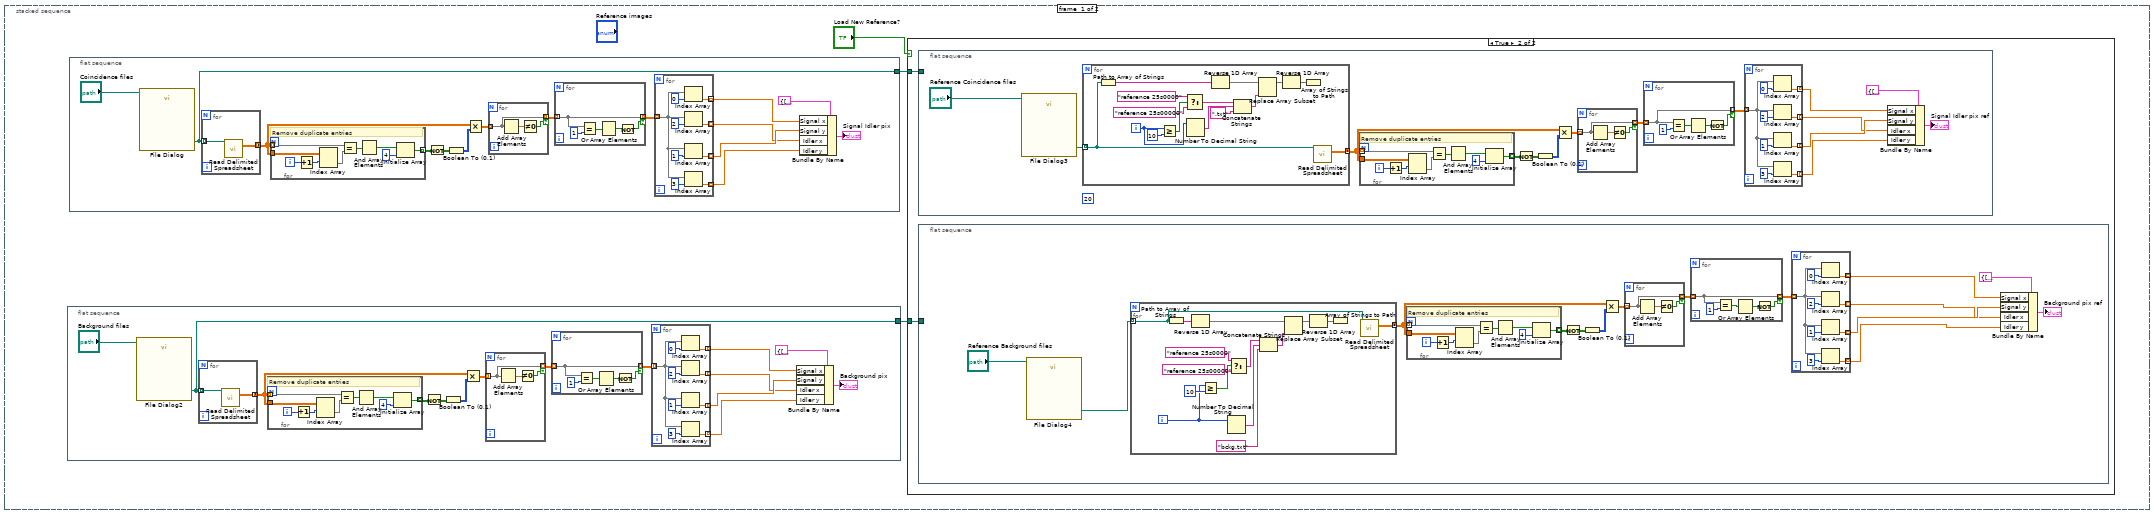
[diagram p2: hidden frame]
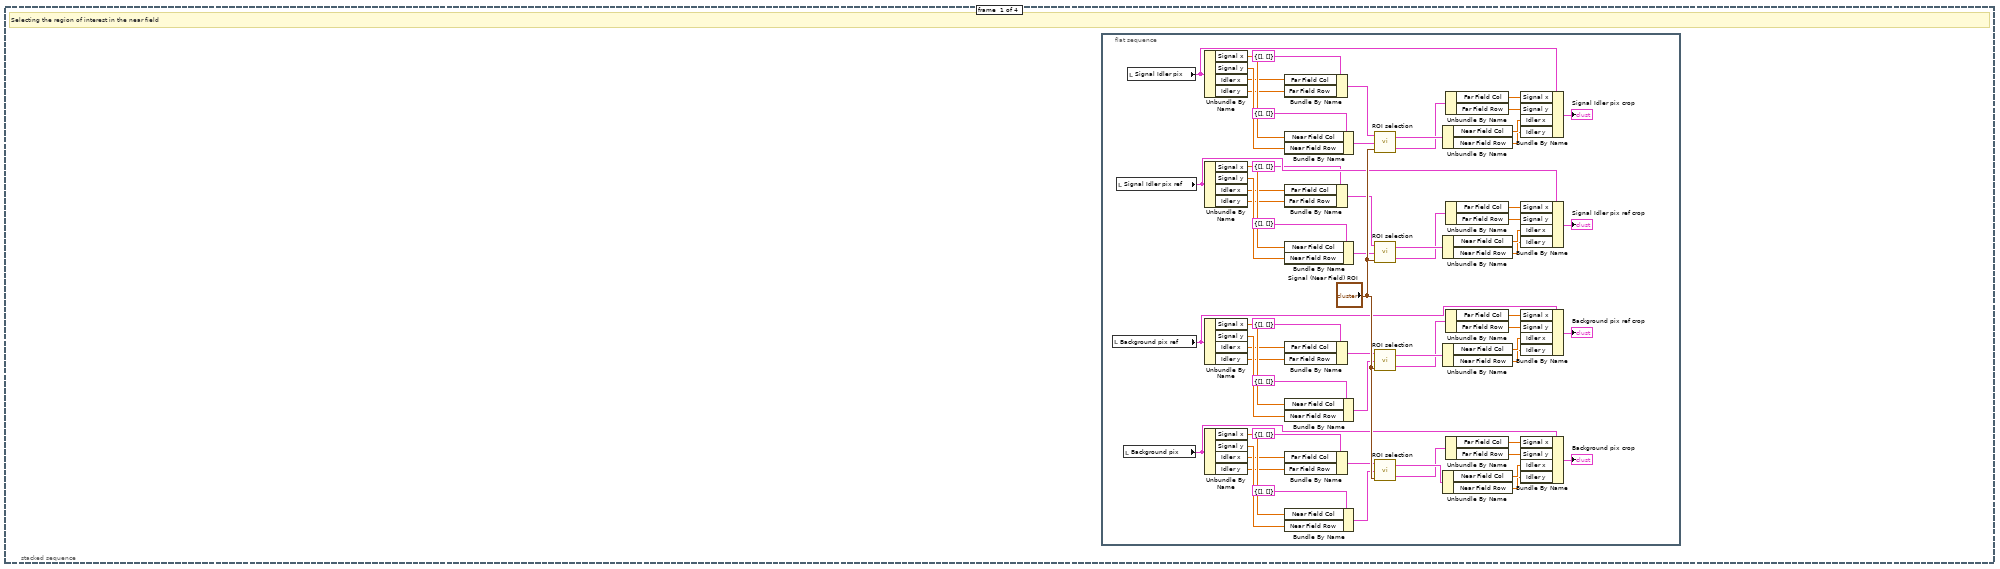
[diagram p4: hidden frame]
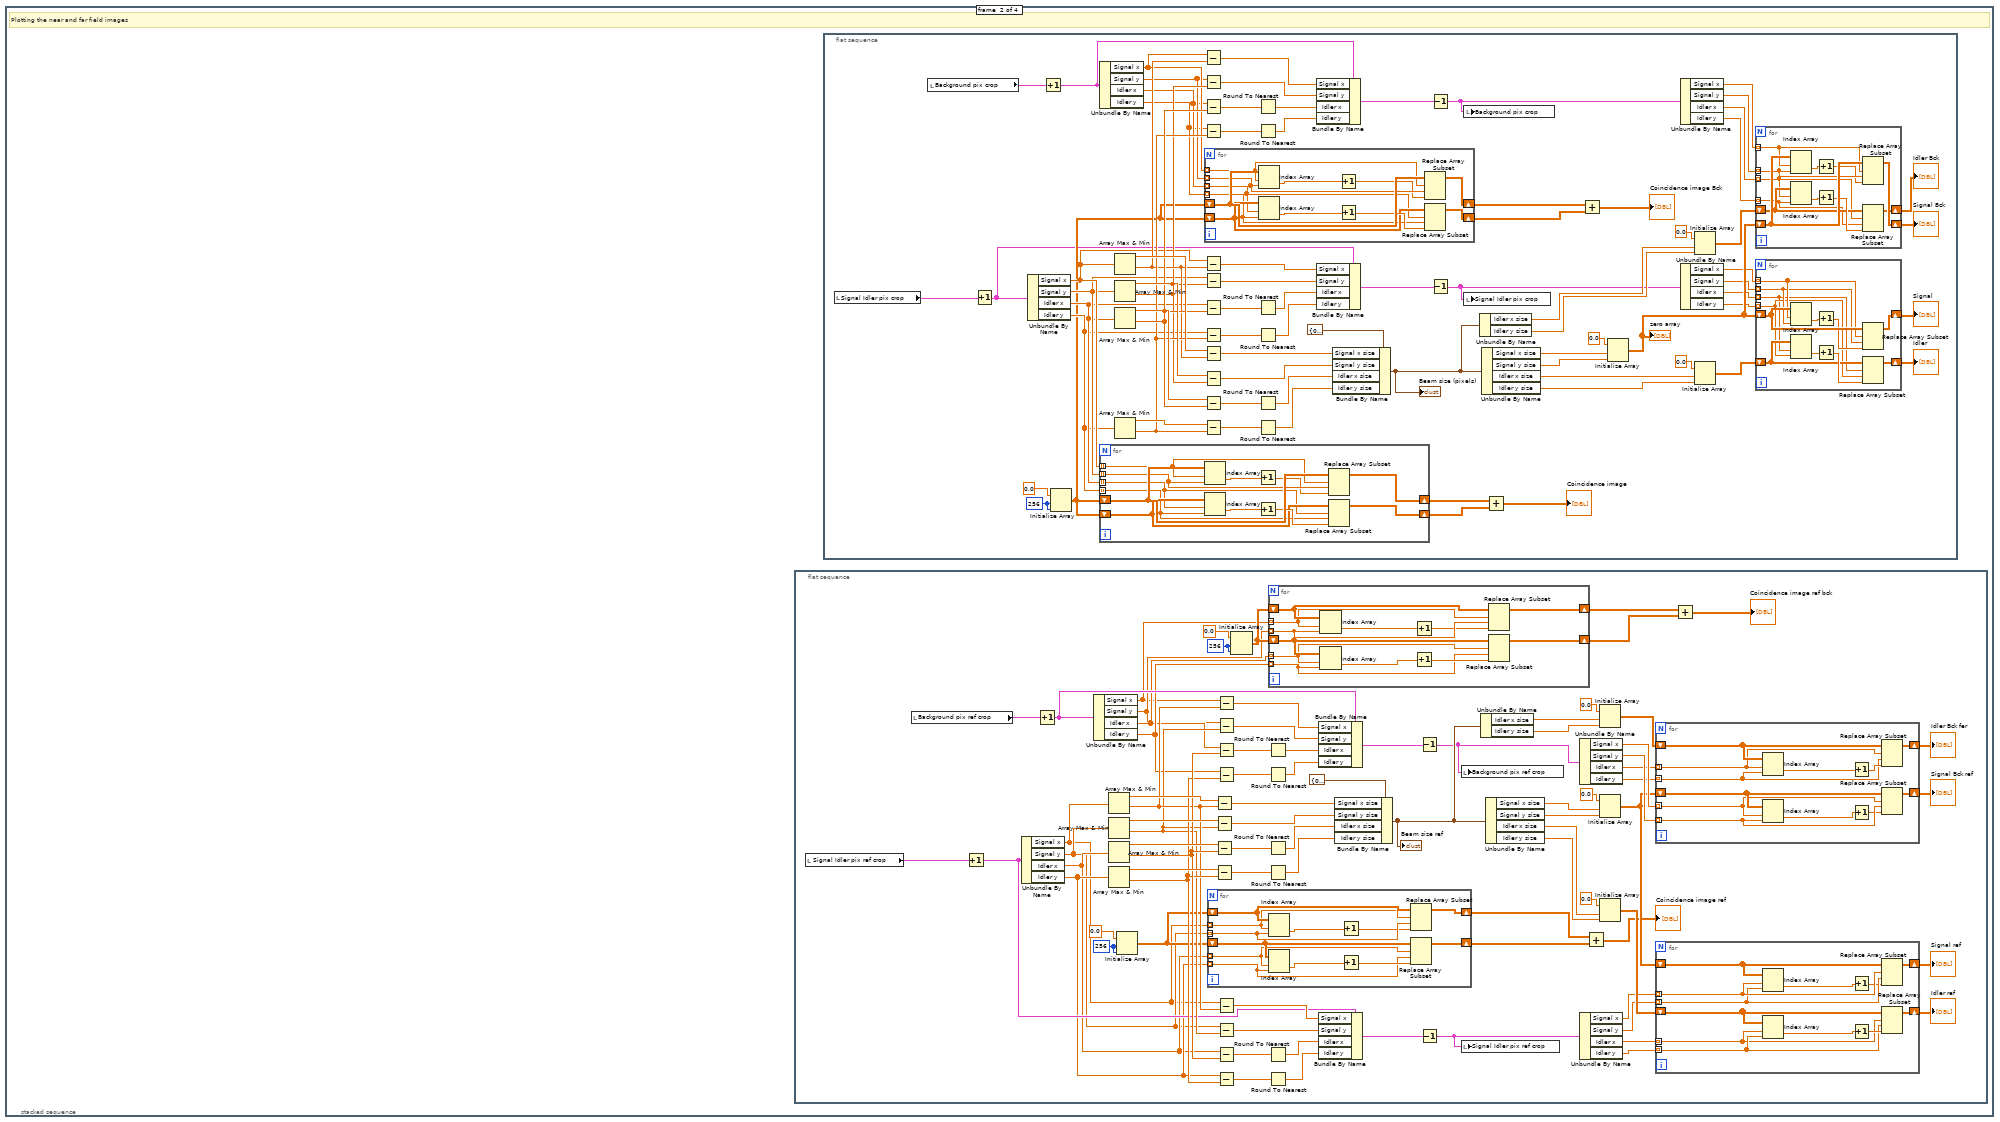
[diagram p5: hidden frame]
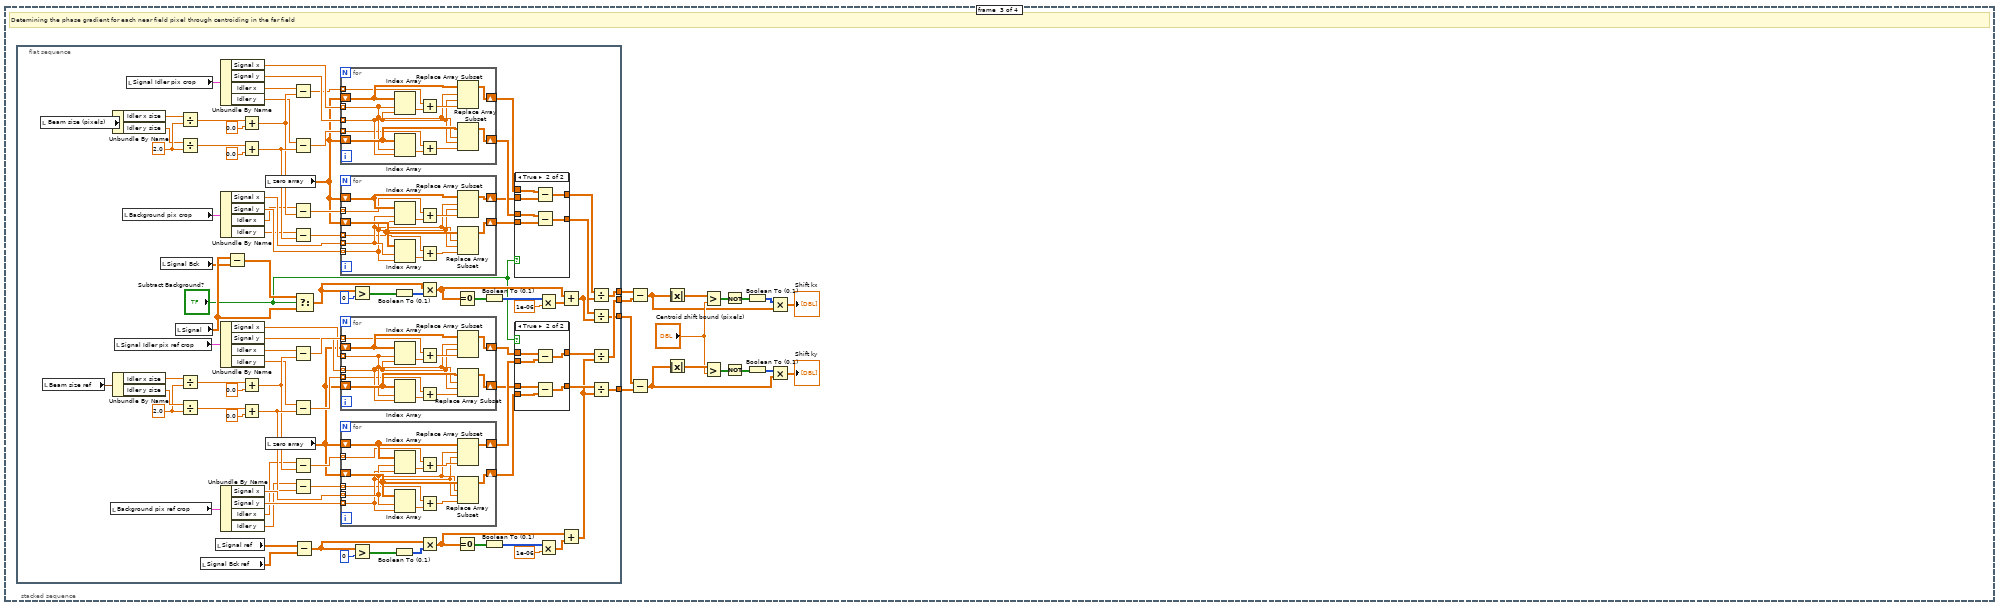
[diagram p6: hidden frame]
diagram:
  n1 = stacked-sequence {
    frame #0 {
      # "Load Coincidence and Background Coincidence"
      n2 = flat-sequence {
        tunnel: [w12] -> w4
        frame #0 {
          n3 = call "File Dialog2"("start path"="Background files") -> ("selected paths"=w12:path[])  [unwired: 11 in, 3 out]
          n4 = for {
            tunnel: w12 -> [w48] mode=indexing
            tunnel: [w47] -> w11 mode=concatenating
            n5 = call-poly <vilib>:"Read Delimited Spreadsheet.vi"("file path (dialog if empty)"=w48) -> ("all rows"=w47:dbl[][])  [unwired: 9 in, 5 out]
          }
          n6 = for {
            tunnel: w11 -> [w42] mode=indexing
            tunnel: w11 -> [w46]
            tunnel: [w38] -> w19 mode=indexing
            i -> [w45]
            # "Remove duplicate entries"
            n7 = Increment(x=w45) -> (x+1=w44:i32)
            n8 = Index Array(array=w46, index (row)=w44) -> (element=w43:dbl[])  [unwired: 1 in]
            n9 = Equal?(x=w42, y=w43) -> (x = y?=w41:bool[])
            n10 = And Array Elements(Boolean array=w41) -> (logical AND=w40:bool)
            n11 = Initialize Array(w40, 4 ("dimension size")) -> (w38:bool[])
          }
          n12 = Not(x=w19) -> (.not. x?=w18:bool[][])
          n13 = Boolean To (0,1)(Boolean=w18) -> (0, 1=w17:i16[][])
          n14 = Multiply(x=w11, y=w17) -> (x*y=w10:dbl[][])
          n15 = for {
            tunnel: w10 -> [w35] mode=indexing
            tunnel: [w35] -> w8 mode=indexing if=w36
            n16 = Add Array Elements(numeric array=w35) -> (sum=w37:dbl)
            n17 = Not Equal To 0?(x=w37) -> (x != 0?=w36:bool)
          }
          n18 = for {
            tunnel: w8 -> [w22] mode=indexing
            tunnel: [w22] -> w9 mode=indexing if=w21
            n19 = Equal?(x=w22, y=1) -> (x = y?=w24:bool[])
            n20 = Or Array Elements(Boolean array=w24) -> (logical OR=w23:bool)
            n21 = Not(x=w23) -> (.not. x?=w21:bool)
          }
          n22 = for {
            tunnel: w9 -> [w30] mode=indexing
            tunnel: [w29] -> w14 mode=indexing
            tunnel: [w28] -> w6 mode=indexing
            tunnel: [w27] -> w13 mode=indexing
            tunnel: [w26] -> w7 mode=indexing
            n23 = Index Array(array=w30, index=0) -> (element=w29:dbl)
            n24 = Index Array(array=w30, index=2) -> (element=w28:dbl)
            n25 = Index Array(array=w30, index=1) -> (element=w27:dbl)
            n26 = Index Array(array=w30, index=3) -> (element=w26:dbl)
          }
          n27 = Bundle By Name(cluster=T2 {"Signal x"=[], "Signal y"=[], "Idler x"=[], "Idler y"=[]} ("Signal Idler"), "Signal x"=w14, "Signal y"=w13, "Idler x"=w6, "Idler y"=w7) -> (→"Background pix":T2)
        }
      }
      n28 = flat-sequence {
        tunnel: [w57] -> w5
        frame #0 {
          n29 = call "File Dialog"("start path"="Coincidence files") -> ("selected paths"=w57:path[])  [unwired: 11 in, 3 out]
          n30 = for {
            tunnel: w57 -> [w91] mode=indexing
            tunnel: [w90] -> w56 mode=concatenating
            n31 = call-poly <vilib>:"Read Delimited Spreadsheet.vi"("file path (dialog if empty)"=w91) -> ("all rows"=w90:dbl[][])  [unwired: 9 in, 5 out]
          }
          n32 = for {
            tunnel: w56 -> [w85] mode=indexing
            tunnel: w56 -> [w89]
            tunnel: [w81] -> w62 mode=indexing
            i -> [w88]
            # "Remove duplicate entries"
            n33 = Increment(x=w88) -> (x+1=w87:i32)
            n34 = Index Array(array=w89, index (row)=w87) -> (element=w86:dbl[])  [unwired: 1 in]
            n35 = Equal?(x=w85, y=w86) -> (x = y?=w84:bool[])
            n36 = And Array Elements(Boolean array=w84) -> (logical AND=w83:bool)
            n37 = Initialize Array(w83, 4 ("dimension size")) -> (w81:bool[])
          }
          n38 = Not(x=w62) -> (.not. x?=w61:bool[][])
          n39 = Boolean To (0,1)(Boolean=w61) -> (0, 1=w60:i16[][])
          n40 = Multiply(x=w56, y=w60) -> (x*y=w55:dbl[][])
          n41 = for {
            tunnel: w55 -> [w79] mode=indexing
            tunnel: [w79] -> w53 mode=indexing if=w78
            n42 = Add Array Elements(numeric array=w79) -> (sum=w80:dbl)
            n43 = Not Equal To 0?(x=w80) -> (x != 0?=w78:bool)
          }
          n44 = for {
            tunnel: w53 -> [w65] mode=indexing
            tunnel: [w65] -> w52 mode=indexing if=w64
            n45 = Equal?(x=w65, y=1) -> (x = y?=w67:bool[])
            n46 = Or Array Elements(Boolean array=w67) -> (logical OR=w66:bool)
            n47 = Not(x=w66) -> (.not. x?=w64:bool)
          }
          n48 = for {
            tunnel: w52 -> [w73] mode=indexing
            tunnel: [w70] -> w54 mode=indexing
            tunnel: [w72] -> w50 mode=indexing
            tunnel: [w69] -> w58 mode=indexing
            tunnel: [w71] -> w49 mode=indexing
            n49 = Index Array(array=w73, index=0) -> (element=w70:dbl)
            n50 = Index Array(array=w73, index=2) -> (element=w72:dbl)
            n51 = Index Array(array=w73, index=1) -> (element=w69:dbl)
            n52 = Index Array(array=w73, index=3) -> (element=w71:dbl)
          }
          n53 = Bundle By Name(cluster=T2 {"Signal x"=[], "Signal y"=[], "Idler x"=[], "Idler y"=[]} ("Signal Idler"), "Signal x"=w54, "Signal y"=w58, "Idler x"=w50, "Idler y"=w49) -> (→"Signal Idler pix":T2)
        }
      }
      n54 = case shown="True" "Load New Reference?" {
        tunnel: w5 -> [_ w93]
        tunnel: w4 -> [_ w92]
        frame False {
        }
        frame True {
          n55 = flat-sequence {
            tunnel: w93 -> [_]
            frame #0 {
              (unwired) 20
              n56 = call "File Dialog3"("start path"="Reference Coincidence files") -> ("selected paths"=w150:path[])  [unwired: 11 in, 3 out]
              n57 = for {
                tunnel: w150 -> [w191] mode=indexing
                tunnel: [w205] -> w156 mode=concatenating
                i -> [w197]
                n58 = Path to Array of Strings(0:w191) -> (2:w204:string[])  [unwired: 1 out]
                n59 = Greater Or Equal?(x=w197, y=10) -> (x >= y?=w195:bool)
                n60 = Select(t="reference 25s0000" ("string"), s=w195, f="reference 25s00000" ("string")) -> (s? t:f=w192:string)
                n61 = Number To Decimal String(number=w197) -> (decimal integer string=w200:string)  [unwired: 1 in]
                n62 = Reverse 1D Array(array=w204) -> (reversed array=w203:string[])
                n63 = Concatenate Strings(w192, w200, ".txt" ("string")) -> (w202:string)
                n64 = Replace Array Subset(array=w203, new element=w202) -> (w199:string[])  [unwired: 1 in]
                n65 = Reverse 1D Array(array=w199) -> (reversed array=w198:string[])
                n66 = Array of Strings to Path(0:w198) -> ()  [unwired: 1 in, 1 out]
                n67 = call-poly <vilib>:"Read Delimited Spreadsheet.vi"("file path (dialog if empty)"=w191) -> ("all rows"=w205:dbl[][])  [unwired: 9 in, 5 out]
              }
              n68 = for {
                tunnel: w156 -> [w186] mode=indexing
                tunnel: w156 -> [w190]
                tunnel: [w182] -> w164 mode=indexing
                i -> [w189]
                # "Remove duplicate entries"
                n69 = Increment(x=w189) -> (x+1=w188:i32)
                n70 = Index Array(array=w190, index (row)=w188) -> (element=w187:dbl[])  [unwired: 1 in]
                n71 = Equal?(x=w186, y=w187) -> (x = y?=w185:bool[])
                n72 = And Array Elements(Boolean array=w185) -> (logical AND=w184:bool)
                n73 = Initialize Array(w184, 4 ("dimension size")) -> (w182:bool[])
              }
              n74 = Not(x=w164) -> (.not. x?=w163:bool[][])
              n75 = Boolean To (0,1)(Boolean=w163) -> (0, 1=w162:i16[][])
              n76 = Multiply(x=w156, y=w162) -> (x*y=w161:dbl[][])
              n77 = for {
                tunnel: w161 -> [w180] mode=indexing
                tunnel: [w180] -> w155 mode=indexing if=w179
                n78 = Add Array Elements(numeric array=w180) -> (sum=w181:dbl)
                n79 = Not Equal To 0?(x=w181) -> (x != 0?=w179:bool)
              }
              n80 = for {
                tunnel: w155 -> [w166] mode=indexing
                tunnel: [w166] -> w154 mode=indexing if=w165
                n81 = Equal?(x=w166, y=1) -> (x = y?=w168:bool[])
                n82 = Or Array Elements(Boolean array=w168) -> (logical OR=w167:bool)
                n83 = Not(x=w167) -> (.not. x?=w165:bool)
              }
              n84 = for {
                tunnel: w154 -> [w174] mode=indexing
                tunnel: [w173] -> w158 mode=indexing
                tunnel: [w172] -> w152 mode=indexing
                tunnel: [w171] -> w157 mode=indexing
                tunnel: [w170] -> w153 mode=indexing
                n85 = Index Array(array=w174, index=0) -> (element=w173:dbl)
                n86 = Index Array(array=w174, index=2) -> (element=w172:dbl)
                n87 = Index Array(array=w174, index=1) -> (element=w171:dbl)
                n88 = Index Array(array=w174, index=3) -> (element=w170:dbl)
              }
              n89 = Bundle By Name(cluster=T2 {"Signal x"=[], "Signal y"=[], "Idler x"=[], "Idler y"=[]} ("Signal Idler"), "Signal x"=w158, "Signal y"=w157, "Idler x"=w152, "Idler y"=w153) -> (→"Signal Idler pix ref":T2)
            }
          }
          n90 = flat-sequence {
            tunnel: w92 -> [_]
            frame #0 {
              n91 = call "File Dialog4"("start path"="Reference Background files") -> ("selected paths"=w94:path[])  [unwired: 11 in, 3 out]
              n92 = for {
                tunnel: w94 -> [w135] mode=indexing
                tunnel: [w149] -> w100 mode=concatenating
                i -> [w137]
                n93 = Path to Array of Strings(0:w135) -> (2:w148:string[])  [unwired: 1 out]
                n94 = Reverse 1D Array(array=w148) -> (reversed array=w147:string[])
                n95 = Greater Or Equal?(x=w137, y=10) -> (x >= y?=w140:bool)
                n96 = Number To Decimal String(number=w137) -> (decimal integer string=w144:string)  [unwired: 1 in]
                n97 = Select(t="reference 25s0000" ("string"), s=w140, f="reference 25s00000" ("string")) -> (s? t:f=w136:string)
                n98 = Concatenate Strings(w136, w144, "bckg.txt" ("string")) -> (w146:string)
                n99 = Replace Array Subset(array=w147, new element=w146) -> (w143:string[])  [unwired: 1 in]
                n100 = Reverse 1D Array(array=w143) -> (reversed array=w142:string[])
                n101 = Array of Strings to Path(0:w142) -> ()  [unwired: 1 in, 1 out]
                n102 = call-poly <vilib>:"Read Delimited Spreadsheet.vi"("file path (dialog if empty)"=w135) -> ("all rows"=w149:dbl[][])  [unwired: 9 in, 5 out]
              }
              n103 = for {
                tunnel: w100 -> [w130] mode=indexing
                tunnel: w100 -> [w134]
                tunnel: [w126] -> w108 mode=indexing
                i -> [w133]
                # "Remove duplicate entries"
                n104 = Increment(x=w133) -> (x+1=w132:i32)
                n105 = Index Array(array=w134, index (row)=w132) -> (element=w131:dbl[])  [unwired: 1 in]
                n106 = Equal?(x=w130, y=w131) -> (x = y?=w129:bool[])
                n107 = And Array Elements(Boolean array=w129) -> (logical AND=w128:bool)
                n108 = Initialize Array(w128, 4 ("dimension size")) -> (w126:bool[])
              }
              n109 = Not(x=w108) -> (.not. x?=w107:bool[][])
              n110 = Boolean To (0,1)(Boolean=w107) -> (0, 1=w106:i16[][])
              n111 = Multiply(x=w100, y=w106) -> (x*y=w105:dbl[][])
              n112 = for {
                tunnel: w105 -> [w124] mode=indexing
                tunnel: [w124] -> w99 mode=indexing if=w123
                n113 = Add Array Elements(numeric array=w124) -> (sum=w125:dbl)
                n114 = Not Equal To 0?(x=w125) -> (x != 0?=w123:bool)
              }
              n115 = for {
                tunnel: w99 -> [w110] mode=indexing
                tunnel: [w110] -> w98 mode=indexing if=w109
                n116 = Equal?(x=w110, y=1) -> (x = y?=w112:bool[])
                n117 = Or Array Elements(Boolean array=w112) -> (logical OR=w111:bool)
                n118 = Not(x=w111) -> (.not. x?=w109:bool)
              }
              n119 = for {
                tunnel: w98 -> [w118] mode=indexing
                tunnel: [w117] -> w102 mode=indexing
                tunnel: [w116] -> w96 mode=indexing
                tunnel: [w115] -> w101 mode=indexing
                tunnel: [w114] -> w97 mode=indexing
                n120 = Index Array(array=w118, index=0) -> (element=w117:dbl)
                n121 = Index Array(array=w118, index=2) -> (element=w116:dbl)
                n122 = Index Array(array=w118, index=1) -> (element=w115:dbl)
                n123 = Index Array(array=w118, index=3) -> (element=w114:dbl)
              }
              n124 = Bundle By Name(cluster=T2 {"Signal x"=[], "Signal y"=[], "Idler x"=[], "Idler y"=[]} ("Signal Idler"), "Signal x"=w102, "Signal y"=w101, "Idler x"=w96, "Idler y"=w97) -> (→"Background pix ref":T2)
            }
          }
        }
      }
    }
    frame #1 {
      # "Plotting Singal and Idler coincidence images"
      n125 = stacked-sequence {
        frame #0 {
          # "Selecting the region of interest in the near field"
          n126 = flat-sequence {
            frame #0 {
              n127 = local read "Background pix ref"() -> (w265:T2)
              n128 = local read "Signal Idler pix ref"() -> (w267:T2)
              n129 = local read "Background pix"() -> (w268:T2)
              n130 = local read "Signal Idler pix"() -> (w269:T2)
              n131 = Unbundle By Name(w269) -> ("Signal x"=w245:dbl[], "Signal y"=w244:dbl[], "Idler x"=w243:dbl[], "Idler y"=w242:dbl[])
              n132 = Unbundle By Name(w267) -> ("Signal x"=w259:dbl[], "Signal y"=w258:dbl[], "Idler x"=w257:dbl[], "Idler y"=w256:dbl[])
              n133 = Unbundle By Name(w265) -> ("Signal x"=w217:dbl[], "Signal y"=w216:dbl[], "Idler x"=w215:dbl[], "Idler y"=w214:dbl[])
              n134 = Unbundle By Name(w268) -> ("Signal x"=w231:dbl[], "Signal y"=w230:dbl[], "Idler x"=w229:dbl[], "Idler y"=w228:dbl[])
              n135 = Bundle By Name(cluster=T7 {"Far Field Row"=[], "Far Field Col"=[]} ("Far Field pixels"), "Far Field Col"=w243, "Far Field Row"=w242) -> (w241:T7)
              n136 = Bundle By Name(cluster=T8 {"Near Field Row"=[], "Near Field Col"=[]} ("Near Field pixels"), "Near Field Col"=w245, "Near Field Row"=w244) -> (w240:T8)
              n137 = Bundle By Name(cluster=T7 {"Far Field Row"=[], "Far Field Col"=[]} ("Far Field pixels"), "Far Field Col"=w257, "Far Field Row"=w256) -> (w255:T7)
              n138 = Bundle By Name(cluster=T8 {"Near Field Row"=[], "Near Field Col"=[]} ("Near Field pixels"), "Near Field Col"=w259, "Near Field Row"=w258) -> (w254:T8)
              n139 = Bundle By Name(cluster=T7 {"Far Field Row"=[], "Far Field Col"=[]} ("Far Field pixels"), "Far Field Col"=w215, "Far Field Row"=w214) -> (w213:T7)
              n140 = Bundle By Name(cluster=T8 {"Near Field Row"=[], "Near Field Col"=[]} ("Near Field pixels"), "Near Field Col"=w217, "Near Field Row"=w216) -> (w212:T8)
              n141 = Bundle By Name(cluster=T7 {"Far Field Row"=[], "Far Field Col"=[]} ("Far Field pixels"), "Far Field Col"=w229, "Far Field Row"=w228) -> (w227:T7)
              n142 = Bundle By Name(cluster=T8 {"Near Field Row"=[], "Near Field Col"=[]} ("Near Field pixels"), "Near Field Col"=w231, "Near Field Row"=w230) -> (w226:T8)
              n143 = call "ROI selection.vi"("ROI"="Signal (Near Field) ROI", "Far Field pixels"=w240, "Near Field pixels"=w241) -> ("Far Field ROI"=w238:T7, "Near Field ROI"=w239:T8)
              n144 = call "ROI selection.vi"("ROI"="Signal (Near Field) ROI", "Far Field pixels"=w254, "Near Field pixels"=w255) -> ("Far Field ROI"=w252:T7, "Near Field ROI"=w253:T8)
              n145 = call "ROI selection.vi"("ROI"="Signal (Near Field) ROI", "Far Field pixels"=w212, "Near Field pixels"=w213) -> ("Far Field ROI"=w210:T7, "Near Field ROI"=w211:T8)
              n146 = call "ROI selection.vi"("ROI"="Signal (Near Field) ROI", "Far Field pixels"=w226, "Near Field pixels"=w227) -> ("Far Field ROI"=w224:T7, "Near Field ROI"=w225:T8)
              n147 = Unbundle By Name(w239) -> ("Near Field Col"=w237:dbl[], "Near Field Row"=w236:dbl[])
              n148 = Unbundle By Name(w253) -> ("Near Field Col"=w251:dbl[], "Near Field Row"=w250:dbl[])
              n149 = Unbundle By Name(w211) -> ("Near Field Col"=w209:dbl[], "Near Field Row"=w208:dbl[])
              n150 = Unbundle By Name(w225) -> ("Near Field Col"=w223:dbl[], "Near Field Row"=w222:dbl[])
              n151 = Unbundle By Name(w238) -> ("Far Field Col"=w235:dbl[], "Far Field Row"=w234:dbl[])
              n152 = Unbundle By Name(w252) -> ("Far Field Col"=w249:dbl[], "Far Field Row"=w248:dbl[])
              n153 = Unbundle By Name(w210) -> ("Far Field Col"=w207:dbl[], "Far Field Row"=w206:dbl[])
              n154 = Unbundle By Name(w224) -> ("Far Field Col"=w221:dbl[], "Far Field Row"=w220:dbl[])
              n155 = Bundle By Name(cluster=w269, "Signal x"=w235, "Signal y"=w234, "Idler x"=w237, "Idler y"=w236) -> (→"Signal Idler pix crop":T2)
              n156 = Bundle By Name(cluster=w267, "Signal x"=w249, "Signal y"=w248, "Idler x"=w251, "Idler y"=w250) -> (→"Signal Idler pix ref crop":T2)
              n157 = Bundle By Name(cluster=w265, "Signal x"=w207, "Signal y"=w206, "Idler x"=w209, "Idler y"=w208) -> (→"Background pix ref crop":T2)
              n158 = Bundle By Name(cluster=w268, "Signal x"=w221, "Signal y"=w220, "Idler x"=w223, "Idler y"=w222) -> (→"Background pix crop":T2)
            }
          }
        }
        frame #1 {
          # "Plotting the near and far field images"
          n159 = flat-sequence {
            frame #0 {
              w285 = 256 ("dimension size")
              w295 = 256 ("dimension size")
              n160 = local read "Signal Idler pix ref crop"() -> (w302:T2)
              n161 = local read "Background pix ref crop"() -> (w304:T2)
              n162 = Increment(x=w302) -> (x+1=w301:T2)
              n163 = Unbundle By Name(w301) -> ("Signal x"=w287:dbl[], "Signal y"=w288:dbl[], "Idler x"=w289:dbl[], "Idler y"=w290:dbl[])
              n164 = Increment(x=w304) -> (x+1=w303:T2)
              n165 = Unbundle By Name(w303) -> ("Signal x"=w277:dbl[], "Signal y"=w278:dbl[], "Idler x"=w279:dbl[], "Idler y"=w280:dbl[])
              n166 = Array Max & Min(array=w287) -> (max value=w349:dbl, min value=w315:dbl)  [unwired: 2 out]
              n167 = Array Max & Min(array=w288) -> (max value=w348:dbl, min value=w314:dbl)  [unwired: 2 out]
              n168 = Array Max & Min(array=w289) -> (max value=w347:dbl, min value=w317:dbl)  [unwired: 2 out]
              n169 = Array Max & Min(array=w290) -> (max value=w346:dbl, min value=w316:dbl)  [unwired: 2 out]
              n170 = Initialize Array(0.0 ("element"), w295, w295) -> (w291:dbl[][])
              n171 = for {
                shift-right: [w363] -> w293
                shift-left: w291 -> [w366]
                shift-right: [w369] -> w294
                shift-left: w291 -> [w374]
                tunnel: w287 -> [w373] mode=indexing
                tunnel: w288 -> [w372] mode=indexing
                tunnel: w289 -> [w364] mode=indexing
                tunnel: w290 -> [w365] mode=indexing
                n172 = Index Array(array=w374, index (row)=w373, index (col)=w372) -> (element=w371:dbl)
                n173 = Index Array(array=w366, index (row)=w364, index (col)=w365) -> (element=w368:dbl)
                n174 = Increment(x=w371) -> (x+1=w370:dbl)
                n175 = Increment(x=w368) -> (x+1=w367:dbl)
                n176 = Replace Array Subset(array=w374, new element=w370, index (row)=w373, index (col)=w372) -> (w369:dbl[][])
                n177 = Replace Array Subset(array=w366, new element=w367, index (row)=w364, index (col)=w365) -> (w363:dbl[][])
              }
              n178 = Subtract(x=w349, y=w315) -> (x-y=w345:dbl)
              n179 = Subtract(x=w348, y=w314) -> (x-y=w344:dbl)
              n180 = Subtract(x=w347, y=w317) -> (x-y=w274:dbl)
              n181 = Subtract(x=w346, y=w316) -> (x-y=w273:dbl)
              n182 = Subtract(x=w277, y=w315) -> (x-y=w318:dbl[])
              n183 = Subtract(x=w278, y=w314) -> (x-y=w319:dbl[])
              n184 = Subtract(x=w279, y=w317) -> (x-y=w276:dbl[])
              n185 = Subtract(x=w280, y=w316) -> (x-y=w275:dbl[])
              n186 = Subtract(x=w287, y=w315) -> (x-y=w330:dbl[])
              n187 = Subtract(x=w288, y=w314) -> (x-y=w331:dbl[])
              n188 = Subtract(x=w289, y=w317) -> (x-y=w272:dbl[])
              n189 = Subtract(x=w290, y=w316) -> (x-y=w271:dbl[])
              n190 = Initialize Array(0.0 ("element"), w285, w285) -> (w281:dbl[][])
              n191 = Round To Nearest(number=w276) -> (nearest integer value=w310:dbl[])
              n192 = Round To Nearest(number=w275) -> (nearest integer value=w309:dbl[])
              n193 = Round To Nearest(number=w274) -> (nearest integer value=w306:dbl)
              n194 = Round To Nearest(number=w273) -> (nearest integer value=w305:dbl)
              n195 = Round To Nearest(number=w272) -> (nearest integer value=w308:dbl[])
              n196 = Round To Nearest(number=w271) -> (nearest integer value=w307:dbl[])
              n197 = for {
                shift-right: [w351] -> w283
                shift-left: w281 -> [w354]
                shift-right: [w357] -> w284
                shift-left: w281 -> [w362]
                tunnel: w277 -> [w361] mode=indexing
                tunnel: w278 -> [w360] mode=indexing
                tunnel: w279 -> [w352] mode=indexing
                tunnel: w280 -> [w353] mode=indexing
                n198 = Index Array(array=w362, index (row)=w361, index (col)=w360) -> (element=w359:dbl)
                n199 = Index Array(array=w354, index (row)=w352, index (col)=w353) -> (element=w356:dbl)
                n200 = Increment(x=w359) -> (x+1=w358:dbl)
                n201 = Increment(x=w356) -> (x+1=w355:dbl)
                n202 = Replace Array Subset(array=w362, new element=w358, index (row)=w361, index (col)=w360) -> (w357:dbl[][])
                n203 = Replace Array Subset(array=w354, new element=w355, index (row)=w352, index (col)=w353) -> (w351:dbl[][])
              }
              n204 = Bundle By Name(cluster=w303, "Signal x"=w318, "Signal y"=w319, "Idler x"=w310, "Idler y"=w309) -> (w300:T2)
              n205 = Bundle By Name(cluster=w301, "Signal x"=w330, "Signal y"=w331, "Idler x"=w308, "Idler y"=w307) -> (w298:T2)
              n206 = Bundle By Name(cluster=T5 {"Signal x size"=0.0, "Signal y size"=0.0, "Idler x size"=0.0, "Idler y size"=0.0} ("Beam size"), "Signal x size"=w345, "Signal y size"=w344, "Idler x size"=w306, "Idler y size"=w305) -> (w350:T5)
              "Beam size ref" <- w350
              n207 = Decrement(x=w300) -> (x-1=w299:T2)
              n208 = Decrement(x=w298) -> (x-1=w297:T2)
              n209 = local write "Background pix ref crop"(w299) -> ()
              n210 = local write "Signal Idler pix ref crop"(w297) -> ()
              n211 = Unbundle By Name(w350) -> ("Idler x size"=w328:dbl, "Idler y size"=w327:dbl)
              n212 = Unbundle By Name(w350) -> ("Signal x size"=w313:dbl, "Signal y size"=w312:dbl, "Idler x size"=w341:dbl, "Idler y size"=w340:dbl)
              n213 = Unbundle By Name(w299) -> ("Signal x"=w325:dbl[], "Signal y"=w324:dbl[], "Idler x"=w323:dbl[], "Idler y"=w322:dbl[])
              n214 = Unbundle By Name(w297) -> ("Signal x"=w338:dbl[], "Signal y"=w337:dbl[], "Idler x"=w336:dbl[], "Idler y"=w335:dbl[])
              n215 = Add(x=w294, y=w293) -> (x+y=→"Coincidence image ref":dbl[][])
              n216 = Initialize Array(0.0 ("element"), w328, w327) -> (w326:dbl[][])
              n217 = Initialize Array(0.0 ("element"), w341, w340) -> (w339:dbl[][])
              n218 = Initialize Array(0.0 ("element"), w313, w312) -> (w311:dbl[][])
              n219 = for {
                shift-right: [w375] -> w320
                shift-left: w326 -> [w378]
                shift-right: [w381] -> w321
                shift-left: w311 -> [w386]
                tunnel: w325 -> [w385] mode=indexing
                tunnel: w324 -> [w384] mode=indexing
                tunnel: w323 -> [w376] mode=indexing
                tunnel: w322 -> [w377] mode=indexing
                n220 = Index Array(array=w378, index (row)=w376, index (col)=w377) -> (element=w380:dbl)
                n221 = Index Array(array=w386, index (row)=w385, index (col)=w384) -> (element=w383:dbl)
                n222 = Increment(x=w380) -> (x+1=w379:dbl)
                n223 = Increment(x=w383) -> (x+1=w382:dbl)
                n224 = Replace Array Subset(array=w378, new element=w379, index (row)=w376, index (col)=w377) -> (w375:dbl[][])
                n225 = Replace Array Subset(array=w386, new element=w382, index (row)=w385, index (col)=w384) -> (w381:dbl[][])
              }
              "Signal Bck ref" <- w321
              "Idler Bck fer" <- w320
              n226 = for {
                shift-right: [w387] -> w333
                shift-left: w339 -> [w390]
                shift-right: [w393] -> w334
                shift-left: w311 -> [w398]
                tunnel: w338 -> [w397] mode=indexing
                tunnel: w337 -> [w396] mode=indexing
                tunnel: w336 -> [w388] mode=indexing
                tunnel: w335 -> [w389] mode=indexing
                n227 = Index Array(array=w398, index (row)=w397, index (col)=w396) -> (element=w395:dbl)
                n228 = Index Array(array=w390, index (row)=w388, index (col)=w389) -> (element=w392:dbl)
                n229 = Increment(x=w395) -> (x+1=w394:dbl)
                n230 = Increment(x=w392) -> (x+1=w391:dbl)
                n231 = Replace Array Subset(array=w398, new element=w394, index (row)=w397, index (col)=w396) -> (w393:dbl[][])
                n232 = Replace Array Subset(array=w390, new element=w391, index (row)=w388, index (col)=w389) -> (w387:dbl[][])
              }
              "Signal ref" <- w334
              "Idler ref" <- w333
              n233 = Add(x=w284, y=w283) -> (x+y=→"Coincidence image ref bck":dbl[][])
            }
          }
          n234 = flat-sequence {
            frame #0 {
              w434 = 256 ("dimension size")
              n235 = local read "Signal Idler pix crop"() -> (w412:T2)
              n236 = local read "Background pix crop"() -> (w410:T2)
              n237 = Increment(x=w412) -> (x+1=w411:T2)
              n238 = Unbundle By Name(w411) -> ("Signal x"=w433:dbl[], "Signal y"=w432:dbl[], "Idler x"=w431:dbl[], "Idler y"=w430:dbl[])
              n239 = Increment(x=w410) -> (x+1=w409:T2)
              n240 = Initialize Array(0.0 ("element"), w434, w434) -> (w426:dbl[][])
              n241 = Unbundle By Name(w409) -> ("Signal x"=w425:dbl[], "Signal y"=w424:dbl[], "Idler x"=w423:dbl[], "Idler y"=w422:dbl[])
              n242 = for {
                shift-right: [w488] -> w428
                shift-left: w426 -> [w491]
                shift-right: [w494] -> w429
                shift-left: w426 -> [w499]
                tunnel: w433 -> [w498] mode=indexing
                tunnel: w432 -> [w497] mode=indexing
                tunnel: w431 -> [w489] mode=indexing
                tunnel: w430 -> [w490] mode=indexing
                n243 = Index Array(array=w499, index (row)=w498, index (col)=w497) -> (element=w496:dbl)
                n244 = Index Array(array=w491, index (row)=w489, index (col)=w490) -> (element=w493:dbl)
                n245 = Increment(x=w496) -> (x+1=w495:dbl)
                n246 = Increment(x=w493) -> (x+1=w492:dbl)
                n247 = Replace Array Subset(array=w499, new element=w495, index (row)=w498, index (col)=w497) -> (w494:dbl[][])
                n248 = Replace Array Subset(array=w491, new element=w492, index (row)=w489, index (col)=w490) -> (w488:dbl[][])
              }
              n249 = Array Max & Min(array=w433) -> (max value=w474:dbl, min value=w448:dbl)  [unwired: 2 out]
              n250 = Array Max & Min(array=w432) -> (max value=w473:dbl, min value=w447:dbl)  [unwired: 2 out]
              n251 = Array Max & Min(array=w431) -> (max value=w472:dbl, min value=w450:dbl)  [unwired: 2 out]
              n252 = Array Max & Min(array=w430) -> (max value=w471:dbl, min value=w449:dbl)  [unwired: 2 out]
              n253 = Subtract(x=w425, y=w448) -> (x-y=w451:dbl[])
              n254 = Subtract(x=w424, y=w447) -> (x-y=w452:dbl[])
              n255 = Subtract(x=w423, y=w450) -> (x-y=w404:dbl[])
              n256 = Subtract(x=w422, y=w449) -> (x-y=w403:dbl[])
              n257 = Subtract(x=w433, y=w448) -> (x-y=w459:dbl[])
              n258 = Subtract(x=w432, y=w447) -> (x-y=w460:dbl[])
              n259 = Subtract(x=w431, y=w450) -> (x-y=w401:dbl[])
              n260 = Subtract(x=w430, y=w449) -> (x-y=w399:dbl[])
              n261 = Subtract(x=w474, y=w448) -> (x-y=w470:dbl)
              n262 = Subtract(x=w473, y=w447) -> (x-y=w469:dbl)
              n263 = Subtract(x=w472, y=w450) -> (x-y=w402:dbl)
              n264 = Subtract(x=w471, y=w449) -> (x-y=w400:dbl)
              n265 = for {
                shift-right: [w476] -> w419
                shift-left: w426 -> [w479]
                shift-right: [w482] -> w420
                shift-left: w426 -> [w487]
                tunnel: w425 -> [w486] mode=indexing
                tunnel: w424 -> [w485] mode=indexing
                tunnel: w423 -> [w477] mode=indexing
                tunnel: w422 -> [w478] mode=indexing
                n266 = Index Array(array=w487, index (row)=w486, index (col)=w485) -> (element=w484:dbl)
                n267 = Index Array(array=w479, index (row)=w477, index (col)=w478) -> (element=w481:dbl)
                n268 = Increment(x=w484) -> (x+1=w483:dbl)
                n269 = Increment(x=w481) -> (x+1=w480:dbl)
                n270 = Replace Array Subset(array=w487, new element=w483, index (row)=w486, index (col)=w485) -> (w482:dbl[][])
                n271 = Replace Array Subset(array=w479, new element=w480, index (row)=w477, index (col)=w478) -> (w476:dbl[][])
              }
              n272 = Round To Nearest(number=w404) -> (nearest integer value=w416:dbl[])
              n273 = Round To Nearest(number=w403) -> (nearest integer value=w415:dbl[])
              n274 = Round To Nearest(number=w401) -> (nearest integer value=w414:dbl[])
              n275 = Round To Nearest(number=w399) -> (nearest integer value=w413:dbl[])
              n276 = Round To Nearest(number=w402) -> (nearest integer value=w417:dbl)
              n277 = Round To Nearest(number=w400) -> (nearest integer value=w418:dbl)
              n278 = Bundle By Name(cluster=w409, "Signal x"=w451, "Signal y"=w452, "Idler x"=w416, "Idler y"=w415) -> (w406:T2)
              n279 = Bundle By Name(cluster=w411, "Signal x"=w459, "Signal y"=w460, "Idler x"=w414, "Idler y"=w413) -> (w408:T2)
              n280 = Bundle By Name(cluster=T5 {"Signal x size"=0.0, "Signal y size"=0.0, "Idler x size"=0.0, "Idler y size"=0.0} ("Beam size"), "Signal x size"=w470, "Signal y size"=w469, "Idler x size"=w417, "Idler y size"=w418) -> (w475:T5)
              "Beam size (pixels)" <- w475
              n281 = Decrement(x=w406) -> (x-1=w405:T2)
              n282 = Decrement(x=w408) -> (x-1=w407:T2)
              n283 = local write "Background pix crop"(w405) -> ()
              n284 = local write "Signal Idler pix crop"(w407) -> ()
              n285 = Unbundle By Name(w475) -> ("Idler x size"=w457:dbl, "Idler y size"=w456:dbl)
              n286 = Unbundle By Name(w475) -> ("Signal x size"=w445:dbl, "Signal y size"=w444:dbl, "Idler x size"=w466:dbl, "Idler y size"=w465:dbl)
              n287 = Add(x=w429, y=w428) -> (x+y=→"Coincidence image":dbl[][])
              n288 = Add(x=w420, y=w419) -> (x+y=→"Coincidence image Bck":dbl[][])
              n289 = Initialize Array(0.0 ("element"), w445, w444) -> (w446:dbl[][])
              "zero array" <- w446
              n290 = Unbundle By Name(w405) -> ("Signal x"=w436:dbl[], "Signal y"=w437:dbl[], "Idler x"=w438:dbl[], "Idler y"=w439:dbl[])
              n291 = Unbundle By Name(w407) -> ("Signal x"=w440:dbl[], "Signal y"=w441:dbl[], "Idler x"=w442:dbl[], "Idler y"=w443:dbl[])
              n292 = Initialize Array(0.0 ("element"), w457, w456) -> (w455:dbl[][])
              n293 = Initialize Array(0.0 ("element"), w466, w465) -> (w464:dbl[][])
              n294 = for {
                shift-right: [w500] -> w453
                shift-left: w455 -> [w503]
                shift-right: [w506] -> w454
                shift-left: w446 -> [w511]
                tunnel: w436 -> [w510] mode=indexing
                tunnel: w437 -> [w509] mode=indexing
                tunnel: w438 -> [w501] mode=indexing
                tunnel: w439 -> [w502] mode=indexing
                n295 = Index Array(array=w511, index (row)=w510, index (col)=w509) -> (element=w508:dbl)
                n296 = Index Array(array=w503, index (row)=w501, index (col)=w502) -> (element=w505:dbl)
                n297 = Increment(x=w508) -> (x+1=w507:dbl)
                n298 = Increment(x=w505) -> (x+1=w504:dbl)
                n299 = Replace Array Subset(array=w511, new element=w507, index (row)=w510, index (col)=w509) -> (w506:dbl[][])
                n300 = Replace Array Subset(array=w503, new element=w504, index (row)=w501, index (col)=w502) -> (w500:dbl[][])
              }
              "Signal Bck" <- w454
              "Idler Bck" <- w453
              n301 = for {
                shift-right: [w512] -> w462
                shift-left: w464 -> [w515]
                shift-right: [w518] -> w463
                shift-left: w446 -> [w523]
                tunnel: w440 -> [w522] mode=indexing
                tunnel: w441 -> [w521] mode=indexing
                tunnel: w442 -> [w513] mode=indexing
                tunnel: w443 -> [w514] mode=indexing
                n302 = Index Array(array=w523, index (row)=w522, index (col)=w521) -> (element=w520:dbl)
                n303 = Index Array(array=w515, index (row)=w513, index (col)=w514) -> (element=w517:dbl)
                n304 = Increment(x=w520) -> (x+1=w519:dbl)
                n305 = Increment(x=w517) -> (x+1=w516:dbl)
                n306 = Replace Array Subset(array=w523, new element=w519, index (row)=w522, index (col)=w521) -> (w518:dbl[][])
                n307 = Replace Array Subset(array=w515, new element=w516, index (row)=w513, index (col)=w514) -> (w512:dbl[][])
              }
              "Signal" <- w463
              "Idler" <- w462
            }
          }
        }
        frame #2 {
          # "Detemining the phase gradient for each near field pixel through centroiding in the far field"
          n308 = flat-sequence {
            tunnel: [w548] -> w529
            tunnel: [w547] -> w528
            tunnel: [w546] -> w527
            tunnel: [w545] -> w526
            frame #0 {
              w592 = 2.0 ("y")
              w631 = 2.0 ("y")
              n309 = local read "Beam size (pixels)"() -> (w632:T5)
              n310 = local read "Beam size ref"() -> (w591:T5)
              n311 = local read "Background pix ref crop"() -> (w593:T2)
              n312 = Unbundle By Name(w632) -> ("Idler x size"=w628:dbl, "Idler y size"=w627:dbl)
              n313 = Unbundle By Name(w591) -> ("Idler x size"=w601:dbl, "Idler y size"=w602:dbl)
              n314 = local read "Signal Idler pix ref crop"() -> (w587:T2)
              n315 = local read "Background pix crop"() -> (w581:T2)
              n316 = local read "Signal Idler pix crop"() -> (w582:T2)
              n317 = local read "Signal Bck"() -> (w555:dbl[][])
              n318 = local read "Signal"() -> (w557:dbl[][])
              n319 = Divide(x=w628, y=w631) -> (x/y=w553:dbl)
              n320 = Divide(x=w627, y=w631) -> (x/y=w552:dbl)
              n321 = Divide(x=w601, y=w592) -> (x/y=w597:dbl)
              n322 = Divide(x=w602, y=w592) -> (x/y=w598:dbl)
              n323 = local read "Signal Bck ref"() -> (w594:dbl[][])
              n324 = local read "Signal ref"() -> (w588:dbl[][])
              n325 = Unbundle By Name(w582) -> ("Signal x"=w622:dbl[], "Signal y"=w621:dbl[], "Idler x"=w570:dbl[], "Idler y"=w569:dbl[])
              n326 = Unbundle By Name(w581) -> ("Signal x"=w616:dbl[], "Signal y"=w615:dbl[], "Idler x"=w568:dbl[], "Idler y"=w567:dbl[])
              n327 = Unbundle By Name(w587) -> ("Signal x"=w607:dbl[], "Signal y"=w608:dbl[], "Idler x"=w566:dbl[], "Idler y"=w565:dbl[])
              n328 = Unbundle By Name(w593) -> ("Signal x"=w613:dbl[], "Signal y"=w614:dbl[], "Idler x"=w564:dbl[], "Idler y"=w563:dbl[])
              n329 = Subtract(x=w557, y=w555) -> (x-y=w559:dbl[][])
              n330 = Add(x=w553, y=0.0) -> (x+y=w579:dbl)
              n331 = Add(x=w552, y=0.0) -> (x+y=w580:dbl)
              n332 = Add(x=w597, y=0.0) -> (x+y=w584:dbl)
              n333 = Add(x=w598, y=0.0) -> (x+y=w585:dbl)
              n334 = local read "zero array"() -> (w583:dbl[][])
              n335 = local read "zero array"() -> (w586:dbl[][])
              n336 = Subtract(x=w570, y=w579) -> (x-y=w620:dbl[])
              n337 = Subtract(x=w569, y=w580) -> (x-y=w619:dbl[])
              n338 = Subtract(x=w568, y=w579) -> (x-y=w618:dbl[])
              n339 = Subtract(x=w567, y=w580) -> (x-y=w617:dbl[])
              n340 = Subtract(x=w566, y=w584) -> (x-y=w609:dbl[])
              n341 = Subtract(x=w565, y=w585) -> (x-y=w610:dbl[])
              n342 = Subtract(x=w564, y=w584) -> (x-y=w611:dbl[])
              n343 = Subtract(x=w563, y=w585) -> (x-y=w612:dbl[])
              n344 = Subtract(x=w588, y=w594) -> (x-y=w572:dbl[][])
              n345 = Select(t=w559, s="Subtract Background?", f=w557) -> (s? t:f=w558:dbl[][])
              n346 = for {
                tunnel: w622 -> [w688] mode=indexing
                tunnel: w621 -> [w687] mode=indexing
                tunnel: w620 -> [w685] mode=indexing
                tunnel: w619 -> [w686] mode=indexing
                shift-right: [w691] -> w561
                shift-left: w583 -> [w696]
                shift-right: [w692] -> w560
                shift-left: w583 -> [w693]
                n347 = Index Array(array=w696, index (row)=w688, index (col)=w687) -> (element=w695:dbl)
                n348 = Index Array(array=w693, index (row)=w688, index (col)=w687) -> (element=w694:dbl)
                n349 = Add(x=w685, y=w695) -> (x+y=w689:dbl)
                n350 = Add(x=w686, y=w694) -> (x+y=w690:dbl)
                n351 = Replace Array Subset(array=w696, new element=w689, index (row)=w688, index (col)=w687) -> (w691:dbl[][])
                n352 = Replace Array Subset(array=w693, new element=w690, index (row)=w688, index (col)=w687) -> (w692:dbl[][])
              }
              n353 = for {
                tunnel: w616 -> [w676] mode=indexing
                tunnel: w615 -> [w675] mode=indexing
                tunnel: w618 -> [w673] mode=indexing
                tunnel: w617 -> [w674] mode=indexing
                shift-right: [w679] -> w554
                shift-left: w583 -> [w684]
                shift-right: [w680] -> w556
                shift-left: w583 -> [w681]
                n354 = Index Array(array=w684, index (row)=w676, index (col)=w675) -> (element=w683:dbl)
                n355 = Index Array(array=w681, index (row)=w676, index (col)=w675) -> (element=w682:dbl)
                n356 = Add(x=w673, y=w683) -> (x+y=w677:dbl)
                n357 = Add(x=w674, y=w682) -> (x+y=w678:dbl)
                n358 = Replace Array Subset(array=w684, new element=w677, index (row)=w676, index (col)=w675) -> (w679:dbl[][])
                n359 = Replace Array Subset(array=w681, new element=w678, index (row)=w676, index (col)=w675) -> (w680:dbl[][])
              }
              n360 = for {
                tunnel: w607 -> [w664] mode=indexing
                tunnel: w608 -> [w663] mode=indexing
                tunnel: w609 -> [w661] mode=indexing
                tunnel: w610 -> [w662] mode=indexing
                shift-right: [w667] -> w589
                shift-left: w586 -> [w672]
                shift-right: [w668] -> w590
                shift-left: w586 -> [w669]
                n361 = Index Array(array=w672, index (row)=w664, index (col)=w663) -> (element=w671:dbl)
                n362 = Index Array(array=w669, index (row)=w664, index (col)=w663) -> (element=w670:dbl)
                n363 = Add(x=w661, y=w671) -> (x+y=w665:dbl)
                n364 = Add(x=w662, y=w670) -> (x+y=w666:dbl)
                n365 = Replace Array Subset(array=w672, new element=w665, index (row)=w664, index (col)=w663) -> (w667:dbl[][])
                n366 = Replace Array Subset(array=w669, new element=w666, index (row)=w664, index (col)=w663) -> (w668:dbl[][])
              }
              n367 = for {
                tunnel: w613 -> [w652] mode=indexing
                tunnel: w614 -> [w651] mode=indexing
                tunnel: w611 -> [w649] mode=indexing
                tunnel: w612 -> [w650] mode=indexing
                shift-right: [w655] -> w595
                shift-left: w586 -> [w660]
                shift-right: [w656] -> w596
                shift-left: w586 -> [w657]
                n368 = Index Array(array=w660, index (row)=w652, index (col)=w651) -> (element=w659:dbl)
                n369 = Index Array(array=w657, index (row)=w652, index (col)=w651) -> (element=w658:dbl)
                n370 = Add(x=w649, y=w659) -> (x+y=w653:dbl)
                n371 = Add(x=w650, y=w658) -> (x+y=w654:dbl)
                n372 = Replace Array Subset(array=w660, new element=w653, index (row)=w652, index (col)=w651) -> (w655:dbl[][])
                n373 = Replace Array Subset(array=w657, new element=w654, index (row)=w652, index (col)=w651) -> (w656:dbl[][])
              }
              n374 = Greater?(x=w558, y=0) -> (0:w577:bool[][])
              n375 = Greater?(x=w572, y=0) -> (0:w574:bool[][])
              n376 = Boolean To (0,1)(Boolean=w577) -> (0, 1=w576:i16[][])
              n377 = Boolean To (0,1)(Boolean=w574) -> (0, 1=w573:i16[][])
              n378 = Multiply(x=w558, y=w576) -> (x*y=w562:dbl[][])
              n379 = Multiply(x=w572, y=w573) -> (x*y=w571:dbl[][])
              n380 = Equal To 0?(x=w562) -> (x = 0?=w626:bool[][])
              n381 = Equal To 0?(x=w571) -> (x = 0?=w603:bool[][])
              n382 = Boolean To (0,1)(Boolean=w626) -> (0, 1=w625:i16[][])
              n383 = Boolean To (0,1)(Boolean=w603) -> (0, 1=w604:i16[][])
              n384 = case shown="True" "Subtract Background?" {
                tunnel: w554 -> [_ w648]
                tunnel: w556 -> [_ w647]
                tunnel: w561 -> [w642 w646]
                tunnel: w560 -> [w641 w645]
                tunnel: [w642 w644] -> w550
                tunnel: [w641 w643] -> w551
                frame False {
                }
                frame True {
                  n385 = Subtract(x=w646, y=w648) -> (x-y=w644:dbl[][])
                  n386 = Subtract(x=w645, y=w647) -> (x-y=w643:dbl[][])
                }
              }
              n387 = case shown="True" "Subtract Background?" {
                tunnel: w596 -> [_ w640]
                tunnel: w595 -> [_ w639]
                tunnel: w590 -> [w633 w638]
                tunnel: w589 -> [w634 w637]
                tunnel: [w634 w636] -> w544
                tunnel: [w633 w635] -> w543
                frame False {
                }
                frame True {
                  n388 = Subtract(x=w637, y=w639) -> (x-y=w636:dbl[][])
                  n389 = Subtract(x=w638, y=w640) -> (x-y=w635:dbl[][])
                }
              }
              n390 = Multiply(x=w625, y=1e-06) -> (x*y=w623:dbl[][])
              n391 = Multiply(x=w604, y=1e-06) -> (x*y=w606:dbl[][])
              n392 = Add(x=w562, y=w623) -> (x+y=w549:dbl[][])
              n393 = Add(x=w571, y=w606) -> (x+y=w542:dbl[][])
              n394 = Divide(x=w550, y=w549) -> (x/y=w546:dbl[][])
              n395 = Divide(x=w551, y=w549) -> (x/y=w545:dbl[][])
              n396 = Divide(x=w544, y=w542) -> (x/y=w548:dbl[][])
              n397 = Divide(x=w543, y=w542) -> (x/y=w547:dbl[][])
            }
          }
          n398 = Subtract(x=w527, y=w529) -> (x-y=w525:dbl[][])
          n399 = Subtract(x=w526, y=w528) -> (x-y=w524:dbl[][])
          n400 = Absolute Value(x=w525) -> (abs(x)=w537:dbl[][])
          n401 = Absolute Value(x=w524) -> (abs(x)=w538:dbl[][])
          n402 = Greater?(x=w537, y="Centroid shift bound (pixels)") -> (0:w533:bool[][])
          n403 = Greater?(x=w538, y="Centroid shift bound (pixels)") -> (0:w530:bool[][])
          n404 = Not(x=w533) -> (.not. x?=w534:bool[][])
          n405 = Not(x=w530) -> (.not. x?=w531:bool[][])
          n406 = Boolean To (0,1)(Boolean=w534) -> (0, 1=w535:i16[][])
          n407 = Boolean To (0,1)(Boolean=w531) -> (0, 1=w532:i16[][])
          n408 = Multiply(x=w535, y=w525) -> (x*y=→"Shift kx":dbl[][])
          n409 = Multiply(x=w532, y=w524) -> (x*y=→"Shift ky":dbl[][])
        }
        frame #3 {
          # "Recovering the phase from the phase gradient"
          n410 = flat-sequence {
            frame #0 {
              w697 = 5.5e-05
              n411 = local read "Shift ky"() -> (w713:dbl[][])
              n412 = local read "Shift kx"() -> (w714:dbl[][])
              n413 = Multiply(x=w713, y=w697) -> (x*y=w709:dbl[][])
              n414 = Multiply(x=w714, y=w697) -> (x*y=w706:dbl[][])
              n415 = Multiply(x=w709, y=37.0 ("x")) -> (x*y=w708:dbl[][])
              n416 = Divide(x=w708, y="focal length (m)") -> (x/y=w711:dbl[][])
              n417 = Multiply(x=w706, y="Magnification") -> (x*y=w705:dbl[][])
              n418 = for {
                tunnel: w711 -> [w756] mode=indexing
                tunnel: [w754] -> w716 mode=indexing
                w755 = u16 0 items=["2nd Order Central", "4th Order Central", "Forward", "Backward"] ("method")
                n419 = call <vilib>:"Derivative x(t).vi"("method"=w755, "dt"=5.5e-05, "X"=w756) -> ("dX/dt"=w754:dbl[])  [unwired: 7 in, 1 out]
              }
              n420 = Divide(x=w705, y="focal length (m)") -> (x/y=w710:dbl[][])
              n421 = call-poly <vilib>:"FFT.vi"("shift?"=TRUE, "X"=w711) -> ("FFT {X}"=w744:cdb[][])  [unwired: 8 in, 1 out]
              n422 = Transpose 2D Array(2D array=w710) -> (transposed array=w715:dbl[][])
              n423 = Array Size(array=w710) -> (size(s)=w746:i32[])
              n424 = for {
                tunnel: w715 -> [w760] mode=indexing
                tunnel: [w759] -> w718 mode=indexing
                w758 = u16 0 items=["2nd Order Central", "4th Order Central", "Forward", "Backward"] ("method")
                n425 = call <vilib>:"Derivative x(t).vi"("method"=w758, "dt"=5.5e-05, "X"=w760) -> ("dX/dt"=w759:dbl[])  [unwired: 7 in, 1 out]
              }
              n426 = Array Max & Min(array=w746) -> (max value=w745:i32)  [unwired: 3 out]
              n427 = for {
                N: w745 -> [w761]
                tunnel: [w762] -> w750 mode=indexing
                n428 = for {
                  N: w761 -> [_]
                  tunnel: [w763] -> w762 mode=indexing
                  i -> [w764]
                  n429 = Increment(x=w764) -> (x+1=w763:i32)
                }
              }
              n430 = Divide(x=w745, y=2) -> (x/y=w748:dbl)
              n431 = Divide(x="Beam Diameter (mm)\n4 sigma", y=1000.0) -> (x/y=w751:dbl)
              n432 = Reciprocal(x=w751) -> (1/x=w752:dbl)
              n433 = Subtract(x=w750, y=w748) -> (x-y=w747:dbl[][])
              n434 = Transpose 2D Array(2D array=w718) -> (transposed array=w717:dbl[][])
              n435 = Multiply(x=w752, y=w747) -> (x*y=w712:dbl[][])
              n436 = Add(x=w717, y=w716) -> (x+y=→"Poisson":dbl[][])
              n437 = Equal To 0?(x=w712) -> (x = 0?=w734:bool[][])
              n438 = Boolean To (0,1)(Boolean=w734) -> (0, 1=w733:i16[][])
              n439 = Multiply(x=1e-06, y=w733) -> (x*y=w732:dbl[][])
              n440 = Add(x=w712, y=w732) -> (x+y=w741:dbl[][])
              n441 = call-poly <vilib>:"FFT.vi"("shift?"=TRUE, "X"=w710) -> ("FFT {X}"=w743:cdb[][])  [unwired: 8 in, 1 out]
              n442 = Multiply(x=w744, y=w741) -> (x*y=w738:cdb[][])
              n443 = Transpose 2D Array(2D array=w741) -> (transposed array=w742:dbl[][])
              n444 = Square(x=w742) -> (x^2=w740:dbl[][])
              n445 = Square(x=w741) -> (x^2=w739:dbl[][])
              n446 = Multiply(x=w743, y=w742) -> (x*y=w737:cdb[][])
              n447 = Add(x=w738, y=w737) -> (x+y=w736:cdb[][])
              n448 = Add(x=w740, y=w739) -> (x+y=w735:dbl[][])
              n449 = Divide(x=w736, y=w735) -> (x/y=w731:cdb[][])
              n450 = Multiply(x=cdb 0.0-1.0i, y=w731) -> (x*y=w703:cdb[][])
              n451 = call-poly <vilib>:"Inverse FFT.vi"("shift?"=TRUE, "FFT {X}"=w703) -> ("X"=w723:dbl[][])  [unwired: 8 in, 1 out]
              n452 = Complex To Re/Im(x + iy=w723) -> (x=w720:dbl[][])  [unwired: 1 out]
              n453 = Divide(x=6.283185307179586, y=8.1e-07) -> (x/y=w719:dbl)
              n454 = Multiply(x=w720, y=w719) -> (x*y=w702:dbl[][])
              n455 = Divide(x=w702, y=3.141592653589793) -> (x/y=→"Phase":dbl[][])
            }
          }
        }
      }
    }
  }
  n456 = call "Intensity Color Tables.vi"("Map Selector"=T6."gray") -> ("Color Map Array"=w1:u32[])
  n457 = property on="Phase" class="IntGraph (strict)"("Color Table"=w1) -> ()  [unwired: 2 in, 2 out]
  n458 = property on="Signal" class="IntGraph (strict)"("Color Table"=w1) -> ()  [unwired: 2 in, 2 out]
  n459 = property on="Idler" class="IntGraph (strict)"("Color Table"=w1) -> ()  [unwired: 2 in, 2 out]
